vi "MCBJ_IETS_07_2021.vi"() -> ()   [LabVIEW 2016]
uses:
  sub_vi_folder/for autom measure somehowControl 2.ctl
  LUCI-10/_TypeDefs/Choose_Device_Enum.ctl
  <vilib>/Instr/_visa.llb/VISA Configure Serial Port (Instr).vi
  Instance           4 28Saved   motor control w IETS .vi
  Stanford Research 830/Stanford Research 830.lvlib
  Agilent 34401/Agilent 34401.lvlib
  Lake Shore Cryotronics 331/Lake Shore Cryotronics 331.lvlib
  Agilent 3446X Series/Agilent 3446X Series.lvlib
  <vilib>/Analysis/NI_AALBase.lvlib
  Keithley DMM6500 DAQ6500 Series/Keithley DMM6500 DAQ6500 Series.lvlib
  LUCI-10/FEMTO_LUCI-10.lvlib
panel:
  out "High R mode":bool=TRUE
  in  "lockin_once":bool
  out "LIA_all":dbl=3.282477411892588e-08
  out "# IV Curves":u16=101
  out "# O/C Cycles":u16=163
  out "LIA_conductance":dbl=3.282477414397079e-08
  out "R_Ohm_LIA1":dbl=2047762829745.1099
  out "CA gain":dbl=1e-11
  out "Femto_gain":T1(ring)=enum."10^11"
  out "Temp B in K":dbl=16.442 min=0.0 max=1645.0 step=1e-05 format="%^.5e"
  out "Temp. A in K":dbl=6.222 min=0.0 max=1645.0 step=1e-05 format="%^.5e"
  out "Bias_meas":dbl=0.028463005
  out "LIA2_DMM":dbl=0.171521931
  out "LIA1_DMM":dbl=0.0890152763
  in  "Set Lockin":bool
  in  "IETS":bool
  out "G in G0":dbl=6.3026848342087415e-09 format="%#_3g"
  out "Volt drop":dbl=0.001389956
  out "x LIA 1":dbl=0.00285722
  out "X LIA 2":dbl=-0.000922445
  out "delt MP Reached":bool
  out "Low R Mode":bool
  in  "Measurement":bool
  out "IV Active":bool
  in  "IV Sweep":bool
  in  "Stop":bool
  out "# Data Points":u32=663713
  out "R [Ohm]":dbl=2047763022414.3882 format="%#_3g"
  out "Motor Position":i32=-244174520 format="%#.3e"
  out "Reference Velocity":i16=1500
  out "Effective Velocity":i32=1499
  out "Open / Close":bool
  in  "Path Data Files":path=path "D:/MCBJ_DATA/IETS_new programm/ganz neu/S5_2021/c60/Evap_5/21_06_2021/0/322_5Hz_new_mot"
  in  "Tab":T2(tab)
  in  "Opening Velocity (High R)":i16=-1000
  in  "Closing  Velocity (High R)":i16=1500
  in  "switch Res Min [Ohm]":dbl=1000.0
  in  "reverse direction":bool
  in  "Min. R (Delta MP)  [Ohm]":dbl=4000.0
  in  "Switch by Motor Position Overrides other Switch Modes":bool
  in  "Delta Motor Position [counts]":i32=-50000000 format="%#.3e"
  in  "Opening Start Resistance [Ohm]":dbl=14906.0 format="%#.3f"
  in  "High -Low Resistance Velocity Mode":bool=TRUE
  in  "Max. Motor Position [counts]":i32=400000000 format="%#.3e"
  in  "Min. Motor Position [counts]":i32=-300000000 format="%#.3e"
  in  "Closing Velocity (Low R)":i16=1000
  in  "Opening Velocity (Low R)":i16=-2000
  in  "Use Motor":bool=TRUE
  in  "Closing Vel":i16=400
  in  "Opening opening Vel":i16=-2500
  in  "Max. Resistance [Ohm]":dbl=5000000000.0 format="%^#_6e"
  in  "Min. Resistance [Ohm]":dbl=120000.0
  in  "O/C Switch Mode":T3(radio)
  in  "Switch Res_Max. [Ohm]":dbl=100000000.0
  in  "Minimum Limit [counts]":i32=-2000000000 format="%#.3e"
  in  "Maximum Limit [counts]":i32=300000000 format="%#.3e"
  in  "Save load":u16(ring) items=["Save", "Recall"]
  in  "Setup Num":dbl=1.0
  in  "Cont Stor":bool=TRUE
  in  "Grounding":u16(ring)=1 items=["Float", "Ground"]
  in  "Sample Rate":u16(ring)=11 items=["62.5 mHz", "125 mHz", "250 mHz", "500 mHz", "1 Hz", "2 Hz", "4 Hz", "8Hz", "16 Hz", "32 Hz", "64 Hz", "128 Hz", "256 Hz", "512 Hz", "Trigger "]
  in  "In Coupling":u16(ring) items=["AC", "DC"]
  in  "Notch":u16(ring) items=["None", "Line Notch", "2x Line Notch", "Both Notch Filters"]
  in  "Input":u16(ring) items=["Single-Ended Voltage", "Differential Voltage", "1 MOhm Current Gain", "100 MOhm Current Gain"]
  in  "Ext  Trigger":u16(ring)=1 items=["Sine Zero Crossing", "TTL Rising Edge", "TTL Falling Edge"]
  in  "wait bias":u32=1
  in  "res 34401":dbl=1.0 format="%_3f"
  in  "talk 34401":bool
  in  "Line Sync":bool
  in  "rang OC (V)":dbl=2.0 format="%_3f"
  in  "Auto Range":bool=TRUE
  in  "AutoZ":bool=TRUE
  in  "Sensitivity 2":dbl=0.1
  in  "Sensitivity":dbl=0.1
  in  "LIA exp 1":dbl=1.0
  in  "LIA exp 2":dbl=100.0
  in  "Input Z":i32(ring) items=["10Mohm", "Auto"]
  in  "Av. F. Type":i32(ring)=1 items=["Repeat", "Moving"]
  in  "F. Count":u32=10
  in  "Average F.":bool
  in  "Fi. Window":dbl
  in  "AC Filter":i32(ring)=3 items=["3"=3, "20"=20, "200"=200]
  in  "Display":i32(ring) items=["Home Screen", "Home with Large Readings", "Reading Table", "Graph", "Functions Swipe", "Graph Swipe", "Secondary Swipe", "Setting Swipe", "Statistic Swipe", "User Swipe", "Channel Swipe", "Nonswitch Swipe", "Scan Swipe", "Control Channel", "Settings Channel", "Scan Channel"]
  in  "CA gain (man)":dbl=0.0001
  in  "Harm":dbl=2.0
  in  "Expand LIA1":u16(ring) items=["x1", "x10", "x100"]
  in  "Expand LIA2":u16(ring)=2 items=["x1", "x10", "x100"]
  in  "Dyn Reserve LIA1":i16(ring)=1 items=["Auto Reserve"=-1, "High Reserve"=0, "Normal"=1, "Low Noise"=2]
  in  "Dyn Reserve  LIA2":i16(ring)=1 items=["Auto Reserve"=-1, "High Reserve"=0, "Normal"=1, "Low Noise"=2]
  in  "Sensitivity LIA1":i16(ring)=23 items=["Auto Gain"=-1, "2 nV/fA"=0, "5 nV/fA"=1, "10 nV/fA"=2, "20 nV/fA"=3, "50 nV/fA"=4, "100 nV/fA"=5, "200 nV/fA"=6, "500 nV/fA"=7, "1 uV/pA"=8, "2 uV/pA"=9, "5 uV/pA"=10, "10 uV/pA"=11, "20 uV/pA"=12, "50 uV/pA"=13, "100 uV/pA"=14, "200 uV/pA"=15, "500 uV/pA"=16, "1 mV/nA"=17, "2 mV/nA"=18, "5 mV/nA"=19, "10 mV/nA"=20, "20 mV/nA"=21, "50 mV/nA"=22, "100 mV/nA"=23, "200 mV/nA"=24, "500 mV/mA"=25, "1 V/uA"=26]
  in  "Sensitivity LIA2":i16(ring)=23 items=["Auto Gain"=-1, "2 nV/fA"=0, "5 nV/fA"=1, "10 nV/fA"=2, "20 nV/fA"=3, "50 nV/fA"=4, "100 nV/fA"=5, "200 nV/fA"=6, "500 nV/fA"=7, "1 uV/pA"=8, "2 uV/pA"=9, "5 uV/pA"=10, "10 uV/pA"=11, "20 uV/pA"=12, "50 uV/pA"=13, "100 uV/pA"=14, "200 uV/pA"=15, "500 uV/pA"=16, "1 mV/nA"=17, "2 mV/nA"=18, "5 mV/nA"=19, "10 mV/nA"=20, "20 mV/nA"=21, "50 mV/nA"=22, "100 mV/nA"=23, "200 mV/nA"=24, "500 mV/mA"=25, "1 V/uA"=26]
  in  "LP_timeLIA2":u16(ring)=9 items=["10 us", "30 us", "100 us", "300 us", "1 ms", "3 ms", "10 ms", "30 ms", "100 ms", "300 ms", "1 s", "3 s", "10 s", "30 s", "100 s", "300 s", "1 ks", "3 ks", "10 ks", "30 ks"]
  in  "LP_timeLIA1":u16(ring)=9 items=["10 us", "30 us", "100 us", "300 us", "1 ms", "3 ms", "10 ms", "30 ms", "100 ms", "300 ms", "1 s", "3 s", "10 s", "30 s", "100 s", "300 s", "1 ks", "3 ks", "10 ks", "30 ks"]
  in  "LP_slope_ LIA1":u16(ring) items=["6 dB/oct", "12 dB/oct", "18 db/oct", "24 dB/oct"]
  in  "LP Slope LIA2":u16(ring) items=["6 dB/oct", "12 dB/oct", "18 db/oct", "24 dB/oct"]
  in  "Frequency":dbl=322.5
  in  "Auto Pha  LIA2":bool
  in  "Auto Phase":bool
  in  "S OutpAmpl":dbl=0.35
  in  "Man Phase LIA1":dbl
  in  "man phase LIA2":dbl=90.0
  in  "Int. Time":dbl(ring)=1.0 items=["0.001"=0.001, "0.002"=0.002, "0.006"=0.006, "0.02"=0.02, "0.06"=0.06, "0.2"=0.2, "1"=1.0, "10"=10.0, "100"=100.0]
  in  "wait points":i16=2500
  in  "Max.  [Ohm]":dbl=105000000.0 format="%^#_6e"
  in  "Min.  [Ohm]":dbl=50000.0 format="%^#_6e"
  in  "IV Delay [ms]":u16=4500
  in  "Initail V":dbl=0.3
  in  "Final V":dbl=-0.3
  in  "Set0 step":dbl=0.002 format="%#.6g"
  in  "Step (V)":dbl=0.001
  in  "Bias Voltage OC":dbl=0.1
  in  "Pre-R [Ohm]":dbl=300.0
  in  "# IV  Loops":u16=1
  in  "Use_femto":bool=TRUE
  out "Overload":bool
  in  "Bias_polarity":bool=TRUE
  in  "LIA_G":bool
  in  "Yoko_Range":T4(ring)=enum."1V"
  out "Resistance / time graph":dbl(graph)=2047763022414.3882
  out "R_Ohm_Vdrop":dbl=102.57700425624137
  out "Sample Conductance (Main)":dbl(graph)=6.3026848342087415e-09
  in  "amp_very_high_gain":dbl=0.35
  in  "?":bool
  out "no IV":bool=TRUE
  out "XY Graph   3":cluster{"x":dbl, "y":dbl}[](graph)=[{"x"=0.30282192, "y"=0.0005515354698005646}, {"x"=0.30282192, "y"=0.0005515354698005646}, {"x"=0.30282192, "y"=0.0005515354698005646}, {"x"=0.30282192, "y"=0.0005515354698005646}, {"x"=0.30282192, "y"=0.0005515354698005646}, {"x"=0.30282192, "y"=0.0005515354698005646}, {"x"=0.30282192, "y"=0.0005515354698005646}, {"x"=0.30282192, "y"=0.0005515354698005646}, {"x"=0.30282192, "y"=0.0005515354698005646}, {"x"=0.30282192, "y"=0.0005515354698005646}, {"x"=0.30282192, "y"=0.0005515354698005646}, {"x"=0.30282192, "y"=0.0005515354698005646}, {"x"=0.30282192, "y"=0.0005515354698005646}, {"x"=0.30282192, "y"=0.0005515354698005646}, {"x"=0.30282192, "y"=0.0005515354698005646}, {"x"=0.30282192, "y"=0.0005515354698005646}, {"x"=0.30282192, "y"=0.0005515354698005646}, {"x"=0.30282192, "y"=0.0005515354698005646}, {"x"=0.30282192, "y"=0.0005515354698005646}, {"x"=0.30282192, "y"=0.0005515354698005646}, {"x"=0.30282192, "y"=0.0005515354698005646}, {"x"=0.30282192, "y"=0.0005515354698005646}, {"x"=0.30282192, "y"=0.0005515354698005646}, {"x"=0.30282192, "y"=0.0005515354698005646}, {"x"=0.30282192, "y"=0.0005515354698005646}, {"x"=0.30282192, "y"=0.0005515354698005646}, {"x"=0.30282192, "y"=0.0005515354698005646}, {"x"=0.30282192, "y"=0.0005515354698005646}, {"x"=0.30282192, "y"=0.0005515354698005646}, {"x"=0.30282192, "y"=0.0005515354698005646}, {"x"=0.30282192, "y"=0.0005515354698005646}, {"x"=0.30282192, "y"=0.0005515354698005646}, {"x"=0.30282192, "y"=0.0005515354698005646}, {"x"=0.30282192, "y"=0.0005515354698005646}, {"x"=0.30282192, "y"=0.0005515354698005646}, {"x"=0.30282192, "y"=0.0005515354698005646}, {"x"=0.30282192, "y"=0.0005515354698005646}, {"x"=0.30282192, "y"=0.0005515354698005646}, {"x"=0.30282192, "y"=0.0005515354698005646}, {"x"=0.30282192, "y"=0.0005515354698005646}, {"x"=0.30282192, "y"=0.0005515354698005646}, {"x"=0.30282192, "y"=0.0005515354698005646}, {"x"=0.30282192, "y"=0.0005515354698005646}, {"x"=0.30282192, "y"=0.0005515354698005646}, {"x"=0.30282192, "y"=0.0005515354698005646}, {"x"=0.30282192, "y"=0.0005515354698005646}, {"x"=0.30282192, "y"=0.0005515354698005646}, {"x"=0.30282192, "y"=0.0005515354698005646}, {"x"=0.30282192, "y"=0.0005515354698005646}, {"x"=0.30282192, "y"=0.0005515354698005646}, {"x"=0.30282192, "y"=0.0005515354698005646}, {"x"=0.30282192, "y"=0.0005515354698005646}, {"x"=0.30282192, "y"=0.0005515354698005646}, {"x"=0.30282192, "y"=0.0005515354698005646}, {"x"=0.30282192, "y"=0.0005515354698005646}, {"x"=0.30282192, "y"=0.0005515354698005646}, {"x"=0.30282192, "y"=0.0005515354698005646}, {"x"=0.30282192, "y"=0.0005515354698005646}, {"x"=0.30282192, "y"=0.0005515354698005646}, {"x"=0.30282192, "y"=0.0005515354698005646}, {"x"=0.30282192, "y"=0.0005515354698005646}, {"x"=0.30282192, "y"=0.0005515354698005646}, {"x"=0.30282192, "y"=0.0005515354698005646}, {"x"=0.30282192, "y"=0.0005515354698005646}, {"x"=0.30282192, "y"=0.0005515354698005646}, {"x"=0.30282192, "y"=0.0005515354698005646}, {"x"=0.30282192, "y"=0.0005515354698005646}, {"x"=0.30282192, "y"=0.0005515354698005646}, {"x"=0.30282192, "y"=0.0005515354698005646}, {"x"=0.30282192, "y"=0.0005515354698005646}, {"x"=0.30282192, "y"=0.0005515354698005646}, {"x"=0.30282192, "y"=0.0005515354698005646}, {"x"=0.30282192, "y"=0.0005515354698005646}, {"x"=0.30282192, "y"=0.0005515354698005646}, {"x"=0.30282192, "y"=0.0005515354698005646}, {"x"=0.30282192, "y"=0.0005515354698005646}, {"x"=0.30282192, "y"=0.0005515354698005646}, {"x"=0.30282192, "y"=0.0005515354698005646}, {"x"=0.30282192, "y"=0.0005515354698005646}, {"x"=0.30282192, "y"=0.0005515354698005646}, {"x"=0.30282192, "y"=0.0005515354698005646}, {"x"=0.30282192, "y"=0.0005515354698005646}, {"x"=0.30282192, "y"=0.0005515354698005646}, {"x"=0.30282192, "y"=0.0005515354698005646}, {"x"=0.30282192, "y"=0.0005515354698005646}, {"x"=0.30282192, "y"=0.0005515354698005646}, {"x"=0.30282192, "y"=0.0005515354698005646}, {"x"=0.30282192, "y"=0.0005515354698005646}, {"x"=0.30282192, "y"=0.0005515354698005646}, {"x"=0.30282192, "y"=0.0005515354698005646}, {"x"=0.30282192, "y"=0.0005515354698005646}, {"x"=0.30282192, "y"=0.0005515354698005646}, {"x"=0.30282192, "y"=0.0005515354698005646}, {"x"=0.30282192, "y"=0.0005515354698005646}, {"x"=0.30282192, "y"=0.0005515354698005646}, {"x"=0.30282192, "y"=0.0005515354698005646}, {"x"=0.30282192, "y"=0.0005515354698005646}, {"x"=0.30282192, "y"=0.0005515354698005646}, {"x"=0.30282192, "y"=0.0005515354698005646}, {"x"=0.30282192, "y"=0.0005515354698005646}, {"x"=0.30282192, "y"=0.0005515354698005646}, {"x"=0.30282192, "y"=0.0005515354698005646}, {"x"=0.30282192, "y"=0.0005515354698005646}, {"x"=0.30282192, "y"=0.0005515354698005646}, {"x"=0.30282192, "y"=0.0005515354698005646}, {"x"=0.30282192, "y"=0.0005515354698005646}, {"x"=0.30282192, "y"=0.0005515354698005646}, {"x"=0.30282192, "y"=0.0005515354698005646}, {"x"=0.30282192, "y"=0.0005515354698005646}, {"x"=0.30282192, "y"=0.0005515354698005646}, {"x"=0.30282192, "y"=0.0005515354698005646}, {"x"=0.30282192, "y"=0.0005515354698005646}, {"x"=0.30282192, "y"=0.0005515354698005646}, {"x"=0.30282192, "y"=0.0005515354698005646}, {"x"=0.30282192, "y"=0.0005515354698005646}, {"x"=0.30282192, "y"=0.0005515354698005646}, {"x"=0.30282192, "y"=0.0005515354698005646}, {"x"=0.30282192, "y"=0.0005515354698005646}, {"x"=0.30282192, "y"=0.0005515354698005646}, {"x"=0.30282192, "y"=0.0005515354698005646}, {"x"=0.30282192, "y"=0.0005515354698005646}, {"x"=0.30282192, "y"=0.0005515354698005646}, {"x"=0.30282192, "y"=0.0005515354698005646}, {"x"=0.30282192, "y"=0.0005515354698005646}, {"x"=0.30282192, "y"=0.0005515354698005646}, {"x"=0.30282192, "y"=0.0005515354698005646}, {"x"=0.30282192, "y"=0.0005515354698005646}, {"x"=0.30282192, "y"=0.0005515354698005646}, {"x"=0.30282192, "y"=0.0005515354698005646}, {"x"=0.30282192, "y"=0.0005515354698005646}, {"x"=0.30282192, "y"=0.0005515354698005646}, {"x"=0.30282192, "y"=0.0005515354698005646}, {"x"=0.30282192, "y"=0.0005515354698005646}, {"x"=0.30282192, "y"=0.0005515354698005646}, {"x"=0.30282192, "y"=0.0005515354698005646}, {"x"=0.30282192, "y"=0.0005515354698005646}, {"x"=0.30282192, "y"=0.0005515354698005646}, {"x"=0.30282192, "y"=0.0005515354698005646}, {"x"=0.30282192, "y"=0.0005515354698005646}, {"x"=0.30282192, "y"=0.0005515354698005646}, {"x"=0.30282192, "y"=0.0005515354698005646}, {"x"=0.30282192, "y"=0.0005515354698005646}, {"x"=0.30282192, "y"=0.0005515354698005646}, {"x"=0.30282192, "y"=0.0005515354698005646}, {"x"=0.30282192, "y"=0.0005515354698005646}, {"x"=0.30282192, "y"=0.0005515354698005646}, {"x"=0.30282192, "y"=0.0005515354698005646}, {"x"=0.30282192, "y"=0.0005515354698005646}, {"x"=0.30282192, "y"=0.0005515354698005646}, {"x"=0.30282192, "y"=0.0005515354698005646}, {"x"=0.30282192, "y"=0.0005515354698005646}, {"x"=0.30282192, "y"=0.0005515354698005646}, {"x"=0.30282192, "y"=0.0005515354698005646}, {"x"=0.30282192, "y"=0.0005515354698005646}, {"x"=0.30282192, "y"=0.0005515354698005646}, {"x"=0.30282192, "y"=0.0005515354698005646}, {"x"=0.30282192, "y"=0.0005515354698005646}, {"x"=0.30282192, "y"=0.0005515354698005646}, {"x"=0.30282192, "y"=0.0005515354698005646}, {"x"=0.30282192, "y"=0.0005515354698005646}, {"x"=0.30282192, "y"=0.0005515354698005646}, {"x"=0.30282192, "y"=0.0005515354698005646}, {"x"=0.30282192, "y"=0.0005515354698005646}, {"x"=0.30282192, "y"=0.0005515354698005646}, {"x"=0.30282192, "y"=0.0005515354698005646}, {"x"=0.30282192, "y"=0.0005515354698005646}, {"x"=0.30282192, "y"=0.0005515354698005646}, {"x"=0.30282192, "y"=0.0005515354698005646}, {"x"=0.30282192, "y"=0.0005515354698005646}, {"x"=0.30282192, "y"=0.0005515354698005646}, {"x"=0.30282192, "y"=0.0005515354698005646}, {"x"=0.30282192, "y"=0.0005515354698005646}, {"x"=0.30282192, "y"=0.0005515354698005646}, {"x"=0.30282192, "y"=0.0005515354698005646}, {"x"=0.30282192, "y"=0.0005515354698005646}, {"x"=0.30282192, "y"=0.0005515354698005646}, {"x"=0.30282192, "y"=0.0005515354698005646}, {"x"=0.30282192, "y"=0.0005515354698005646}, {"x"=0.30282192, "y"=0.0005515354698005646}, {"x"=0.30282192, "y"=0.0005515354698005646}, {"x"=0.30282192, "y"=0.0005515354698005646}, {"x"=0.30282192, "y"=0.0005515354698005646}, {"x"=0.30282192, "y"=0.0005515354698005646}, {"x"=0.30282192, "y"=0.0005515354698005646}, {"x"=0.30282192, "y"=0.0005515354698005646}, {"x"=0.30282192, "y"=0.0005515354698005646}, {"x"=0.30282192, "y"=0.0005515354698005646}, {"x"=0.30282192, "y"=0.0005515354698005646}, {"x"=0.30282192, "y"=0.0005515354698005646}, {"x"=0.30282192, "y"=0.0005515354698005646}, {"x"=0.30282192, "y"=0.0005515354698005646}, {"x"=0.30282192, "y"=0.0005515354698005646}, {"x"=0.30282192, "y"=0.0005515354698005646}, {"x"=0.30282192, "y"=0.0005515354698005646}, {"x"=0.30282192, "y"=0.0005515354698005646}, {"x"=0.30282192, "y"=0.0005515354698005646}, {"x"=0.30282192, "y"=0.0005515354698005646}, {"x"=0.30282192, "y"=0.0005515354698005646}, {"x"=0.30282192, "y"=0.0005515354698005646}, {"x"=0.30282192, "y"=0.0005515354698005646}, {"x"=0.30282192, "y"=0.0005515354698005646}, {"x"=0.30282192, "y"=0.0005515354698005646}, {"x"=0.30282192, "y"=0.0005515354698005646}, {"x"=0.30282192, "y"=0.0005515354698005646}, {"x"=0.30282192, "y"=0.0005515354698005646}, {"x"=0.30282192, "y"=0.0005515354698005646}, {"x"=0.30282192, "y"=0.0005515354698005646}, {"x"=0.30282192, "y"=0.0005515354698005646}, {"x"=0.30282192, "y"=0.0005515354698005646}, {"x"=0.30282192, "y"=0.0005515354698005646}, {"x"=0.30282192, "y"=0.0005515354698005646}, {"x"=0.30282192, "y"=0.0005515354698005646}, {"x"=0.30282192, "y"=0.0005515354698005646}, {"x"=0.30282192, "y"=0.0005515354698005646}, {"x"=0.30282192, "y"=0.0005515354698005646}, {"x"=0.30282192, "y"=0.0005515354698005646}, {"x"=0.30282192, "y"=0.0005515354698005646}, {"x"=0.30282192, "y"=0.0005515354698005646}, {"x"=0.30282192, "y"=0.0005515354698005646}, {"x"=0.30282192, "y"=0.0005515354698005646}, {"x"=0.30282192, "y"=0.0005515354698005646}, {"x"=0.30282192, "y"=0.0005515354698005646}, {"x"=0.30282192, "y"=0.0005515354698005646}, {"x"=0.30282192, "y"=0.0005515354698005646}, {"x"=0.30282192, "y"=0.0005515354698005646}, {"x"=0.30282192, "y"=0.0005515354698005646}, {"x"=0.30282192, "y"=0.0005515354698005646}, {"x"=0.30282192, "y"=0.0005515354698005646}, {"x"=0.30282192, "y"=0.0005515354698005646}, {"x"=0.30282192, "y"=0.0005515354698005646}, {"x"=0.30282192, "y"=0.0005515354698005646}, {"x"=0.30282192, "y"=0.0005515354698005646}, {"x"=0.30282192, "y"=0.0005515354698005646}, {"x"=0.30282192, "y"=0.0005515354698005646}, {"x"=0.30282192, "y"=0.0005515354698005646}, {"x"=0.30282192, "y"=0.0005515354698005646}, {"x"=0.30282192, "y"=0.0005515354698005646}, {"x"=0.30282192, "y"=0.0005515354698005646}, {"x"=0.30282192, "y"=0.0005515354698005646}, {"x"=0.30282192, "y"=0.0005515354698005646}, {"x"=0.30282192, "y"=0.0005515354698005646}, {"x"=0.30282192, "y"=0.0005515354698005646}, {"x"=0.30282192, "y"=0.0005515354698005646}, {"x"=0.30282192, "y"=0.0005515354698005646}, {"x"=0.30282192, "y"=0.0005515354698005646}, {"x"=0.30282192, "y"=0.0005515354698005646}, {"x"=0.30282192, "y"=0.0005515354698005646}, {"x"=0.30282192, "y"=0.0005515354698005646}, {"x"=0.30282192, "y"=0.0005515354698005646}, {"x"=0.30282192, "y"=0.0005515354698005646}, {"x"=0.30282192, "y"=0.0005515354698005646}, {"x"=0.30282192, "y"=0.0005515354698005646}, {"x"=0.30282192, "y"=0.0005515354698005646}, {"x"=0.30282192, "y"=0.0005515354698005646}, {"x"=0.30282192, "y"=0.0005515354698005646}, {"x"=0.30282192, "y"=0.0005515354698005646}, {"x"=0.30282192, "y"=0.0005515354698005646}, {"x"=0.30282192, "y"=0.0005515354698005646}, {"x"=0.30282192, "y"=0.0005515354698005646}, {"x"=0.30282192, "y"=0.0005515354698005646}, {"x"=0.30282192, "y"=0.0005515354698005646}, {"x"=0.30282192, "y"=0.0005515354698005646}, {"x"=0.30282192, "y"=0.0005515354698005646}, {"x"=0.30282192, "y"=0.0005515354698005646}, {"x"=0.30282192, "y"=0.0005515354698005646}, {"x"=0.30282192, "y"=0.0005515354698005646}, {"x"=0.30282192, "y"=0.0005515354698005646}, {"x"=0.30282192, "y"=0.0005515354698005646}, {"x"=0.30282192, "y"=0.0005515354698005646}, {"x"=0.30282192, "y"=0.0005515354698005646}, {"x"=0.30282192, "y"=0.0005515354698005646}, {"x"=0.30282192, "y"=0.0005515354698005646}, {"x"=0.30282192, "y"=0.0005515354698005646}, {"x"=0.30282192, "y"=0.0005515354698005646}, {"x"=0.30282192, "y"=0.0005515354698005646}, {"x"=0.30282192, "y"=0.0005515354698005646}, {"x"=0.30282192, "y"=0.0005515354698005646}, {"x"=0.30282192, "y"=0.0005515354698005646}, {"x"=0.30282192, "y"=0.0005515354698005646}, {"x"=0.30282192, "y"=0.0005515354698005646}, {"x"=0.30282192, "y"=0.0005515354698005646}, {"x"=0.30282192, "y"=0.0005515354698005646}, {"x"=0.30282192, "y"=0.0005515354698005646}, {"x"=0.30282192, "y"=0.0005515354698005646}, {"x"=0.30282192, "y"=0.0005515354698005646}, {"x"=0.30282192, "y"=0.0005515354698005646}, {"x"=0.30282192, "y"=0.0005515354698005646}, {"x"=0.30282192, "y"=0.0005515354698005646}, {"x"=0.30282192, "y"=0.0005515354698005646}, {"x"=0.30282192, "y"=0.0005515354698005646}, {"x"=0.30282192, "y"=0.0005515354698005646}, {"x"=0.30282192, "y"=0.0005515354698005646}, {"x"=0.30282192, "y"=0.0005515354698005646}, {"x"=0.30282192, "y"=0.0005515354698005646}, {"x"=0.30282192, "y"=0.0005515354698005646}, {"x"=0.30282192, "y"=0.0005515354698005646}, {"x"=0.30282192, "y"=0.0005515354698005646}, {"x"=0.30282192, "y"=0.0005515354698005646}, {"x"=0.30282192, "y"=0.0005515354698005646}, {"x"=0.30282192, "y"=0.0005515354698005646}, {"x"=0.30282192, "y"=0.0005515354698005646}, {"x"=0.30282192, "y"=0.0005515354698005646}, {"x"=0.30282192, "y"=0.0005515354698005646}, {"x"=0.30282192, "y"=0.0005515354698005646}, {"x"=0.30282192, "y"=0.0005515354698005646}, {"x"=0.30282192, "y"=0.0005515354698005646}, {"x"=0.30282192, "y"=0.0005515354698005646}, {"x"=0.30282192, "y"=0.0005515354698005646}, {"x"=0.30282192, "y"=0.0005515354698005646}, {"x"=0.30282192, "y"=0.0005515354698005646}, {"x"=0.30282192, "y"=0.0005515354698005646}, {"x"=0.30282192, "y"=0.0005515354698005646}, {"x"=0.30282192, "y"=0.0005515354698005646}, {"x"=0.30282192, "y"=0.0005515354698005646}, {"x"=0.30282192, "y"=0.0005515354698005646}, {"x"=0.30282192, "y"=0.0005515354698005646}, {"x"=0.30282192, "y"=0.0005515354698005646}, {"x"=0.30282192, "y"=0.0005515354698005646}, {"x"=0.30282192, "y"=0.0005515354698005646}, {"x"=0.30282192, "y"=0.0005515354698005646}, {"x"=0.30282192, "y"=0.0005515354698005646}, {"x"=0.30282192, "y"=0.0005515354698005646}, {"x"=0.30282192, "y"=0.0005515354698005646}, {"x"=0.30282192, "y"=0.0005515354698005646}, {"x"=0.30282192, "y"=0.0005515354698005646}, {"x"=0.30282192, "y"=0.0005515354698005646}, {"x"=0.30282192, "y"=0.0005515354698005646}, {"x"=0.30282192, "y"=0.0005515354698005646}, {"x"=0.30282192, "y"=0.0005515354698005646}, {"x"=0.30282192, "y"=0.0005515354698005646}, {"x"=0.30282192, "y"=0.0005515354698005646}, {"x"=0.30282192, "y"=0.0005515354698005646}, {"x"=0.30282192, "y"=0.0005515354698005646}, {"x"=0.30282192, "y"=0.0005515354698005646}, {"x"=0.30282192, "y"=0.0005515354698005646}, {"x"=0.30282192, "y"=0.0005515354698005646}, {"x"=0.30282192, "y"=0.0005515354698005646}, {"x"=0.30282192, "y"=0.0005515354698005646}, {"x"=0.30282192, "y"=0.0005515354698005646}, {"x"=0.30282192, "y"=0.0005515354698005646}, {"x"=0.30282192, "y"=0.0005515354698005646}, {"x"=0.30282192, "y"=0.0005515354698005646}, {"x"=0.30282192, "y"=0.0005515354698005646}, {"x"=0.30282192, "y"=0.0005515354698005646}, {"x"=0.30282192, "y"=0.0005515354698005646}, {"x"=0.30282192, "y"=0.0005515354698005646}, {"x"=0.30282192, "y"=0.0005515354698005646}, {"x"=0.30282192, "y"=0.0005515354698005646}, {"x"=0.30282192, "y"=0.0005515354698005646}, {"x"=0.30282192, "y"=0.0005515354698005646}, {"x"=0.30282192, "y"=0.0005515354698005646}, {"x"=0.30282192, "y"=0.0005515354698005646}, {"x"=0.30282192, "y"=0.0005515354698005646}, {"x"=0.30282192, "y"=0.0005515354698005646}, {"x"=0.30282192, "y"=0.0005515354698005646}, {"x"=0.30282192, "y"=0.0005515354698005646}, {"x"=0.30282192, "y"=0.0005515354698005646}, {"x"=0.30282192, "y"=0.0005515354698005646}, {"x"=0.30282192, "y"=0.0005515354698005646}, {"x"=0.30282192, "y"=0.0005515354698005646}, {"x"=0.30282192, "y"=0.0005515354698005646}, {"x"=0.30282192, "y"=0.0005515354698005646}, {"x"=0.30282192, "y"=0.0005515354698005646}, {"x"=0.30282192, "y"=0.0005515354698005646}, {"x"=0.30282192, "y"=0.0005515354698005646}, {"x"=0.30282192, "y"=0.0005515354698005646}, {"x"=0.30282192, "y"=0.0005515354698005646}, {"x"=0.30282192, "y"=0.0005515354698005646}, {"x"=0.30282192, "y"=0.0005515354698005646}, {"x"=0.30282192, "y"=0.0005515354698005646}, {"x"=0.30282192, "y"=0.0005515354698005646}, {"x"=0.30282192, "y"=0.0005515354698005646}, {"x"=0.30282192, "y"=0.0005515354698005646}, {"x"=0.30282192, "y"=0.0005515354698005646}, {"x"=0.30282192, "y"=0.0005515354698005646}, {"x"=0.30282192, "y"=0.0005515354698005646}, {"x"=0.30282192, "y"=0.0005515354698005646}, {"x"=0.30282192, "y"=0.0005515354698005646}, {"x"=0.30282192, "y"=0.0005515354698005646}, {"x"=0.30282192, "y"=0.0005515354698005646}, {"x"=0.30282192, "y"=0.0005515354698005646}, {"x"=0.30282192, "y"=0.0005515354698005646}, {"x"=0.30282192, "y"=0.0005515354698005646}, {"x"=0.30282192, "y"=0.0005515354698005646}, {"x"=0.30282192, "y"=0.0005515354698005646}, {"x"=0.30282192, "y"=0.0005515354698005646}, {"x"=0.30282192, "y"=0.0005515354698005646}, {"x"=0.30282192, "y"=0.0005515354698005646}, {"x"=0.30282192, "y"=0.0005515354698005646}, {"x"=0.30282192, "y"=0.0005515354698005646}, {"x"=0.30282192, "y"=0.0005515354698005646}, {"x"=0.30282192, "y"=0.0005515354698005646}, {"x"=0.30282192, "y"=0.0005515354698005646}, {"x"=0.30282192, "y"=0.0005515354698005646}, {"x"=0.30282192, "y"=0.0005515354698005646}, {"x"=0.30282192, "y"=0.0005515354698005646}, {"x"=0.30282192, "y"=0.0005515354698005646}, {"x"=0.30282192, "y"=0.0005515354698005646}, {"x"=0.30282192, "y"=0.0005515354698005646}, {"x"=0.30282192, "y"=0.0005515354698005646}, {"x"=0.30282192, "y"=0.0005515354698005646}, {"x"=0.30282192, "y"=0.0005515354698005646}, {"x"=0.30282192, "y"=0.0005515354698005646}, {"x"=0.30282192, "y"=0.0005515354698005646}, {"x"=0.30282192, "y"=0.0005515354698005646}, {"x"=0.30282192, "y"=0.0005515354698005646}, {"x"=0.30282192, "y"=0.0005515354698005646}, {"x"=0.30282192, "y"=0.0005515354698005646}, {"x"=0.30282192, "y"=0.0005515354698005646}, {"x"=0.30282192, "y"=0.0005515354698005646}, {"x"=0.30282192, "y"=0.0005515354698005646}, {"x"=0.30282192, "y"=0.0005515354698005646}, {"x"=0.30282192, "y"=0.0005515354698005646}, {"x"=0.30282192, "y"=0.0005515354698005646}, {"x"=0.30282192, "y"=0.0005515354698005646}, {"x"=0.30282192, "y"=0.0005515354698005646}, {"x"=0.30282192, "y"=0.0005515354698005646}, {"x"=0.30282192, "y"=0.0005515354698005646}, {"x"=0.30282192, "y"=0.0005515354698005646}, {"x"=0.30282192, "y"=0.0005515354698005646}, {"x"=0.30282192, "y"=0.0005515354698005646}, {"x"=0.30282192, "y"=0.0005515354698005646}, {"x"=0.30282192, "y"=0.0005515354698005646}, {"x"=0.30282192, "y"=0.0005515354698005646}, {"x"=0.30282192, "y"=0.0005515354698005646}, {"x"=0.30282192, "y"=0.0005515354698005646}, {"x"=0.30282192, "y"=0.0005515354698005646}, {"x"=0.30282192, "y"=0.0005515354698005646}, {"x"=0.30282192, "y"=0.0005515354698005646}, {"x"=0.30282192, "y"=0.0005515354698005646}, {"x"=0.30282192, "y"=0.0005515354698005646}, {"x"=0.30282192, "y"=0.0005515354698005646}, {"x"=0.30282192, "y"=0.0005515354698005646}, {"x"=0.30282192, "y"=0.0005515354698005646}, {"x"=0.30282192, "y"=0.0005515354698005646}, {"x"=0.30282192, "y"=0.0005515354698005646}, {"x"=0.30282192, "y"=0.0005515354698005646}, {"x"=0.30282192, "y"=0.0005515354698005646}, {"x"=0.30282192, "y"=0.0005515354698005646}, {"x"=0.30282192, "y"=0.0005515354698005646}, {"x"=0.30282192, "y"=0.0005515354698005646}, {"x"=0.30282192, "y"=0.0005515354698005646}, {"x"=0.30282192, "y"=0.0005515354698005646}, {"x"=0.30282192, "y"=0.0005515354698005646}, {"x"=0.30282192, "y"=0.0005515354698005646}, {"x"=0.30282192, "y"=0.0005515354698005646}, {"x"=0.30282192, "y"=0.0005515354698005646}, {"x"=0.30282192, "y"=0.0005515354698005646}, {"x"=0.30282192, "y"=0.0005515354698005646}, {"x"=0.30282192, "y"=0.0005515354698005646}, {"x"=0.30282192, "y"=0.0005515354698005646}, {"x"=0.30282192, "y"=0.0005515354698005646}, {"x"=0.30282192, "y"=0.0005515354698005646}, {"x"=0.30282192, "y"=0.0005515354698005646}, {"x"=0.30282192, "y"=0.0005515354698005646}, {"x"=0.30282192, "y"=0.0005515354698005646}, {"x"=0.30282192, "y"=0.0005515354698005646}, {"x"=0.30282192, "y"=0.0005515354698005646}, {"x"=0.30282192, "y"=0.0005515354698005646}, {"x"=0.30282192, "y"=0.0005515354698005646}, {"x"=0.30282192, "y"=0.0005515354698005646}, {"x"=0.30282192, "y"=0.0005515354698005646}, {"x"=0.30282192, "y"=0.0005515354698005646}, {"x"=0.30282192, "y"=0.0005515354698005646}, {"x"=0.30282192, "y"=0.0005515354698005646}, {"x"=0.30282192, "y"=0.0005515354698005646}, {"x"=0.30282192, "y"=0.0005515354698005646}, {"x"=0.30282192, "y"=0.0005515354698005646}, {"x"=0.30282192, "y"=0.0005515354698005646}, {"x"=0.30282192, "y"=0.0005515354698005646}, {"x"=0.30282192, "y"=0.0005515354698005646}, {"x"=0.30282192, "y"=0.0005515354698005646}, {"x"=0.30282192, "y"=0.0005515354698005646}, {"x"=0.30282192, "y"=0.0005515354698005646}, {"x"=0.30282192, "y"=0.0005515354698005646}, {"x"=0.30282192, "y"=0.0005515354698005646}, {"x"=0.30282192, "y"=0.0005515354698005646}, {"x"=0.30282192, "y"=0.0005515354698005646}, {"x"=0.30282192, "y"=0.0005515354698005646}, {"x"=0.30282192, "y"=0.0005515354698005646}, {"x"=0.30282192, "y"=0.0005515354698005646}, {"x"=0.30282192, "y"=0.0005515354698005646}, {"x"=0.30282192, "y"=0.0005515354698005646}, {"x"=0.30282192, "y"=0.0005515354698005646}, {"x"=0.30282192, "y"=0.0005515354698005646}, {"x"=0.30282192, "y"=0.0005515354698005646}, {"x"=0.30282192, "y"=0.0005515354698005646}, {"x"=0.30282192, "y"=0.0005515354698005646}, {"x"=0.30282192, "y"=0.0005515354698005646}, {"x"=0.30282192, "y"=0.0005515354698005646}, {"x"=0.30282192, "y"=0.0005515354698005646}, {"x"=0.30282192, "y"=0.0005515354698005646}, {"x"=0.30282192, "y"=0.0005515354698005646}, {"x"=0.30282192, "y"=0.0005515354698005646}, {"x"=0.30282192, "y"=0.0005515354698005646}, {"x"=0.30282192, "y"=0.0005515354698005646}, {"x"=0.30282192, "y"=0.0005515354698005646}, {"x"=0.30282192, "y"=0.0005515354698005646}, {"x"=0.30282192, "y"=0.0005515354698005646}, {"x"=0.30282192, "y"=0.0005515354698005646}, {"x"=0.30282192, "y"=0.0005515354698005646}, {"x"=0.30282192, "y"=0.0005515354698005646}, {"x"=0.30282192, "y"=0.0005515354698005646}, {"x"=0.30282192, "y"=0.0005515354698005646}, {"x"=0.30282192, "y"=0.0005515354698005646}, {"x"=0.30282192, "y"=0.0005515354698005646}, {"x"=0.30282192, "y"=0.0005515354698005646}, {"x"=0.30282192, "y"=0.0005515354698005646}, {"x"=0.30282192, "y"=0.0005515354698005646}, {"x"=0.30282192, "y"=0.0005515354698005646}, {"x"=0.30282192, "y"=0.0005515354698005646}, {"x"=0.30282192, "y"=0.0005515354698005646}, {"x"=0.30282192, "y"=0.0005515354698005646}, {"x"=0.30282192, "y"=0.0005515354698005646}, {"x"=0.30282192, "y"=0.0005515354698005646}, {"x"=0.30282192, "y"=0.0005515354698005646}, {"x"=0.30282192, "y"=0.0005515354698005646}, {"x"=0.30282192, "y"=0.0005515354698005646}, {"x"=0.30282192, "y"=0.0005515354698005646}, {"x"=0.30282192, "y"=0.0005515354698005646}, {"x"=0.30282192, "y"=0.0005515354698005646}, {"x"=0.30282192, "y"=0.0005515354698005646}, {"x"=0.30282192, "y"=0.0005515354698005646}, {"x"=0.30282192, "y"=0.0005515354698005646}, {"x"=0.30282192, "y"=0.0005515354698005646}, {"x"=0.30282192, "y"=0.0005515354698005646}, {"x"=0.30282192, "y"=0.0005515354698005646}, {"x"=0.30282192, "y"=0.0005515354698005646}, {"x"=0.30282192, "y"=0.0005515354698005646}, {"x"=0.30282192, "y"=0.0005515354698005646}, {"x"=0.30282192, "y"=0.0005515354698005646}, {"x"=0.30282192, "y"=0.0005515354698005646}, {"x"=0.30282192, "y"=0.0005515354698005646}, {"x"=0.30282192, "y"=0.0005515354698005646}, {"x"=0.30282192, "y"=0.0005515354698005646}, {"x"=0.30282192, "y"=0.0005515354698005646}, {"x"=0.30282192, "y"=0.0005515354698005646}, {"x"=0.30282192, "y"=0.0005515354698005646}, {"x"=0.30282192, "y"=0.0005515354698005646}, {"x"=0.30282192, "y"=0.0005515354698005646}, {"x"=0.30282192, "y"=0.0005515354698005646}, {"x"=0.30282192, "y"=0.0005515354698005646}, {"x"=0.30282192, "y"=0.0005515354698005646}, {"x"=0.30282192, "y"=0.0005515354698005646}, {"x"=0.30282192, "y"=0.0005515354698005646}, {"x"=0.30282192, "y"=0.0005515354698005646}, {"x"=0.30282192, "y"=0.0005515354698005646}, {"x"=0.30282192, "y"=0.0005515354698005646}, {"x"=0.30282192, "y"=0.0005515354698005646}, {"x"=0.30282192, "y"=0.0005515354698005646}, {"x"=0.30282192, "y"=0.0005515354698005646}, {"x"=0.30282192, "y"=0.0005515354698005646}, {"x"=0.30282192, "y"=0.0005515354698005646}, {"x"=0.30282192, "y"=0.0005515354698005646}, {"x"=0.30282192, "y"=0.0005515354698005646}, {"x"=0.30282192, "y"=0.0005515354698005646}, {"x"=0.30282192, "y"=0.0005515354698005646}, {"x"=0.30282192, "y"=0.0005515354698005646}, {"x"=0.30282192, "y"=0.0005515354698005646}, {"x"=0.30282192, "y"=0.0005515354698005646}, {"x"=0.30282192, "y"=0.0005515354698005646}, {"x"=0.30282192, "y"=0.0005515354698005646}, {"x"=0.30282192, "y"=0.0005515354698005646}, {"x"=0.30282192, "y"=0.0005515354698005646}, {"x"=0.30282192, "y"=0.0005515354698005646}, {"x"=0.30282192, "y"=0.0005515354698005646}, {"x"=0.30282192, "y"=0.0005515354698005646}, {"x"=0.30282192, "y"=0.0005515354698005646}, {"x"=0.30282192, "y"=0.0005515354698005646}, {"x"=0.30282192, "y"=0.0005515354698005646}, {"x"=0.30282192, "y"=0.0005515354698005646}, {"x"=0.30282192, "y"=0.0005515354698005646}, {"x"=0.30282192, "y"=0.0005515354698005646}, {"x"=0.30282192, "y"=0.0005515354698005646}, {"x"=0.30282192, "y"=0.0005515354698005646}, {"x"=0.30282192, "y"=0.0005515354698005646}, {"x"=0.30282192, "y"=0.0005515354698005646}, {"x"=0.30282192, "y"=0.0005515354698005646}, {"x"=0.30282192, "y"=0.0005515354698005646}, {"x"=0.30282192, "y"=0.0005515354698005646}, {"x"=0.30282192, "y"=0.0005515354698005646}, {"x"=0.30282192, "y"=0.0005515354698005646}, {"x"=0.30282192, "y"=0.0005515354698005646}, {"x"=0.30282192, "y"=0.0005515354698005646}, {"x"=0.30282192, "y"=0.0005515354698005646}, {"x"=0.30282192, "y"=0.0005515354698005646}, {"x"=0.30282192, "y"=0.0005515354698005646}, {"x"=0.30282192, "y"=0.0005515354698005646}, {"x"=0.30282192, "y"=0.0005515354698005646}, {"x"=0.30282192, "y"=0.0005515354698005646}, {"x"=0.30282192, "y"=0.0005515354698005646}, {"x"=0.30282192, "y"=0.0005515354698005646}, {"x"=0.30282192, "y"=0.0005515354698005646}, {"x"=0.30282192, "y"=0.0005515354698005646}, {"x"=0.30282192, "y"=0.0005515354698005646}, {"x"=0.30282192, "y"=0.0005515354698005646}, {"x"=0.30282192, "y"=0.0005515354698005646}, {"x"=0.30282192, "y"=0.0005515354698005646}, {"x"=0.30282192, "y"=0.0005515354698005646}, {"x"=0.30282192, "y"=0.0005515354698005646}, {"x"=0.30282192, "y"=0.0005515354698005646}, {"x"=0.30282192, "y"=0.0005515354698005646}, {"x"=0.30282192, "y"=0.0005515354698005646}, {"x"=0.30282192, "y"=0.0005515354698005646}, {"x"=0.30282192, "y"=0.0005515354698005646}, {"x"=0.30282192, "y"=0.0005515354698005646}, {"x"=0.30282192, "y"=0.0005515354698005646}, {"x"=0.30282192, "y"=0.0005515354698005646}, {"x"=0.30282192, "y"=0.0005515354698005646}, {"x"=0.30282192, "y"=0.0005515354698005646}, {"x"=0.30282192, "y"=0.0005515354698005646}, {"x"=0.30282192, "y"=0.0005515354698005646}, {"x"=0.30282192, "y"=0.0005515354698005646}, {"x"=0.30282192, "y"=0.0005515354698005646}, {"x"=0.30282192, "y"=0.0005515354698005646}, {"x"=0.30282192, "y"=0.0005515354698005646}, {"x"=0.30282192, "y"=0.0005515354698005646}, {"x"=0.30282192, "y"=0.0005515354698005646}, {"x"=0.30282192, "y"=0.0005515354698005646}, {"x"=0.30282192, "y"=0.0005515354698005646}, {"x"=0.30282192, "y"=0.0005515354698005646}, {"x"=0.30282192, "y"=0.0005515354698005646}, {"x"=0.30282192, "y"=0.0005515354698005646}, {"x"=0.30282192, "y"=0.0005515354698005646}, {"x"=0.30282192, "y"=0.0005515354698005646}, {"x"=0.30282192, "y"=0.0005515354698005646}, {"x"=0.30282192, "y"=0.0005515354698005646}, {"x"=0.30282192, "y"=0.0005515354698005646}, {"x"=0.30282192, "y"=0.0005515354698005646}, {"x"=0.30282192, "y"=0.0005515354698005646}, {"x"=0.30282192, "y"=0.0005515354698005646}, {"x"=0.30282192, "y"=0.0005515354698005646}, {"x"=0.30282192, "y"=0.0005515354698005646}, {"x"=0.30282192, "y"=0.0005515354698005646}, {"x"=0.30282192, "y"=0.0005515354698005646}, {"x"=0.30282192, "y"=0.0005515354698005646}, {"x"=0.30282192, "y"=0.0005515354698005646}, {"x"=0.30282192, "y"=0.0005515354698005646}, {"x"=0.30282192, "y"=0.0005515354698005646}, {"x"=0.30282192, "y"=0.0005515354698005646}, {"x"=0.30282192, "y"=0.0005515354698005646}, {"x"=0.30282192, "y"=0.0005515354698005646}, {"x"=0.30282192, "y"=0.0005515354698005646}, {"x"=0.30282192, "y"=0.0005515354698005646}, {"x"=0.30282192, "y"=0.0005515354698005646}, {"x"=0.30282192, "y"=0.0005515354698005646}, {"x"=0.30282192, "y"=0.0005515354698005646}, {"x"=0.30282192, "y"=0.0005515354698005646}, {"x"=0.30282192, "y"=0.0005515354698005646}, {"x"=0.30282192, "y"=0.0005515354698005646}, {"x"=0.30282192, "y"=0.0005515354698005646}, {"x"=0.30282192, "y"=0.0005515354698005646}, {"x"=0.30282192, "y"=0.0005515354698005646}, {"x"=0.30282192, "y"=0.0005515354698005646}, {"x"=0.30282192, "y"=0.0005515354698005646}, {"x"=0.30282192, "y"=0.0005515354698005646}, {"x"=0.30282192, "y"=0.0005515354698005646}, {"x"=0.30282192, "y"=0.0005515354698005646}, {"x"=0.30282192, "y"=0.0005515354698005646}, {"x"=0.30282192, "y"=0.0005515354698005646}, {"x"=0.30282192, "y"=0.0005515354698005646}, {"x"=0.30282192, "y"=0.0005515354698005646}, {"x"=0.30282192, "y"=0.0005515354698005646}, {"x"=0.30282192, "y"=0.0005515354698005646}, {"x"=0.30282192, "y"=0.0005515354698005646}, {"x"=0.30282192, "y"=0.0005515354698005646}, {"x"=0.30282192, "y"=0.0005515354698005646}, {"x"=0.30282192, "y"=0.0005515354698005646}, {"x"=0.30282192, "y"=0.0005515354698005646}, {"x"=0.30282192, "y"=0.0005515354698005646}, {"x"=0.30282192, "y"=0.0005515354698005646}, {"x"=0.30282192, "y"=0.0005515354698005646}, {"x"=0.30282192, "y"=0.0005515354698005646}, {"x"=0.30282192, "y"=0.0005515354698005646}, {"x"=0.30282192, "y"=0.0005515354698005646}, {"x"=0.30282192, "y"=0.0005515354698005646}, {"x"=0.30282192, "y"=0.0005515354698005646}, {"x"=0.30282192, "y"=0.0005515354698005646}, {"x"=0.30282192, "y"=0.0005515354698005646}, {"x"=0.30282192, "y"=0.0005515354698005646}, {"x"=0.30282192, "y"=0.0005515354698005646}, {"x"=0.30282192, "y"=0.0005515354698005646}, {"x"=0.30282192, "y"=0.0005515354698005646}, {"x"=0.30282192, "y"=0.0005515354698005646}, {"x"=0.30282192, "y"=0.0005515354698005646}, {"x"=0.30282192, "y"=0.0005515354698005646}, {"x"=0.30282192, "y"=0.0005515354698005646}, {"x"=0.30282192, "y"=0.0005515354698005646}, {"x"=0.30282192, "y"=0.0005515354698005646}, {"x"=0.30282192, "y"=0.0005515354698005646}, {"x"=0.30282192, "y"=0.0005515354698005646}, {"x"=0.30282192, "y"=0.0005515354698005646}, {"x"=0.30282192, "y"=0.0005515354698005646}, {"x"=0.30282192, "y"=0.0005515354698005646}, {"x"=0.30282192, "y"=0.0005515354698005646}, {"x"=0.30282192, "y"=0.0005515354698005646}, {"x"=0.30282192, "y"=0.0005515354698005646}, {"x"=0.30282192, "y"=0.0005515354698005646}, {"x"=0.30282192, "y"=0.0005515354698005646}, {"x"=0.30282192, "y"=0.0005515354698005646}, {"x"=0.30282192, "y"=0.0005515354698005646}, {"x"=0.30282192, "y"=0.0005515354698005646}, {"x"=0.30282192, "y"=0.0005515354698005646}, {"x"=0.30282192, "y"=0.0005515354698005646}, {"x"=0.30282192, "y"=0.0005515354698005646}, {"x"=0.30282192, "y"=0.0005515354698005646}, {"x"=0.30282192, "y"=0.0005515354698005646}, {"x"=0.30282192, "y"=0.0005515354698005646}, {"x"=0.30282192, "y"=0.0005515354698005646}, {"x"=0.30282192, "y"=0.0005515354698005646}, {"x"=0.30282192, "y"=0.0005515354698005646}, {"x"=0.30282192, "y"=0.0005515354698005646}, {"x"=0.30282192, "y"=0.0005515354698005646}, {"x"=0.30282192, "y"=0.0005515354698005646}, {"x"=0.30282192, "y"=0.0005515354698005646}, {"x"=0.30282192, "y"=0.0005515354698005646}, {"x"=0.30282192, "y"=0.0005515354698005646}, {"x"=0.30282192, "y"=0.0005515354698005646}, {"x"=0.30282192, "y"=0.0005515354698005646}, {"x"=0.30282192, "y"=0.0005515354698005646}, {"x"=0.30282192, "y"=0.0005515354698005646}, {"x"=0.30282192, "y"=0.0005515354698005646}, {"x"=0.30282192, "y"=0.0005515354698005646}, {"x"=0.30282192, "y"=0.0005515354698005646}, {"x"=0.30282192, "y"=0.0005515354698005646}, {"x"=0.30282192, "y"=0.0005515354698005646}, {"x"=0.30282192, "y"=0.0005515354698005646}, {"x"=0.30282192, "y"=0.0005515354698005646}, {"x"=0.30282192, "y"=0.0005515354698005646}, {"x"=0.30282192, "y"=0.0005515354698005646}, {"x"=0.30282192, "y"=0.0005515354698005646}, {"x"=0.30282192, "y"=0.0005515354698005646}, {"x"=0.30282192, "y"=0.0005515354698005646}, {"x"=0.30282192, "y"=0.0005515354698005646}, {"x"=0.30282192, "y"=0.0005515354698005646}, {"x"=0.30282192, "y"=0.0005515354698005646}, {"x"=0.30282192, "y"=0.0005515354698005646}, {"x"=0.30282192, "y"=0.0005515354698005646}, {"x"=0.30282192, "y"=0.0005515354698005646}, {"x"=0.30282192, "y"=0.0005515354698005646}, {"x"=0.30282192, "y"=0.0005515354698005646}, {"x"=0.30282192, "y"=0.0005515354698005646}, {"x"=0.30282192, "y"=0.0005515354698005646}, {"x"=0.30282192, "y"=0.0005515354698005646}, {"x"=0.30282192, "y"=0.0005515354698005646}, {"x"=0.30282192, "y"=0.0005515354698005646}, {"x"=0.30282192, "y"=0.0005515354698005646}, {"x"=0.30282192, "y"=0.0005515354698005646}, {"x"=0.30282192, "y"=0.0005515354698005646}, {"x"=0.30282192, "y"=0.0005515354698005646}, {"x"=0.30282192, "y"=0.0005515354698005646}, {"x"=0.30282192, "y"=0.0005515354698005646}, {"x"=0.30282192, "y"=0.0005515354698005646}, {"x"=0.30282192, "y"=0.0005515354698005646}, {"x"=0.30282192, "y"=0.0005515354698005646}, {"x"=0.30282192, "y"=0.0005515354698005646}, {"x"=0.30282192, "y"=0.0005515354698005646}, {"x"=0.30282192, "y"=0.0005515354698005646}, {"x"=0.30282192, "y"=0.0005515354698005646}, {"x"=0.30282192, "y"=0.0005515354698005646}, {"x"=0.30282192, "y"=0.0005515354698005646}, {"x"=0.30282192, "y"=0.0005515354698005646}, {"x"=0.30282192, "y"=0.0005515354698005646}, {"x"=0.30282192, "y"=0.0005515354698005646}, {"x"=0.30282192, "y"=0.0005515354698005646}, {"x"=0.30282192, "y"=0.0005515354698005646}, {"x"=0.30282192, "y"=0.0005515354698005646}, {"x"=0.30282192, "y"=0.0005515354698005646}, {"x"=0.30282192, "y"=0.0005515354698005646}, {"x"=0.30282192, "y"=0.0005515354698005646}, {"x"=0.30282192, "y"=0.0005515354698005646}, {"x"=0.30282192, "y"=0.0005515354698005646}, {"x"=0.30282192, "y"=0.0005515354698005646}, {"x"=0.30282192, "y"=0.0005515354698005646}, {"x"=0.30282192, "y"=0.0005515354698005646}, {"x"=0.30282192, "y"=0.0005515354698005646}, {"x"=0.30282192, "y"=0.0005515354698005646}, {"x"=0.30282192, "y"=0.0005515354698005646}, {"x"=0.30282192, "y"=0.0005515354698005646}, {"x"=0.30282192, "y"=0.0005515354698005646}, {"x"=0.30282192, "y"=0.0005515354698005646}, {"x"=0.30282192, "y"=0.0005515354698005646}, {"x"=0.30282192, "y"=0.0005515354698005646}, {"x"=0.30282192, "y"=0.0005515354698005646}, {"x"=0.30282192, "y"=0.0005515354698005646}, {"x"=0.30282192, "y"=0.0005515354698005646}, {"x"=0.30282192, "y"=0.0005515354698005646}, {"x"=0.30282192, "y"=0.0005515354698005646}, {"x"=0.30282192, "y"=0.0005515354698005646}, {"x"=0.30282192, "y"=0.0005515354698005646}, {"x"=0.30282192, "y"=0.0005515354698005646}, {"x"=0.30282192, "y"=0.0005515354698005646}, {"x"=0.30282192, "y"=0.0005515354698005646}, {"x"=0.30282192, "y"=0.0005515354698005646}, {"x"=0.30282192, "y"=0.0005515354698005646}, {"x"=0.30282192, "y"=0.0005515354698005646}, {"x"=0.30282192, "y"=0.0005515354698005646}, {"x"=0.30282192, "y"=0.0005515354698005646}, {"x"=0.30282192, "y"=0.0005515354698005646}, {"x"=0.30282192, "y"=0.0005515354698005646}, {"x"=0.30282192, "y"=0.0005515354698005646}, {"x"=0.30282192, "y"=0.0005515354698005646}, {"x"=0.30282192, "y"=0.0005515354698005646}, {"x"=0.30282192, "y"=0.0005515354698005646}, {"x"=0.30282192, "y"=0.0005515354698005646}, {"x"=0.30282192, "y"=0.0005515354698005646}, {"x"=0.30282192, "y"=0.0005515354698005646}, {"x"=0.30282192, "y"=0.0005515354698005646}, {"x"=0.30282192, "y"=0.0005515354698005646}, {"x"=0.30282192, "y"=0.0005515354698005646}, {"x"=0.30282192, "y"=0.0005515354698005646}, {"x"=0.30282192, "y"=0.0005515354698005646}, {"x"=0.30282192, "y"=0.0005515354698005646}, {"x"=0.30282192, "y"=0.0005515354698005646}, {"x"=0.30282192, "y"=0.0005515354698005646}, {"x"=0.30282192, "y"=0.0005515354698005646}, {"x"=0.30282192, "y"=0.0005515354698005646}, {"x"=0.30282192, "y"=0.0005515354698005646}, {"x"=0.30282192, "y"=0.0005515354698005646}, {"x"=0.30282192, "y"=0.0005515354698005646}, {"x"=0.30282192, "y"=0.0005515354698005646}, {"x"=0.30282192, "y"=0.0005515354698005646}, {"x"=0.30282192, "y"=0.0005515354698005646}, {"x"=0.30282192, "y"=0.0005515354698005646}, {"x"=0.30282192, "y"=0.0005515354698005646}, {"x"=0.30282192, "y"=0.0005515354698005646}, {"x"=0.30282192, "y"=0.0005515354698005646}, {"x"=0.30282192, "y"=0.0005515354698005646}, {"x"=0.30282192, "y"=0.0005515354698005646}, {"x"=0.30282192, "y"=0.0005515354698005646}, {"x"=0.30282192, "y"=0.0005515354698005646}, {"x"=0.30282192, "y"=0.0005515354698005646}, {"x"=0.30282192, "y"=0.0005515354698005646}, {"x"=0.30282192, "y"=0.0005515354698005646}, {"x"=0.30282192, "y"=0.0005515354698005646}, {"x"=0.30282192, "y"=0.0005515354698005646}, {"x"=0.30282192, "y"=0.0005515354698005646}, {"x"=0.30282192, "y"=0.0005515354698005646}, {"x"=0.30282192, "y"=0.0005515354698005646}, {"x"=0.30282192, "y"=0.0005515354698005646}, {"x"=0.30282192, "y"=0.0005515354698005646}, {"x"=0.30282192, "y"=0.0005515354698005646}, {"x"=0.30282192, "y"=0.0005515354698005646}, {"x"=0.30282192, "y"=0.0005515354698005646}, {"x"=0.30282192, "y"=0.0005515354698005646}, {"x"=0.30282192, "y"=0.0005515354698005646}, {"x"=0.30282192, "y"=0.0005515354698005646}, {"x"=0.30282192, "y"=0.0005515354698005646}, {"x"=0.30282192, "y"=0.0005515354698005646}, {"x"=0.30282192, "y"=0.0005515354698005646}, {"x"=0.30282192, "y"=0.0005515354698005646}, {"x"=0.30282192, "y"=0.0005515354698005646}, {"x"=0.30282192, "y"=0.0005515354698005646}, {"x"=0.30282192, "y"=0.0005515354698005646}, {"x"=0.30282192, "y"=0.0005515354698005646}, {"x"=0.30282192, "y"=0.0005515354698005646}, {"x"=0.30282192, "y"=0.0005515354698005646}, {"x"=0.30282192, "y"=0.0005515354698005646}, {"x"=0.30282192, "y"=0.0005515354698005646}, {"x"=0.30282192, "y"=0.0005515354698005646}, {"x"=0.30282192, "y"=0.0005515354698005646}, {"x"=0.30282192, "y"=0.0005515354698005646}, {"x"=0.30282192, "y"=0.0005515354698005646}, {"x"=0.30282192, "y"=0.0005515354698005646}, {"x"=0.30282192, "y"=0.0005515354698005646}, {"x"=0.30282192, "y"=0.0005515354698005646}, {"x"=0.30282192, "y"=0.0005515354698005646}, {"x"=0.30282192, "y"=0.0005515354698005646}, {"x"=0.30282192, "y"=0.0005515354698005646}, {"x"=0.30282192, "y"=0.0005515354698005646}, {"x"=0.30282192, "y"=0.0005515354698005646}, {"x"=0.30282192, "y"=0.0005515354698005646}, {"x"=0.30282192, "y"=0.0005515354698005646}, {"x"=0.30282192, "y"=0.0005515354698005646}, {"x"=0.30282192, "y"=0.0005515354698005646}, {"x"=0.30282192, "y"=0.0005515354698005646}, {"x"=0.30282192, "y"=0.0005515354698005646}, {"x"=0.30282192, "y"=0.0005515354698005646}, {"x"=0.30282192, "y"=0.0005515354698005646}, {"x"=0.30282192, "y"=0.0005515354698005646}, {"x"=0.30282192, "y"=0.0005515354698005646}, {"x"=0.30282192, "y"=0.0005515354698005646}, {"x"=0.30282192, "y"=0.0005515354698005646}, {"x"=0.30282192, "y"=0.0005515354698005646}, {"x"=0.30282192, "y"=0.0005515354698005646}, {"x"=0.30282192, "y"=0.0005515354698005646}, {"x"=0.30282192, "y"=0.0005515354698005646}, {"x"=0.30282192, "y"=0.0005515354698005646}, {"x"=0.30282192, "y"=0.0005515354698005646}, {"x"=0.30282192, "y"=0.0005515354698005646}, {"x"=0.30282192, "y"=0.0005515354698005646}, {"x"=0.30282192, "y"=0.0005515354698005646}, {"x"=0.30282192, "y"=0.0005515354698005646}, {"x"=0.30282192, "y"=0.0005515354698005646}, {"x"=0.30282192, "y"=0.0005515354698005646}, {"x"=0.30282192, "y"=0.0005515354698005646}, {"x"=0.30282192, "y"=0.0005515354698005646}, {"x"=0.30282192, "y"=0.0005515354698005646}, {"x"=0.30282192, "y"=0.0005515354698005646}, {"x"=0.30282192, "y"=0.0005515354698005646}, {"x"=0.30282192, "y"=0.0005515354698005646}, {"x"=0.30282192, "y"=0.0005515354698005646}, {"x"=0.30282192, "y"=0.0005515354698005646}, {"x"=0.30282192, "y"=0.0005515354698005646}, {"x"=0.30282192, "y"=0.0005515354698005646}, {"x"=0.30282192, "y"=0.0005515354698005646}, {"x"=0.30282192, "y"=0.0005515354698005646}, {"x"=0.30282192, "y"=0.0005515354698005646}, {"x"=0.30282192, "y"=0.0005515354698005646}, {"x"=0.30282192, "y"=0.0005515354698005646}, {"x"=0.30282192, "y"=0.0005515354698005646}, {"x"=0.30282192, "y"=0.0005515354698005646}, {"x"=0.30282192, "y"=0.0005515354698005646}, {"x"=0.30282192, "y"=0.0005515354698005646}, {"x"=0.30282192, "y"=0.0005515354698005646}, {"x"=0.30282192, "y"=0.0005515354698005646}, {"x"=0.30282192, "y"=0.0005515354698005646}, {"x"=0.30282192, "y"=0.0005515354698005646}, {"x"=0.30282192, "y"=0.0005515354698005646}, {"x"=0.30282192, "y"=0.0005515354698005646}, {"x"=0.30282192, "y"=0.0005515354698005646}, {"x"=0.30282192, "y"=0.0005515354698005646}, {"x"=0.30282192, "y"=0.0005515354698005646}, {"x"=0.30282192, "y"=0.0005515354698005646}, {"x"=0.30282192, "y"=0.0005515354698005646}, {"x"=0.30282192, "y"=0.0005515354698005646}, {"x"=0.30282192, "y"=0.0005515354698005646}, {"x"=0.30282192, "y"=0.0005515354698005646}, {"x"=0.30282192, "y"=0.0005515354698005646}, {"x"=0.30282192, "y"=0.0005515354698005646}, {"x"=0.30282192, "y"=0.0005515354698005646}, {"x"=0.30282192, "y"=0.0005515354698005646}, {"x"=0.30282192, "y"=0.0005515354698005646}, {"x"=0.30282192, "y"=0.0005515354698005646}, {"x"=0.30282192, "y"=0.0005515354698005646}, {"x"=0.30282192, "y"=0.0005515354698005646}, {"x"=0.30282192, "y"=0.0005515354698005646}, {"x"=0.30282192, "y"=0.0005515354698005646}, {"x"=0.30282192, "y"=0.0005515354698005646}, {"x"=0.30282192, "y"=0.0005515354698005646}, {"x"=0.30282192, "y"=0.0005515354698005646}, {"x"=0.30282192, "y"=0.0005515354698005646}, {"x"=0.30282192, "y"=0.0005515354698005646}, {"x"=0.30282192, "y"=0.0005515354698005646}, {"x"=0.30282192, "y"=0.0005515354698005646}, {"x"=0.30282192, "y"=0.0005515354698005646}, {"x"=0.30282192, "y"=0.0005515354698005646}, {"x"=0.30282192, "y"=0.0005515354698005646}, {"x"=0.30282192, "y"=0.0005515354698005646}, {"x"=0.30282192, "y"=0.0005515354698005646}]
  out "XY Graph   4":cluster{"x":dbl, "y":dbl}[](graph)=[{"x"=0.30282192, "y"=0.012730640556902548}, {"x"=0.30282192, "y"=0.012730640556902548}, {"x"=0.30282192, "y"=0.012730640556902548}, {"x"=0.30282192, "y"=0.012730640556902548}, {"x"=0.30282192, "y"=0.012730640556902548}, {"x"=0.30282192, "y"=0.012730640556902548}, {"x"=0.30282192, "y"=0.012730640556902548}, {"x"=0.30282192, "y"=0.012730640556902548}, {"x"=0.30282192, "y"=0.012730640556902548}, {"x"=0.30282192, "y"=0.012730640556902548}, {"x"=0.30282192, "y"=0.012730640556902548}, {"x"=0.30282192, "y"=0.012730640556902548}, {"x"=0.30282192, "y"=0.012730640556902548}, {"x"=0.30282192, "y"=0.012730640556902548}, {"x"=0.30282192, "y"=0.012730640556902548}, {"x"=0.30282192, "y"=0.012730640556902548}, {"x"=0.30282192, "y"=0.012730640556902548}, {"x"=0.30282192, "y"=0.012730640556902548}, {"x"=0.30282192, "y"=0.012730640556902548}, {"x"=0.30282192, "y"=0.012730640556902548}, {"x"=0.30282192, "y"=0.012730640556902548}, {"x"=0.30282192, "y"=0.012730640556902548}, {"x"=0.30282192, "y"=0.012730640556902548}, {"x"=0.30282192, "y"=0.012730640556902548}, {"x"=0.30282192, "y"=0.012730640556902548}, {"x"=0.30282192, "y"=0.012730640556902548}, {"x"=0.30282192, "y"=0.012730640556902548}, {"x"=0.30282192, "y"=0.012730640556902548}, {"x"=0.30282192, "y"=0.012730640556902548}, {"x"=0.30282192, "y"=0.012730640556902548}, {"x"=0.30282192, "y"=0.012730640556902548}, {"x"=0.30282192, "y"=0.012730640556902548}, {"x"=0.30282192, "y"=0.012730640556902548}, {"x"=0.30282192, "y"=0.012730640556902548}, {"x"=0.30282192, "y"=0.012730640556902548}, {"x"=0.30282192, "y"=0.012730640556902548}, {"x"=0.30282192, "y"=0.012730640556902548}, {"x"=0.30282192, "y"=0.012730640556902548}, {"x"=0.30282192, "y"=0.012730640556902548}, {"x"=0.30282192, "y"=0.012730640556902548}, {"x"=0.30282192, "y"=0.012730640556902548}, {"x"=0.30282192, "y"=0.012730640556902548}, {"x"=0.30282192, "y"=0.012730640556902548}, {"x"=0.30282192, "y"=0.012730640556902548}, {"x"=0.30282192, "y"=0.012730640556902548}, {"x"=0.30282192, "y"=0.012730640556902548}, {"x"=0.30282192, "y"=0.012730640556902548}, {"x"=0.30282192, "y"=0.012730640556902548}, {"x"=0.30282192, "y"=0.012730640556902548}, {"x"=0.30282192, "y"=0.012730640556902548}, {"x"=0.30282192, "y"=0.012730640556902548}, {"x"=0.30282192, "y"=0.012730640556902548}, {"x"=0.30282192, "y"=0.012730640556902548}, {"x"=0.30282192, "y"=0.012730640556902548}, {"x"=0.30282192, "y"=0.012730640556902548}, {"x"=0.30282192, "y"=0.012730640556902548}, {"x"=0.30282192, "y"=0.012730640556902548}, {"x"=0.30282192, "y"=0.012730640556902548}, {"x"=0.30282192, "y"=0.012730640556902548}, {"x"=0.30282192, "y"=0.012730640556902548}, {"x"=0.30282192, "y"=0.012730640556902548}, {"x"=0.30282192, "y"=0.012730640556902548}, {"x"=0.30282192, "y"=0.012730640556902548}, {"x"=0.30282192, "y"=0.012730640556902548}, {"x"=0.30282192, "y"=0.012730640556902548}, {"x"=0.30282192, "y"=0.012730640556902548}, {"x"=0.30282192, "y"=0.012730640556902548}, {"x"=0.30282192, "y"=0.012730640556902548}, {"x"=0.30282192, "y"=0.012730640556902548}, {"x"=0.30282192, "y"=0.012730640556902548}, {"x"=0.30282192, "y"=0.012730640556902548}, {"x"=0.30282192, "y"=0.012730640556902548}, {"x"=0.30282192, "y"=0.012730640556902548}, {"x"=0.30282192, "y"=0.012730640556902548}, {"x"=0.30282192, "y"=0.012730640556902548}, {"x"=0.30282192, "y"=0.012730640556902548}, {"x"=0.30282192, "y"=0.012730640556902548}, {"x"=0.30282192, "y"=0.012730640556902548}, {"x"=0.30282192, "y"=0.012730640556902548}, {"x"=0.30282192, "y"=0.012730640556902548}, {"x"=0.30282192, "y"=0.012730640556902548}, {"x"=0.30282192, "y"=0.012730640556902548}, {"x"=0.30282192, "y"=0.012730640556902548}, {"x"=0.30282192, "y"=0.012730640556902548}, {"x"=0.30282192, "y"=0.012730640556902548}, {"x"=0.30282192, "y"=0.012730640556902548}, {"x"=0.30282192, "y"=0.012730640556902548}, {"x"=0.30282192, "y"=0.012730640556902548}, {"x"=0.30282192, "y"=0.012730640556902548}, {"x"=0.30282192, "y"=0.012730640556902548}, {"x"=0.30282192, "y"=0.012730640556902548}, {"x"=0.30282192, "y"=0.012730640556902548}, {"x"=0.30282192, "y"=0.012730640556902548}, {"x"=0.30282192, "y"=0.012730640556902548}, {"x"=0.30282192, "y"=0.012730640556902548}, {"x"=0.30282192, "y"=0.012730640556902548}, {"x"=0.30282192, "y"=0.012730640556902548}, {"x"=0.30282192, "y"=0.012730640556902548}, {"x"=0.30282192, "y"=0.012730640556902548}, {"x"=0.30282192, "y"=0.012730640556902548}, {"x"=0.30282192, "y"=0.012730640556902548}, {"x"=0.30282192, "y"=0.012730640556902548}, {"x"=0.30282192, "y"=0.012730640556902548}, {"x"=0.30282192, "y"=0.012730640556902548}, {"x"=0.30282192, "y"=0.012730640556902548}, {"x"=0.30282192, "y"=0.012730640556902548}, {"x"=0.30282192, "y"=0.012730640556902548}, {"x"=0.30282192, "y"=0.012730640556902548}, {"x"=0.30282192, "y"=0.012730640556902548}, {"x"=0.30282192, "y"=0.012730640556902548}, {"x"=0.30282192, "y"=0.012730640556902548}, {"x"=0.30282192, "y"=0.012730640556902548}, {"x"=0.30282192, "y"=0.012730640556902548}, {"x"=0.30282192, "y"=0.012730640556902548}, {"x"=0.30282192, "y"=0.012730640556902548}, {"x"=0.30282192, "y"=0.012730640556902548}, {"x"=0.30282192, "y"=0.012730640556902548}, {"x"=0.30282192, "y"=0.012730640556902548}, {"x"=0.30282192, "y"=0.012730640556902548}, {"x"=0.30282192, "y"=0.012730640556902548}, {"x"=0.30282192, "y"=0.012730640556902548}, {"x"=0.30282192, "y"=0.012730640556902548}, {"x"=0.30282192, "y"=0.012730640556902548}, {"x"=0.30282192, "y"=0.012730640556902548}, {"x"=0.30282192, "y"=0.012730640556902548}, {"x"=0.30282192, "y"=0.012730640556902548}, {"x"=0.30282192, "y"=0.012730640556902548}, {"x"=0.30282192, "y"=0.012730640556902548}, {"x"=0.30282192, "y"=0.012730640556902548}, {"x"=0.30282192, "y"=0.012730640556902548}, {"x"=0.30282192, "y"=0.012730640556902548}, {"x"=0.30282192, "y"=0.012730640556902548}, {"x"=0.30282192, "y"=0.012730640556902548}, {"x"=0.30282192, "y"=0.012730640556902548}, {"x"=0.30282192, "y"=0.012730640556902548}, {"x"=0.30282192, "y"=0.012730640556902548}, {"x"=0.30282192, "y"=0.012730640556902548}, {"x"=0.30282192, "y"=0.012730640556902548}, {"x"=0.30282192, "y"=0.012730640556902548}, {"x"=0.30282192, "y"=0.012730640556902548}, {"x"=0.30282192, "y"=0.012730640556902548}, {"x"=0.30282192, "y"=0.012730640556902548}, {"x"=0.30282192, "y"=0.012730640556902548}, {"x"=0.30282192, "y"=0.012730640556902548}, {"x"=0.30282192, "y"=0.012730640556902548}, {"x"=0.30282192, "y"=0.012730640556902548}, {"x"=0.30282192, "y"=0.012730640556902548}, {"x"=0.30282192, "y"=0.012730640556902548}, {"x"=0.30282192, "y"=0.012730640556902548}, {"x"=0.30282192, "y"=0.012730640556902548}, {"x"=0.30282192, "y"=0.012730640556902548}, {"x"=0.30282192, "y"=0.012730640556902548}, {"x"=0.30282192, "y"=0.012730640556902548}, {"x"=0.30282192, "y"=0.012730640556902548}, {"x"=0.30282192, "y"=0.012730640556902548}, {"x"=0.30282192, "y"=0.012730640556902548}, {"x"=0.30282192, "y"=0.012730640556902548}, {"x"=0.30282192, "y"=0.012730640556902548}, {"x"=0.30282192, "y"=0.012730640556902548}, {"x"=0.30282192, "y"=0.012730640556902548}, {"x"=0.30282192, "y"=0.012730640556902548}, {"x"=0.30282192, "y"=0.012730640556902548}, {"x"=0.30282192, "y"=0.012730640556902548}, {"x"=0.30282192, "y"=0.012730640556902548}, {"x"=0.30282192, "y"=0.012730640556902548}, {"x"=0.30282192, "y"=0.012730640556902548}, {"x"=0.30282192, "y"=0.012730640556902548}, {"x"=0.30282192, "y"=0.012730640556902548}, {"x"=0.30282192, "y"=0.012730640556902548}, {"x"=0.30282192, "y"=0.012730640556902548}, {"x"=0.30282192, "y"=0.012730640556902548}, {"x"=0.30282192, "y"=0.012730640556902548}, {"x"=0.30282192, "y"=0.012730640556902548}, {"x"=0.30282192, "y"=0.012730640556902548}, {"x"=0.30282192, "y"=0.012730640556902548}, {"x"=0.30282192, "y"=0.012730640556902548}, {"x"=0.30282192, "y"=0.012730640556902548}, {"x"=0.30282192, "y"=0.012730640556902548}, {"x"=0.30282192, "y"=0.012730640556902548}, {"x"=0.30282192, "y"=0.012730640556902548}, {"x"=0.30282192, "y"=0.012730640556902548}, {"x"=0.30282192, "y"=0.012730640556902548}, {"x"=0.30282192, "y"=0.012730640556902548}, {"x"=0.30282192, "y"=0.012730640556902548}, {"x"=0.30282192, "y"=0.012730640556902548}, {"x"=0.30282192, "y"=0.012730640556902548}, {"x"=0.30282192, "y"=0.012730640556902548}, {"x"=0.30282192, "y"=0.012730640556902548}, {"x"=0.30282192, "y"=0.012730640556902548}, {"x"=0.30282192, "y"=0.012730640556902548}, {"x"=0.30282192, "y"=0.012730640556902548}, {"x"=0.30282192, "y"=0.012730640556902548}, {"x"=0.30282192, "y"=0.012730640556902548}, {"x"=0.30282192, "y"=0.012730640556902548}, {"x"=0.30282192, "y"=0.012730640556902548}, {"x"=0.30282192, "y"=0.012730640556902548}, {"x"=0.30282192, "y"=0.012730640556902548}, {"x"=0.30282192, "y"=0.012730640556902548}, {"x"=0.30282192, "y"=0.012730640556902548}, {"x"=0.30282192, "y"=0.012730640556902548}, {"x"=0.30282192, "y"=0.012730640556902548}, {"x"=0.30282192, "y"=0.012730640556902548}, {"x"=0.30282192, "y"=0.012730640556902548}, {"x"=0.30282192, "y"=0.012730640556902548}, {"x"=0.30282192, "y"=0.012730640556902548}, {"x"=0.30282192, "y"=0.012730640556902548}, {"x"=0.30282192, "y"=0.012730640556902548}, {"x"=0.30282192, "y"=0.012730640556902548}, {"x"=0.30282192, "y"=0.012730640556902548}, {"x"=0.30282192, "y"=0.012730640556902548}, {"x"=0.30282192, "y"=0.012730640556902548}, {"x"=0.30282192, "y"=0.012730640556902548}, {"x"=0.30282192, "y"=0.012730640556902548}, {"x"=0.30282192, "y"=0.012730640556902548}, {"x"=0.30282192, "y"=0.012730640556902548}, {"x"=0.30282192, "y"=0.012730640556902548}, {"x"=0.30282192, "y"=0.012730640556902548}, {"x"=0.30282192, "y"=0.012730640556902548}, {"x"=0.30282192, "y"=0.012730640556902548}, {"x"=0.30282192, "y"=0.012730640556902548}, {"x"=0.30282192, "y"=0.012730640556902548}, {"x"=0.30282192, "y"=0.012730640556902548}, {"x"=0.30282192, "y"=0.012730640556902548}, {"x"=0.30282192, "y"=0.012730640556902548}, {"x"=0.30282192, "y"=0.012730640556902548}, {"x"=0.30282192, "y"=0.012730640556902548}, {"x"=0.30282192, "y"=0.012730640556902548}, {"x"=0.30282192, "y"=0.012730640556902548}, {"x"=0.30282192, "y"=0.012730640556902548}, {"x"=0.30282192, "y"=0.012730640556902548}, {"x"=0.30282192, "y"=0.012730640556902548}, {"x"=0.30282192, "y"=0.012730640556902548}, {"x"=0.30282192, "y"=0.012730640556902548}, {"x"=0.30282192, "y"=0.012730640556902548}, {"x"=0.30282192, "y"=0.012730640556902548}, {"x"=0.30282192, "y"=0.012730640556902548}, {"x"=0.30282192, "y"=0.012730640556902548}, {"x"=0.30282192, "y"=0.012730640556902548}, {"x"=0.30282192, "y"=0.012730640556902548}, {"x"=0.30282192, "y"=0.012730640556902548}, {"x"=0.30282192, "y"=0.012730640556902548}, {"x"=0.30282192, "y"=0.012730640556902548}, {"x"=0.30282192, "y"=0.012730640556902548}, {"x"=0.30282192, "y"=0.012730640556902548}, {"x"=0.30282192, "y"=0.012730640556902548}, {"x"=0.30282192, "y"=0.012730640556902548}, {"x"=0.30282192, "y"=0.012730640556902548}, {"x"=0.30282192, "y"=0.012730640556902548}, {"x"=0.30282192, "y"=0.012730640556902548}, {"x"=0.30282192, "y"=0.012730640556902548}, {"x"=0.30282192, "y"=0.012730640556902548}, {"x"=0.30282192, "y"=0.012730640556902548}, {"x"=0.30282192, "y"=0.012730640556902548}, {"x"=0.30282192, "y"=0.012730640556902548}, {"x"=0.30282192, "y"=0.012730640556902548}, {"x"=0.30282192, "y"=0.012730640556902548}, {"x"=0.30282192, "y"=0.012730640556902548}, {"x"=0.30282192, "y"=0.012730640556902548}, {"x"=0.30282192, "y"=0.012730640556902548}, {"x"=0.30282192, "y"=0.012730640556902548}, {"x"=0.30282192, "y"=0.012730640556902548}, {"x"=0.30282192, "y"=0.012730640556902548}, {"x"=0.30282192, "y"=0.012730640556902548}, {"x"=0.30282192, "y"=0.012730640556902548}, {"x"=0.30282192, "y"=0.012730640556902548}, {"x"=0.30282192, "y"=0.012730640556902548}, {"x"=0.30282192, "y"=0.012730640556902548}, {"x"=0.30282192, "y"=0.012730640556902548}, {"x"=0.30282192, "y"=0.012730640556902548}, {"x"=0.30282192, "y"=0.012730640556902548}, {"x"=0.30282192, "y"=0.012730640556902548}, {"x"=0.30282192, "y"=0.012730640556902548}, {"x"=0.30282192, "y"=0.012730640556902548}, {"x"=0.30282192, "y"=0.012730640556902548}, {"x"=0.30282192, "y"=0.012730640556902548}, {"x"=0.30282192, "y"=0.012730640556902548}, {"x"=0.30282192, "y"=0.012730640556902548}, {"x"=0.30282192, "y"=0.012730640556902548}, {"x"=0.30282192, "y"=0.012730640556902548}, {"x"=0.30282192, "y"=0.012730640556902548}, {"x"=0.30282192, "y"=0.012730640556902548}, {"x"=0.30282192, "y"=0.012730640556902548}, {"x"=0.30282192, "y"=0.012730640556902548}, {"x"=0.30282192, "y"=0.012730640556902548}, {"x"=0.30282192, "y"=0.012730640556902548}, {"x"=0.30282192, "y"=0.012730640556902548}, {"x"=0.30282192, "y"=0.012730640556902548}, {"x"=0.30282192, "y"=0.012730640556902548}, {"x"=0.30282192, "y"=0.012730640556902548}, {"x"=0.30282192, "y"=0.012730640556902548}, {"x"=0.30282192, "y"=0.012730640556902548}, {"x"=0.30282192, "y"=0.012730640556902548}, {"x"=0.30282192, "y"=0.012730640556902548}, {"x"=0.30282192, "y"=0.012730640556902548}, {"x"=0.30282192, "y"=0.012730640556902548}, {"x"=0.30282192, "y"=0.012730640556902548}, {"x"=0.30282192, "y"=0.012730640556902548}, {"x"=0.30282192, "y"=0.012730640556902548}, {"x"=0.30282192, "y"=0.012730640556902548}, {"x"=0.30282192, "y"=0.012730640556902548}, {"x"=0.30282192, "y"=0.012730640556902548}, {"x"=0.30282192, "y"=0.012730640556902548}, {"x"=0.30282192, "y"=0.012730640556902548}, {"x"=0.30282192, "y"=0.012730640556902548}, {"x"=0.30282192, "y"=0.012730640556902548}, {"x"=0.30282192, "y"=0.012730640556902548}, {"x"=0.30282192, "y"=0.012730640556902548}, {"x"=0.30282192, "y"=0.012730640556902548}, {"x"=0.30282192, "y"=0.012730640556902548}, {"x"=0.30282192, "y"=0.012730640556902548}, {"x"=0.30282192, "y"=0.012730640556902548}, {"x"=0.30282192, "y"=0.012730640556902548}, {"x"=0.30282192, "y"=0.012730640556902548}, {"x"=0.30282192, "y"=0.012730640556902548}, {"x"=0.30282192, "y"=0.012730640556902548}, {"x"=0.30282192, "y"=0.012730640556902548}, {"x"=0.30282192, "y"=0.012730640556902548}, {"x"=0.30282192, "y"=0.012730640556902548}, {"x"=0.30282192, "y"=0.012730640556902548}, {"x"=0.30282192, "y"=0.012730640556902548}, {"x"=0.30282192, "y"=0.012730640556902548}, {"x"=0.30282192, "y"=0.012730640556902548}, {"x"=0.30282192, "y"=0.012730640556902548}, {"x"=0.30282192, "y"=0.012730640556902548}, {"x"=0.30282192, "y"=0.012730640556902548}, {"x"=0.30282192, "y"=0.012730640556902548}, {"x"=0.30282192, "y"=0.012730640556902548}, {"x"=0.30282192, "y"=0.012730640556902548}, {"x"=0.30282192, "y"=0.012730640556902548}, {"x"=0.30282192, "y"=0.012730640556902548}, {"x"=0.30282192, "y"=0.012730640556902548}, {"x"=0.30282192, "y"=0.012730640556902548}, {"x"=0.30282192, "y"=0.012730640556902548}, {"x"=0.30282192, "y"=0.012730640556902548}, {"x"=0.30282192, "y"=0.012730640556902548}, {"x"=0.30282192, "y"=0.012730640556902548}, {"x"=0.30282192, "y"=0.012730640556902548}, {"x"=0.30282192, "y"=0.012730640556902548}, {"x"=0.30282192, "y"=0.012730640556902548}, {"x"=0.30282192, "y"=0.012730640556902548}, {"x"=0.30282192, "y"=0.012730640556902548}, {"x"=0.30282192, "y"=0.012730640556902548}, {"x"=0.30282192, "y"=0.012730640556902548}, {"x"=0.30282192, "y"=0.012730640556902548}, {"x"=0.30282192, "y"=0.012730640556902548}, {"x"=0.30282192, "y"=0.012730640556902548}, {"x"=0.30282192, "y"=0.012730640556902548}, {"x"=0.30282192, "y"=0.012730640556902548}, {"x"=0.30282192, "y"=0.012730640556902548}, {"x"=0.30282192, "y"=0.012730640556902548}, {"x"=0.30282192, "y"=0.012730640556902548}, {"x"=0.30282192, "y"=0.012730640556902548}, {"x"=0.30282192, "y"=0.012730640556902548}, {"x"=0.30282192, "y"=0.012730640556902548}, {"x"=0.30282192, "y"=0.012730640556902548}, {"x"=0.30282192, "y"=0.012730640556902548}, {"x"=0.30282192, "y"=0.012730640556902548}, {"x"=0.30282192, "y"=0.012730640556902548}, {"x"=0.30282192, "y"=0.012730640556902548}, {"x"=0.30282192, "y"=0.012730640556902548}, {"x"=0.30282192, "y"=0.012730640556902548}, {"x"=0.30282192, "y"=0.012730640556902548}, {"x"=0.30282192, "y"=0.012730640556902548}, {"x"=0.30282192, "y"=0.012730640556902548}, {"x"=0.30282192, "y"=0.012730640556902548}, {"x"=0.30282192, "y"=0.012730640556902548}, {"x"=0.30282192, "y"=0.012730640556902548}, {"x"=0.30282192, "y"=0.012730640556902548}, {"x"=0.30282192, "y"=0.012730640556902548}, {"x"=0.30282192, "y"=0.012730640556902548}, {"x"=0.30282192, "y"=0.012730640556902548}, {"x"=0.30282192, "y"=0.012730640556902548}, {"x"=0.30282192, "y"=0.012730640556902548}, {"x"=0.30282192, "y"=0.012730640556902548}, {"x"=0.30282192, "y"=0.012730640556902548}, {"x"=0.30282192, "y"=0.012730640556902548}, {"x"=0.30282192, "y"=0.012730640556902548}, {"x"=0.30282192, "y"=0.012730640556902548}, {"x"=0.30282192, "y"=0.012730640556902548}, {"x"=0.30282192, "y"=0.012730640556902548}, {"x"=0.30282192, "y"=0.012730640556902548}, {"x"=0.30282192, "y"=0.012730640556902548}, {"x"=0.30282192, "y"=0.012730640556902548}, {"x"=0.30282192, "y"=0.012730640556902548}, {"x"=0.30282192, "y"=0.012730640556902548}, {"x"=0.30282192, "y"=0.012730640556902548}, {"x"=0.30282192, "y"=0.012730640556902548}, {"x"=0.30282192, "y"=0.012730640556902548}, {"x"=0.30282192, "y"=0.012730640556902548}, {"x"=0.30282192, "y"=0.012730640556902548}, {"x"=0.30282192, "y"=0.012730640556902548}, {"x"=0.30282192, "y"=0.012730640556902548}, {"x"=0.30282192, "y"=0.012730640556902548}, {"x"=0.30282192, "y"=0.012730640556902548}, {"x"=0.30282192, "y"=0.012730640556902548}, {"x"=0.30282192, "y"=0.012730640556902548}, {"x"=0.30282192, "y"=0.012730640556902548}, {"x"=0.30282192, "y"=0.012730640556902548}, {"x"=0.30282192, "y"=0.012730640556902548}, {"x"=0.30282192, "y"=0.012730640556902548}, {"x"=0.30282192, "y"=0.012730640556902548}, {"x"=0.30282192, "y"=0.012730640556902548}, {"x"=0.30282192, "y"=0.012730640556902548}, {"x"=0.30282192, "y"=0.012730640556902548}, {"x"=0.30282192, "y"=0.012730640556902548}, {"x"=0.30282192, "y"=0.012730640556902548}, {"x"=0.30282192, "y"=0.012730640556902548}, {"x"=0.30282192, "y"=0.012730640556902548}, {"x"=0.30282192, "y"=0.012730640556902548}, {"x"=0.30282192, "y"=0.012730640556902548}, {"x"=0.30282192, "y"=0.012730640556902548}, {"x"=0.30282192, "y"=0.012730640556902548}, {"x"=0.30282192, "y"=0.012730640556902548}, {"x"=0.30282192, "y"=0.012730640556902548}, {"x"=0.30282192, "y"=0.012730640556902548}, {"x"=0.30282192, "y"=0.012730640556902548}, {"x"=0.30282192, "y"=0.012730640556902548}, {"x"=0.30282192, "y"=0.012730640556902548}, {"x"=0.30282192, "y"=0.012730640556902548}, {"x"=0.30282192, "y"=0.012730640556902548}, {"x"=0.30282192, "y"=0.012730640556902548}, {"x"=0.30282192, "y"=0.012730640556902548}, {"x"=0.30282192, "y"=0.012730640556902548}, {"x"=0.30282192, "y"=0.012730640556902548}, {"x"=0.30282192, "y"=0.012730640556902548}, {"x"=0.30282192, "y"=0.012730640556902548}, {"x"=0.30282192, "y"=0.012730640556902548}, {"x"=0.30282192, "y"=0.012730640556902548}, {"x"=0.30282192, "y"=0.012730640556902548}, {"x"=0.30282192, "y"=0.012730640556902548}, {"x"=0.30282192, "y"=0.012730640556902548}, {"x"=0.30282192, "y"=0.012730640556902548}, {"x"=0.30282192, "y"=0.012730640556902548}, {"x"=0.30282192, "y"=0.012730640556902548}, {"x"=0.30282192, "y"=0.012730640556902548}, {"x"=0.30282192, "y"=0.012730640556902548}, {"x"=0.30282192, "y"=0.012730640556902548}, {"x"=0.30282192, "y"=0.012730640556902548}, {"x"=0.30282192, "y"=0.012730640556902548}, {"x"=0.30282192, "y"=0.012730640556902548}, {"x"=0.30282192, "y"=0.012730640556902548}, {"x"=0.30282192, "y"=0.012730640556902548}, {"x"=0.30282192, "y"=0.012730640556902548}, {"x"=0.30282192, "y"=0.012730640556902548}, {"x"=0.30282192, "y"=0.012730640556902548}, {"x"=0.30282192, "y"=0.012730640556902548}, {"x"=0.30282192, "y"=0.012730640556902548}, {"x"=0.30282192, "y"=0.012730640556902548}, {"x"=0.30282192, "y"=0.012730640556902548}, {"x"=0.30282192, "y"=0.012730640556902548}, {"x"=0.30282192, "y"=0.012730640556902548}, {"x"=0.30282192, "y"=0.012730640556902548}, {"x"=0.30282192, "y"=0.012730640556902548}, {"x"=0.30282192, "y"=0.012730640556902548}, {"x"=0.30282192, "y"=0.012730640556902548}, {"x"=0.30282192, "y"=0.012730640556902548}, {"x"=0.30282192, "y"=0.012730640556902548}, {"x"=0.30282192, "y"=0.012730640556902548}, {"x"=0.30282192, "y"=0.012730640556902548}, {"x"=0.30282192, "y"=0.012730640556902548}, {"x"=0.30282192, "y"=0.012730640556902548}, {"x"=0.30282192, "y"=0.012730640556902548}, {"x"=0.30282192, "y"=0.012730640556902548}, {"x"=0.30282192, "y"=0.012730640556902548}, {"x"=0.30282192, "y"=0.012730640556902548}, {"x"=0.30282192, "y"=0.012730640556902548}, {"x"=0.30282192, "y"=0.012730640556902548}, {"x"=0.30282192, "y"=0.012730640556902548}, {"x"=0.30282192, "y"=0.012730640556902548}, {"x"=0.30282192, "y"=0.012730640556902548}, {"x"=0.30282192, "y"=0.012730640556902548}, {"x"=0.30282192, "y"=0.012730640556902548}, {"x"=0.30282192, "y"=0.012730640556902548}, {"x"=0.30282192, "y"=0.012730640556902548}, {"x"=0.30282192, "y"=0.012730640556902548}, {"x"=0.30282192, "y"=0.012730640556902548}, {"x"=0.30282192, "y"=0.012730640556902548}, {"x"=0.30282192, "y"=0.012730640556902548}, {"x"=0.30282192, "y"=0.012730640556902548}, {"x"=0.30282192, "y"=0.012730640556902548}, {"x"=0.30282192, "y"=0.012730640556902548}, {"x"=0.30282192, "y"=0.012730640556902548}, {"x"=0.30282192, "y"=0.012730640556902548}, {"x"=0.30282192, "y"=0.012730640556902548}, {"x"=0.30282192, "y"=0.012730640556902548}, {"x"=0.30282192, "y"=0.012730640556902548}, {"x"=0.30282192, "y"=0.012730640556902548}, {"x"=0.30282192, "y"=0.012730640556902548}, {"x"=0.30282192, "y"=0.012730640556902548}, {"x"=0.30282192, "y"=0.012730640556902548}, {"x"=0.30282192, "y"=0.012730640556902548}, {"x"=0.30282192, "y"=0.012730640556902548}, {"x"=0.30282192, "y"=0.012730640556902548}, {"x"=0.30282192, "y"=0.012730640556902548}, {"x"=0.30282192, "y"=0.012730640556902548}, {"x"=0.30282192, "y"=0.012730640556902548}, {"x"=0.30282192, "y"=0.012730640556902548}, {"x"=0.30282192, "y"=0.012730640556902548}, {"x"=0.30282192, "y"=0.012730640556902548}, {"x"=0.30282192, "y"=0.012730640556902548}, {"x"=0.30282192, "y"=0.012730640556902548}, {"x"=0.30282192, "y"=0.012730640556902548}, {"x"=0.30282192, "y"=0.012730640556902548}, {"x"=0.30282192, "y"=0.012730640556902548}, {"x"=0.30282192, "y"=0.012730640556902548}, {"x"=0.30282192, "y"=0.012730640556902548}, {"x"=0.30282192, "y"=0.012730640556902548}, {"x"=0.30282192, "y"=0.012730640556902548}, {"x"=0.30282192, "y"=0.012730640556902548}, {"x"=0.30282192, "y"=0.012730640556902548}, {"x"=0.30282192, "y"=0.012730640556902548}, {"x"=0.30282192, "y"=0.012730640556902548}, {"x"=0.30282192, "y"=0.012730640556902548}, {"x"=0.30282192, "y"=0.012730640556902548}, {"x"=0.30282192, "y"=0.012730640556902548}, {"x"=0.30282192, "y"=0.012730640556902548}, {"x"=0.30282192, "y"=0.012730640556902548}, {"x"=0.30282192, "y"=0.012730640556902548}, {"x"=0.30282192, "y"=0.012730640556902548}, {"x"=0.30282192, "y"=0.012730640556902548}, {"x"=0.30282192, "y"=0.012730640556902548}, {"x"=0.30282192, "y"=0.012730640556902548}, {"x"=0.30282192, "y"=0.012730640556902548}, {"x"=0.30282192, "y"=0.012730640556902548}, {"x"=0.30282192, "y"=0.012730640556902548}, {"x"=0.30282192, "y"=0.012730640556902548}, {"x"=0.30282192, "y"=0.012730640556902548}, {"x"=0.30282192, "y"=0.012730640556902548}, {"x"=0.30282192, "y"=0.012730640556902548}, {"x"=0.30282192, "y"=0.012730640556902548}, {"x"=0.30282192, "y"=0.012730640556902548}, {"x"=0.30282192, "y"=0.012730640556902548}, {"x"=0.30282192, "y"=0.012730640556902548}, {"x"=0.30282192, "y"=0.012730640556902548}, {"x"=0.30282192, "y"=0.012730640556902548}, {"x"=0.30282192, "y"=0.012730640556902548}, {"x"=0.30282192, "y"=0.012730640556902548}, {"x"=0.30282192, "y"=0.012730640556902548}, {"x"=0.30282192, "y"=0.012730640556902548}, {"x"=0.30282192, "y"=0.012730640556902548}, {"x"=0.30282192, "y"=0.012730640556902548}, {"x"=0.30282192, "y"=0.012730640556902548}, {"x"=0.30282192, "y"=0.012730640556902548}, {"x"=0.30282192, "y"=0.012730640556902548}, {"x"=0.30282192, "y"=0.012730640556902548}, {"x"=0.30282192, "y"=0.012730640556902548}, {"x"=0.30282192, "y"=0.012730640556902548}, {"x"=0.30282192, "y"=0.012730640556902548}, {"x"=0.30282192, "y"=0.012730640556902548}, {"x"=0.30282192, "y"=0.012730640556902548}, {"x"=0.30282192, "y"=0.012730640556902548}, {"x"=0.30282192, "y"=0.012730640556902548}, {"x"=0.30282192, "y"=0.012730640556902548}, {"x"=0.30282192, "y"=0.012730640556902548}, {"x"=0.30282192, "y"=0.012730640556902548}, {"x"=0.30282192, "y"=0.012730640556902548}, {"x"=0.30282192, "y"=0.012730640556902548}, {"x"=0.30282192, "y"=0.012730640556902548}, {"x"=0.30282192, "y"=0.012730640556902548}, {"x"=0.30282192, "y"=0.012730640556902548}, {"x"=0.30282192, "y"=0.012730640556902548}, {"x"=0.30282192, "y"=0.012730640556902548}, {"x"=0.30282192, "y"=0.012730640556902548}, {"x"=0.30282192, "y"=0.012730640556902548}, {"x"=0.30282192, "y"=0.012730640556902548}, {"x"=0.30282192, "y"=0.012730640556902548}, {"x"=0.30282192, "y"=0.012730640556902548}, {"x"=0.30282192, "y"=0.012730640556902548}, {"x"=0.30282192, "y"=0.012730640556902548}, {"x"=0.30282192, "y"=0.012730640556902548}, {"x"=0.30282192, "y"=0.012730640556902548}, {"x"=0.30282192, "y"=0.012730640556902548}, {"x"=0.30282192, "y"=0.012730640556902548}, {"x"=0.30282192, "y"=0.012730640556902548}, {"x"=0.30282192, "y"=0.012730640556902548}, {"x"=0.30282192, "y"=0.012730640556902548}, {"x"=0.30282192, "y"=0.012730640556902548}, {"x"=0.30282192, "y"=0.012730640556902548}, {"x"=0.30282192, "y"=0.012730640556902548}, {"x"=0.30282192, "y"=0.012730640556902548}, {"x"=0.30282192, "y"=0.012730640556902548}, {"x"=0.30282192, "y"=0.012730640556902548}, {"x"=0.30282192, "y"=0.012730640556902548}, {"x"=0.30282192, "y"=0.012730640556902548}, {"x"=0.30282192, "y"=0.012730640556902548}, {"x"=0.30282192, "y"=0.012730640556902548}, {"x"=0.30282192, "y"=0.012730640556902548}, {"x"=0.30282192, "y"=0.012730640556902548}, {"x"=0.30282192, "y"=0.012730640556902548}, {"x"=0.30282192, "y"=0.012730640556902548}, {"x"=0.30282192, "y"=0.012730640556902548}, {"x"=0.30282192, "y"=0.012730640556902548}, {"x"=0.30282192, "y"=0.012730640556902548}, {"x"=0.30282192, "y"=0.012730640556902548}, {"x"=0.30282192, "y"=0.012730640556902548}, {"x"=0.30282192, "y"=0.012730640556902548}, {"x"=0.30282192, "y"=0.012730640556902548}, {"x"=0.30282192, "y"=0.012730640556902548}, {"x"=0.30282192, "y"=0.012730640556902548}, {"x"=0.30282192, "y"=0.012730640556902548}, {"x"=0.30282192, "y"=0.012730640556902548}, {"x"=0.30282192, "y"=0.012730640556902548}, {"x"=0.30282192, "y"=0.012730640556902548}, {"x"=0.30282192, "y"=0.012730640556902548}, {"x"=0.30282192, "y"=0.012730640556902548}, {"x"=0.30282192, "y"=0.012730640556902548}, {"x"=0.30282192, "y"=0.012730640556902548}, {"x"=0.30282192, "y"=0.012730640556902548}, {"x"=0.30282192, "y"=0.012730640556902548}, {"x"=0.30282192, "y"=0.012730640556902548}, {"x"=0.30282192, "y"=0.012730640556902548}, {"x"=0.30282192, "y"=0.012730640556902548}, {"x"=0.30282192, "y"=0.012730640556902548}, {"x"=0.30282192, "y"=0.012730640556902548}, {"x"=0.30282192, "y"=0.012730640556902548}, {"x"=0.30282192, "y"=0.012730640556902548}, {"x"=0.30282192, "y"=0.012730640556902548}, {"x"=0.30282192, "y"=0.012730640556902548}, {"x"=0.30282192, "y"=0.012730640556902548}, {"x"=0.30282192, "y"=0.012730640556902548}, {"x"=0.30282192, "y"=0.012730640556902548}, {"x"=0.30282192, "y"=0.012730640556902548}, {"x"=0.30282192, "y"=0.012730640556902548}, {"x"=0.30282192, "y"=0.012730640556902548}, {"x"=0.30282192, "y"=0.012730640556902548}, {"x"=0.30282192, "y"=0.012730640556902548}, {"x"=0.30282192, "y"=0.012730640556902548}, {"x"=0.30282192, "y"=0.012730640556902548}, {"x"=0.30282192, "y"=0.012730640556902548}, {"x"=0.30282192, "y"=0.012730640556902548}, {"x"=0.30282192, "y"=0.012730640556902548}, {"x"=0.30282192, "y"=0.012730640556902548}, {"x"=0.30282192, "y"=0.012730640556902548}, {"x"=0.30282192, "y"=0.012730640556902548}, {"x"=0.30282192, "y"=0.012730640556902548}, {"x"=0.30282192, "y"=0.012730640556902548}, {"x"=0.30282192, "y"=0.012730640556902548}, {"x"=0.30282192, "y"=0.012730640556902548}, {"x"=0.30282192, "y"=0.012730640556902548}, {"x"=0.30282192, "y"=0.012730640556902548}, {"x"=0.30282192, "y"=0.012730640556902548}, {"x"=0.30282192, "y"=0.012730640556902548}, {"x"=0.30282192, "y"=0.012730640556902548}, {"x"=0.30282192, "y"=0.012730640556902548}, {"x"=0.30282192, "y"=0.012730640556902548}, {"x"=0.30282192, "y"=0.012730640556902548}, {"x"=0.30282192, "y"=0.012730640556902548}, {"x"=0.30282192, "y"=0.012730640556902548}, {"x"=0.30282192, "y"=0.012730640556902548}, {"x"=0.30282192, "y"=0.012730640556902548}, {"x"=0.30282192, "y"=0.012730640556902548}, {"x"=0.30282192, "y"=0.012730640556902548}, {"x"=0.30282192, "y"=0.012730640556902548}, {"x"=0.30282192, "y"=0.012730640556902548}, {"x"=0.30282192, "y"=0.012730640556902548}, {"x"=0.30282192, "y"=0.012730640556902548}, {"x"=0.30282192, "y"=0.012730640556902548}, {"x"=0.30282192, "y"=0.012730640556902548}, {"x"=0.30282192, "y"=0.012730640556902548}, {"x"=0.30282192, "y"=0.012730640556902548}, {"x"=0.30282192, "y"=0.012730640556902548}, {"x"=0.30282192, "y"=0.012730640556902548}, {"x"=0.30282192, "y"=0.012730640556902548}, {"x"=0.30282192, "y"=0.012730640556902548}, {"x"=0.30282192, "y"=0.012730640556902548}, {"x"=0.30282192, "y"=0.012730640556902548}, {"x"=0.30282192, "y"=0.012730640556902548}, {"x"=0.30282192, "y"=0.012730640556902548}, {"x"=0.30282192, "y"=0.012730640556902548}, {"x"=0.30282192, "y"=0.012730640556902548}, {"x"=0.30282192, "y"=0.012730640556902548}, {"x"=0.30282192, "y"=0.012730640556902548}, {"x"=0.30282192, "y"=0.012730640556902548}, {"x"=0.30282192, "y"=0.012730640556902548}, {"x"=0.30282192, "y"=0.012730640556902548}, {"x"=0.30282192, "y"=0.012730640556902548}, {"x"=0.30282192, "y"=0.012730640556902548}, {"x"=0.30282192, "y"=0.012730640556902548}, {"x"=0.30282192, "y"=0.012730640556902548}, {"x"=0.30282192, "y"=0.012730640556902548}, {"x"=0.30282192, "y"=0.012730640556902548}, {"x"=0.30282192, "y"=0.012730640556902548}, {"x"=0.30282192, "y"=0.012730640556902548}, {"x"=0.30282192, "y"=0.012730640556902548}, {"x"=0.30282192, "y"=0.012730640556902548}, {"x"=0.30282192, "y"=0.012730640556902548}, {"x"=0.30282192, "y"=0.012730640556902548}, {"x"=0.30282192, "y"=0.012730640556902548}, {"x"=0.30282192, "y"=0.012730640556902548}, {"x"=0.30282192, "y"=0.012730640556902548}, {"x"=0.30282192, "y"=0.012730640556902548}, {"x"=0.30282192, "y"=0.012730640556902548}, {"x"=0.30282192, "y"=0.012730640556902548}, {"x"=0.30282192, "y"=0.012730640556902548}, {"x"=0.30282192, "y"=0.012730640556902548}, {"x"=0.30282192, "y"=0.012730640556902548}, {"x"=0.30282192, "y"=0.012730640556902548}, {"x"=0.30282192, "y"=0.012730640556902548}, {"x"=0.30282192, "y"=0.012730640556902548}, {"x"=0.30282192, "y"=0.012730640556902548}, {"x"=0.30282192, "y"=0.012730640556902548}, {"x"=0.30282192, "y"=0.012730640556902548}, {"x"=0.30282192, "y"=0.012730640556902548}, {"x"=0.30282192, "y"=0.012730640556902548}, {"x"=0.30282192, "y"=0.012730640556902548}, {"x"=0.30282192, "y"=0.012730640556902548}, {"x"=0.30282192, "y"=0.012730640556902548}, {"x"=0.30282192, "y"=0.012730640556902548}, {"x"=0.30282192, "y"=0.012730640556902548}, {"x"=0.30282192, "y"=0.012730640556902548}, {"x"=0.30282192, "y"=0.012730640556902548}, {"x"=0.30282192, "y"=0.012730640556902548}, {"x"=0.30282192, "y"=0.012730640556902548}, {"x"=0.30282192, "y"=0.012730640556902548}, {"x"=0.30282192, "y"=0.012730640556902548}, {"x"=0.30282192, "y"=0.012730640556902548}, {"x"=0.30282192, "y"=0.012730640556902548}, {"x"=0.30282192, "y"=0.012730640556902548}, {"x"=0.30282192, "y"=0.012730640556902548}, {"x"=0.30282192, "y"=0.012730640556902548}, {"x"=0.30282192, "y"=0.012730640556902548}, {"x"=0.30282192, "y"=0.012730640556902548}, {"x"=0.30282192, "y"=0.012730640556902548}, {"x"=0.30282192, "y"=0.012730640556902548}, {"x"=0.30282192, "y"=0.012730640556902548}, {"x"=0.30282192, "y"=0.012730640556902548}, {"x"=0.30282192, "y"=0.012730640556902548}, {"x"=0.30282192, "y"=0.012730640556902548}, {"x"=0.30282192, "y"=0.012730640556902548}, {"x"=0.30282192, "y"=0.012730640556902548}, {"x"=0.30282192, "y"=0.012730640556902548}, {"x"=0.30282192, "y"=0.012730640556902548}, {"x"=0.30282192, "y"=0.012730640556902548}, {"x"=0.30282192, "y"=0.012730640556902548}, {"x"=0.30282192, "y"=0.012730640556902548}, {"x"=0.30282192, "y"=0.012730640556902548}, {"x"=0.30282192, "y"=0.012730640556902548}, {"x"=0.30282192, "y"=0.012730640556902548}, {"x"=0.30282192, "y"=0.012730640556902548}, {"x"=0.30282192, "y"=0.012730640556902548}, {"x"=0.30282192, "y"=0.012730640556902548}, {"x"=0.30282192, "y"=0.012730640556902548}, {"x"=0.30282192, "y"=0.012730640556902548}, {"x"=0.30282192, "y"=0.012730640556902548}, {"x"=0.30282192, "y"=0.012730640556902548}, {"x"=0.30282192, "y"=0.012730640556902548}, {"x"=0.30282192, "y"=0.012730640556902548}, {"x"=0.30282192, "y"=0.012730640556902548}, {"x"=0.30282192, "y"=0.012730640556902548}, {"x"=0.30282192, "y"=0.012730640556902548}, {"x"=0.30282192, "y"=0.012730640556902548}, {"x"=0.30282192, "y"=0.012730640556902548}, {"x"=0.30282192, "y"=0.012730640556902548}, {"x"=0.30282192, "y"=0.012730640556902548}, {"x"=0.30282192, "y"=0.012730640556902548}, {"x"=0.30282192, "y"=0.012730640556902548}, {"x"=0.30282192, "y"=0.012730640556902548}, {"x"=0.30282192, "y"=0.012730640556902548}, {"x"=0.30282192, "y"=0.012730640556902548}, {"x"=0.30282192, "y"=0.012730640556902548}, {"x"=0.30282192, "y"=0.012730640556902548}, {"x"=0.30282192, "y"=0.012730640556902548}, {"x"=0.30282192, "y"=0.012730640556902548}, {"x"=0.30282192, "y"=0.012730640556902548}, {"x"=0.30282192, "y"=0.012730640556902548}, {"x"=0.30282192, "y"=0.012730640556902548}, {"x"=0.30282192, "y"=0.012730640556902548}, {"x"=0.30282192, "y"=0.012730640556902548}, {"x"=0.30282192, "y"=0.012730640556902548}, {"x"=0.30282192, "y"=0.012730640556902548}, {"x"=0.30282192, "y"=0.012730640556902548}, {"x"=0.30282192, "y"=0.012730640556902548}, {"x"=0.30282192, "y"=0.012730640556902548}, {"x"=0.30282192, "y"=0.012730640556902548}, {"x"=0.30282192, "y"=0.012730640556902548}, {"x"=0.30282192, "y"=0.012730640556902548}, {"x"=0.30282192, "y"=0.012730640556902548}, {"x"=0.30282192, "y"=0.012730640556902548}, {"x"=0.30282192, "y"=0.012730640556902548}, {"x"=0.30282192, "y"=0.012730640556902548}, {"x"=0.30282192, "y"=0.012730640556902548}, {"x"=0.30282192, "y"=0.012730640556902548}, {"x"=0.30282192, "y"=0.012730640556902548}, {"x"=0.30282192, "y"=0.012730640556902548}, {"x"=0.30282192, "y"=0.012730640556902548}, {"x"=0.30282192, "y"=0.012730640556902548}, {"x"=0.30282192, "y"=0.012730640556902548}, {"x"=0.30282192, "y"=0.012730640556902548}, {"x"=0.30282192, "y"=0.012730640556902548}, {"x"=0.30282192, "y"=0.012730640556902548}, {"x"=0.30282192, "y"=0.012730640556902548}, {"x"=0.30282192, "y"=0.012730640556902548}, {"x"=0.30282192, "y"=0.012730640556902548}, {"x"=0.30282192, "y"=0.012730640556902548}, {"x"=0.30282192, "y"=0.012730640556902548}, {"x"=0.30282192, "y"=0.012730640556902548}, {"x"=0.30282192, "y"=0.012730640556902548}, {"x"=0.30282192, "y"=0.012730640556902548}, {"x"=0.30282192, "y"=0.012730640556902548}, {"x"=0.30282192, "y"=0.012730640556902548}, {"x"=0.30282192, "y"=0.012730640556902548}, {"x"=0.30282192, "y"=0.012730640556902548}, {"x"=0.30282192, "y"=0.012730640556902548}, {"x"=0.30282192, "y"=0.012730640556902548}, {"x"=0.30282192, "y"=0.012730640556902548}, {"x"=0.30282192, "y"=0.012730640556902548}, {"x"=0.30282192, "y"=0.012730640556902548}, {"x"=0.30282192, "y"=0.012730640556902548}, {"x"=0.30282192, "y"=0.012730640556902548}, {"x"=0.30282192, "y"=0.012730640556902548}, {"x"=0.30282192, "y"=0.012730640556902548}, {"x"=0.30282192, "y"=0.012730640556902548}, {"x"=0.30282192, "y"=0.012730640556902548}, {"x"=0.30282192, "y"=0.012730640556902548}, {"x"=0.30282192, "y"=0.012730640556902548}, {"x"=0.30282192, "y"=0.012730640556902548}, {"x"=0.30282192, "y"=0.012730640556902548}, {"x"=0.30282192, "y"=0.012730640556902548}, {"x"=0.30282192, "y"=0.012730640556902548}, {"x"=0.30282192, "y"=0.012730640556902548}, {"x"=0.30282192, "y"=0.012730640556902548}, {"x"=0.30282192, "y"=0.012730640556902548}, {"x"=0.30282192, "y"=0.012730640556902548}, {"x"=0.30282192, "y"=0.012730640556902548}, {"x"=0.30282192, "y"=0.012730640556902548}, {"x"=0.30282192, "y"=0.012730640556902548}, {"x"=0.30282192, "y"=0.012730640556902548}, {"x"=0.30282192, "y"=0.012730640556902548}, {"x"=0.30282192, "y"=0.012730640556902548}, {"x"=0.30282192, "y"=0.012730640556902548}, {"x"=0.30282192, "y"=0.012730640556902548}, {"x"=0.30282192, "y"=0.012730640556902548}, {"x"=0.30282192, "y"=0.012730640556902548}, {"x"=0.30282192, "y"=0.012730640556902548}, {"x"=0.30282192, "y"=0.012730640556902548}, {"x"=0.30282192, "y"=0.012730640556902548}, {"x"=0.30282192, "y"=0.012730640556902548}, {"x"=0.30282192, "y"=0.012730640556902548}, {"x"=0.30282192, "y"=0.012730640556902548}, {"x"=0.30282192, "y"=0.012730640556902548}, {"x"=0.30282192, "y"=0.012730640556902548}, {"x"=0.30282192, "y"=0.012730640556902548}, {"x"=0.30282192, "y"=0.012730640556902548}, {"x"=0.30282192, "y"=0.012730640556902548}, {"x"=0.30282192, "y"=0.012730640556902548}, {"x"=0.30282192, "y"=0.012730640556902548}, {"x"=0.30282192, "y"=0.012730640556902548}, {"x"=0.30282192, "y"=0.012730640556902548}, {"x"=0.30282192, "y"=0.012730640556902548}, {"x"=0.30282192, "y"=0.012730640556902548}, {"x"=0.30282192, "y"=0.012730640556902548}, {"x"=0.30282192, "y"=0.012730640556902548}, {"x"=0.30282192, "y"=0.012730640556902548}, {"x"=0.30282192, "y"=0.012730640556902548}, {"x"=0.30282192, "y"=0.012730640556902548}, {"x"=0.30282192, "y"=0.012730640556902548}, {"x"=0.30282192, "y"=0.012730640556902548}, {"x"=0.30282192, "y"=0.012730640556902548}, {"x"=0.30282192, "y"=0.012730640556902548}, {"x"=0.30282192, "y"=0.012730640556902548}, {"x"=0.30282192, "y"=0.012730640556902548}, {"x"=0.30282192, "y"=0.012730640556902548}, {"x"=0.30282192, "y"=0.012730640556902548}, {"x"=0.30282192, "y"=0.012730640556902548}, {"x"=0.30282192, "y"=0.012730640556902548}, {"x"=0.30282192, "y"=0.012730640556902548}, {"x"=0.30282192, "y"=0.012730640556902548}, {"x"=0.30282192, "y"=0.012730640556902548}, {"x"=0.30282192, "y"=0.012730640556902548}, {"x"=0.30282192, "y"=0.012730640556902548}, {"x"=0.30282192, "y"=0.012730640556902548}, {"x"=0.30282192, "y"=0.012730640556902548}, {"x"=0.30282192, "y"=0.012730640556902548}, {"x"=0.30282192, "y"=0.012730640556902548}, {"x"=0.30282192, "y"=0.012730640556902548}, {"x"=0.30282192, "y"=0.012730640556902548}, {"x"=0.30282192, "y"=0.012730640556902548}, {"x"=0.30282192, "y"=0.012730640556902548}, {"x"=0.30282192, "y"=0.012730640556902548}, {"x"=0.30282192, "y"=0.012730640556902548}, {"x"=0.30282192, "y"=0.012730640556902548}, {"x"=0.30282192, "y"=0.012730640556902548}, {"x"=0.30282192, "y"=0.012730640556902548}, {"x"=0.30282192, "y"=0.012730640556902548}, {"x"=0.30282192, "y"=0.012730640556902548}, {"x"=0.30282192, "y"=0.012730640556902548}, {"x"=0.30282192, "y"=0.012730640556902548}, {"x"=0.30282192, "y"=0.012730640556902548}, {"x"=0.30282192, "y"=0.012730640556902548}, {"x"=0.30282192, "y"=0.012730640556902548}, {"x"=0.30282192, "y"=0.012730640556902548}, {"x"=0.30282192, "y"=0.012730640556902548}, {"x"=0.30282192, "y"=0.012730640556902548}, {"x"=0.30282192, "y"=0.012730640556902548}, {"x"=0.30282192, "y"=0.012730640556902548}, {"x"=0.30282192, "y"=0.012730640556902548}, {"x"=0.30282192, "y"=0.012730640556902548}, {"x"=0.30282192, "y"=0.012730640556902548}, {"x"=0.30282192, "y"=0.012730640556902548}, {"x"=0.30282192, "y"=0.012730640556902548}, {"x"=0.30282192, "y"=0.012730640556902548}, {"x"=0.30282192, "y"=0.012730640556902548}, {"x"=0.30282192, "y"=0.012730640556902548}, {"x"=0.30282192, "y"=0.012730640556902548}, {"x"=0.30282192, "y"=0.012730640556902548}, {"x"=0.30282192, "y"=0.012730640556902548}, {"x"=0.30282192, "y"=0.012730640556902548}, {"x"=0.30282192, "y"=0.012730640556902548}, {"x"=0.30282192, "y"=0.012730640556902548}, {"x"=0.30282192, "y"=0.012730640556902548}, {"x"=0.30282192, "y"=0.012730640556902548}, {"x"=0.30282192, "y"=0.012730640556902548}, {"x"=0.30282192, "y"=0.012730640556902548}, {"x"=0.30282192, "y"=0.012730640556902548}, {"x"=0.30282192, "y"=0.012730640556902548}, {"x"=0.30282192, "y"=0.012730640556902548}, {"x"=0.30282192, "y"=0.012730640556902548}, {"x"=0.30282192, "y"=0.012730640556902548}, {"x"=0.30282192, "y"=0.012730640556902548}, {"x"=0.30282192, "y"=0.012730640556902548}, {"x"=0.30282192, "y"=0.012730640556902548}, {"x"=0.30282192, "y"=0.012730640556902548}, {"x"=0.30282192, "y"=0.012730640556902548}, {"x"=0.30282192, "y"=0.012730640556902548}, {"x"=0.30282192, "y"=0.012730640556902548}, {"x"=0.30282192, "y"=0.012730640556902548}, {"x"=0.30282192, "y"=0.012730640556902548}, {"x"=0.30282192, "y"=0.012730640556902548}, {"x"=0.30282192, "y"=0.012730640556902548}, {"x"=0.30282192, "y"=0.012730640556902548}, {"x"=0.30282192, "y"=0.012730640556902548}, {"x"=0.30282192, "y"=0.012730640556902548}, {"x"=0.30282192, "y"=0.012730640556902548}, {"x"=0.30282192, "y"=0.012730640556902548}, {"x"=0.30282192, "y"=0.012730640556902548}, {"x"=0.30282192, "y"=0.012730640556902548}, {"x"=0.30282192, "y"=0.012730640556902548}, {"x"=0.30282192, "y"=0.012730640556902548}, {"x"=0.30282192, "y"=0.012730640556902548}, {"x"=0.30282192, "y"=0.012730640556902548}, {"x"=0.30282192, "y"=0.012730640556902548}, {"x"=0.30282192, "y"=0.012730640556902548}, {"x"=0.30282192, "y"=0.012730640556902548}, {"x"=0.30282192, "y"=0.012730640556902548}, {"x"=0.30282192, "y"=0.012730640556902548}, {"x"=0.30282192, "y"=0.012730640556902548}, {"x"=0.30282192, "y"=0.012730640556902548}, {"x"=0.30282192, "y"=0.012730640556902548}, {"x"=0.30282192, "y"=0.012730640556902548}, {"x"=0.30282192, "y"=0.012730640556902548}]
  in  "Min_LIA1_Signal":dbl=0.035
  in  "MAX LIA_1_Signal":dbl=0.65
  in  "MAX V_drop_Signal":dbl=0.35
  in  "Min_Vdrop_Signal":dbl=0.028
  in  "LIA2_internal":bool=TRUE
  in  "auto_amp_high_gain":dbl=0.25
  in  "auto_amp_low_gain":dbl=0.2
  in  "ampl. high_low_G":T5(ring)=enum."10^7"
  in  "ampl. low_low_G":T5(ring)=enum."10^8"
  in  "ampl. high_high_G":T5(ring)=enum."10^6"
  in  "amp_very_low_gain":dbl=0.2
  out "lia 2 phase":dbl=-93.672
  out "phase_Lia1":dbl=76.77
  in  "min_temp_limit":dbl=35.0 format="%#_13g"
  out "?":cluster{"x":dbl, "y":dbl}[](graph)=[{"x"=0.30282192, "y"=0.780048243}, {"x"=0.30282192, "y"=0.780048243}, {"x"=0.30282192, "y"=0.780048243}, {"x"=0.30282192, "y"=0.780048243}, {"x"=0.30282192, "y"=0.780048243}, {"x"=0.30282192, "y"=0.780048243}, {"x"=0.30282192, "y"=0.780048243}, {"x"=0.30282192, "y"=0.780048243}, {"x"=0.30282192, "y"=0.780048243}, {"x"=0.30282192, "y"=0.780048243}, {"x"=0.30282192, "y"=0.780048243}, {"x"=0.30282192, "y"=0.780048243}, {"x"=0.30282192, "y"=0.780048243}, {"x"=0.30282192, "y"=0.780048243}, {"x"=0.30282192, "y"=0.780048243}, {"x"=0.30282192, "y"=0.780048243}, {"x"=0.30282192, "y"=0.780048243}, {"x"=0.30282192, "y"=0.780048243}, {"x"=0.30282192, "y"=0.780048243}, {"x"=0.30282192, "y"=0.780048243}, {"x"=0.30282192, "y"=0.780048243}, {"x"=0.30282192, "y"=0.780048243}, {"x"=0.30282192, "y"=0.780048243}, {"x"=0.30282192, "y"=0.780048243}, {"x"=0.30282192, "y"=0.780048243}, {"x"=0.30282192, "y"=0.780048243}, {"x"=0.30282192, "y"=0.780048243}, {"x"=0.30282192, "y"=0.780048243}, {"x"=0.30282192, "y"=0.780048243}, {"x"=0.30282192, "y"=0.780048243}, {"x"=0.30282192, "y"=0.780048243}, {"x"=0.30282192, "y"=0.780048243}, {"x"=0.30282192, "y"=0.780048243}, {"x"=0.30282192, "y"=0.780048243}, {"x"=0.30282192, "y"=0.780048243}, {"x"=0.30282192, "y"=0.780048243}, {"x"=0.30282192, "y"=0.780048243}, {"x"=0.30282192, "y"=0.780048243}, {"x"=0.30282192, "y"=0.780048243}, {"x"=0.30282192, "y"=0.780048243}, {"x"=0.30282192, "y"=0.780048243}, {"x"=0.30282192, "y"=0.780048243}, {"x"=0.30282192, "y"=0.780048243}, {"x"=0.30282192, "y"=0.780048243}, {"x"=0.30282192, "y"=0.780048243}, {"x"=0.30282192, "y"=0.780048243}, {"x"=0.30282192, "y"=0.780048243}, {"x"=0.30282192, "y"=0.780048243}, {"x"=0.30282192, "y"=0.780048243}, {"x"=0.30282192, "y"=0.780048243}, {"x"=0.30282192, "y"=0.780048243}, {"x"=0.30282192, "y"=0.780048243}, {"x"=0.30282192, "y"=0.780048243}, {"x"=0.30282192, "y"=0.780048243}, {"x"=0.30282192, "y"=0.780048243}, {"x"=0.30282192, "y"=0.780048243}, {"x"=0.30282192, "y"=0.780048243}, {"x"=0.30282192, "y"=0.780048243}, {"x"=0.30282192, "y"=0.780048243}, {"x"=0.30282192, "y"=0.780048243}, {"x"=0.30282192, "y"=0.780048243}, {"x"=0.30282192, "y"=0.780048243}, {"x"=0.30282192, "y"=0.780048243}, {"x"=0.30282192, "y"=0.780048243}, {"x"=0.30282192, "y"=0.780048243}, {"x"=0.30282192, "y"=0.780048243}, {"x"=0.30282192, "y"=0.780048243}, {"x"=0.30282192, "y"=0.780048243}, {"x"=0.30282192, "y"=0.780048243}, {"x"=0.30282192, "y"=0.780048243}, {"x"=0.30282192, "y"=0.780048243}, {"x"=0.30282192, "y"=0.780048243}, {"x"=0.30282192, "y"=0.780048243}, {"x"=0.30282192, "y"=0.780048243}, {"x"=0.30282192, "y"=0.780048243}, {"x"=0.30282192, "y"=0.780048243}, {"x"=0.30282192, "y"=0.780048243}, {"x"=0.30282192, "y"=0.780048243}, {"x"=0.30282192, "y"=0.780048243}, {"x"=0.30282192, "y"=0.780048243}, {"x"=0.30282192, "y"=0.780048243}, {"x"=0.30282192, "y"=0.780048243}, {"x"=0.30282192, "y"=0.780048243}, {"x"=0.30282192, "y"=0.780048243}, {"x"=0.30282192, "y"=0.780048243}, {"x"=0.30282192, "y"=0.780048243}, {"x"=0.30282192, "y"=0.780048243}, {"x"=0.30282192, "y"=0.780048243}, {"x"=0.30282192, "y"=0.780048243}, {"x"=0.30282192, "y"=0.780048243}, {"x"=0.30282192, "y"=0.780048243}, {"x"=0.30282192, "y"=0.780048243}, {"x"=0.30282192, "y"=0.780048243}, {"x"=0.30282192, "y"=0.780048243}, {"x"=0.30282192, "y"=0.780048243}, {"x"=0.30282192, "y"=0.780048243}, {"x"=0.30282192, "y"=0.780048243}, {"x"=0.30282192, "y"=0.780048243}, {"x"=0.30282192, "y"=0.780048243}, {"x"=0.30282192, "y"=0.780048243}, {"x"=0.30282192, "y"=0.780048243}, {"x"=0.30282192, "y"=0.780048243}, {"x"=0.30282192, "y"=0.780048243}, {"x"=0.30282192, "y"=0.780048243}, {"x"=0.30282192, "y"=0.780048243}, {"x"=0.30282192, "y"=0.780048243}, {"x"=0.30282192, "y"=0.780048243}, {"x"=0.30282192, "y"=0.780048243}, {"x"=0.30282192, "y"=0.780048243}, {"x"=0.30282192, "y"=0.780048243}, {"x"=0.30282192, "y"=0.780048243}, {"x"=0.30282192, "y"=0.780048243}, {"x"=0.30282192, "y"=0.780048243}, {"x"=0.30282192, "y"=0.780048243}, {"x"=0.30282192, "y"=0.780048243}, {"x"=0.30282192, "y"=0.780048243}, {"x"=0.30282192, "y"=0.780048243}, {"x"=0.30282192, "y"=0.780048243}, {"x"=0.30282192, "y"=0.780048243}, {"x"=0.30282192, "y"=0.780048243}, {"x"=0.30282192, "y"=0.780048243}, {"x"=0.30282192, "y"=0.780048243}, {"x"=0.30282192, "y"=0.780048243}, {"x"=0.30282192, "y"=0.780048243}, {"x"=0.30282192, "y"=0.780048243}, {"x"=0.30282192, "y"=0.780048243}, {"x"=0.30282192, "y"=0.780048243}, {"x"=0.30282192, "y"=0.780048243}, {"x"=0.30282192, "y"=0.780048243}, {"x"=0.30282192, "y"=0.780048243}, {"x"=0.30282192, "y"=0.780048243}, {"x"=0.30282192, "y"=0.780048243}, {"x"=0.30282192, "y"=0.780048243}, {"x"=0.30282192, "y"=0.780048243}, {"x"=0.30282192, "y"=0.780048243}, {"x"=0.30282192, "y"=0.780048243}, {"x"=0.30282192, "y"=0.780048243}, {"x"=0.30282192, "y"=0.780048243}, {"x"=0.30282192, "y"=0.780048243}, {"x"=0.30282192, "y"=0.780048243}, {"x"=0.30282192, "y"=0.780048243}, {"x"=0.30282192, "y"=0.780048243}, {"x"=0.30282192, "y"=0.780048243}, {"x"=0.30282192, "y"=0.780048243}, {"x"=0.30282192, "y"=0.780048243}, {"x"=0.30282192, "y"=0.780048243}, {"x"=0.30282192, "y"=0.780048243}, {"x"=0.30282192, "y"=0.780048243}, {"x"=0.30282192, "y"=0.780048243}, {"x"=0.30282192, "y"=0.780048243}, {"x"=0.30282192, "y"=0.780048243}, {"x"=0.30282192, "y"=0.780048243}, {"x"=0.30282192, "y"=0.780048243}, {"x"=0.30282192, "y"=0.780048243}, {"x"=0.30282192, "y"=0.780048243}, {"x"=0.30282192, "y"=0.780048243}, {"x"=0.30282192, "y"=0.780048243}, {"x"=0.30282192, "y"=0.780048243}, {"x"=0.30282192, "y"=0.780048243}, {"x"=0.30282192, "y"=0.780048243}, {"x"=0.30282192, "y"=0.780048243}, {"x"=0.30282192, "y"=0.780048243}, {"x"=0.30282192, "y"=0.780048243}, {"x"=0.30282192, "y"=0.780048243}, {"x"=0.30282192, "y"=0.780048243}, {"x"=0.30282192, "y"=0.780048243}, {"x"=0.30282192, "y"=0.780048243}, {"x"=0.30282192, "y"=0.780048243}, {"x"=0.30282192, "y"=0.780048243}, {"x"=0.30282192, "y"=0.780048243}, {"x"=0.30282192, "y"=0.780048243}, {"x"=0.30282192, "y"=0.780048243}, {"x"=0.30282192, "y"=0.780048243}, {"x"=0.30282192, "y"=0.780048243}, {"x"=0.30282192, "y"=0.780048243}, {"x"=0.30282192, "y"=0.780048243}, {"x"=0.30282192, "y"=0.780048243}, {"x"=0.30282192, "y"=0.780048243}, {"x"=0.30282192, "y"=0.780048243}, {"x"=0.30282192, "y"=0.780048243}, {"x"=0.30282192, "y"=0.780048243}, {"x"=0.30282192, "y"=0.780048243}, {"x"=0.30282192, "y"=0.780048243}, {"x"=0.30282192, "y"=0.780048243}, {"x"=0.30282192, "y"=0.780048243}, {"x"=0.30282192, "y"=0.780048243}, {"x"=0.30282192, "y"=0.780048243}, {"x"=0.30282192, "y"=0.780048243}, {"x"=0.30282192, "y"=0.780048243}, {"x"=0.30282192, "y"=0.780048243}, {"x"=0.30282192, "y"=0.780048243}, {"x"=0.30282192, "y"=0.780048243}, {"x"=0.30282192, "y"=0.780048243}, {"x"=0.30282192, "y"=0.780048243}, {"x"=0.30282192, "y"=0.780048243}, {"x"=0.30282192, "y"=0.780048243}, {"x"=0.30282192, "y"=0.780048243}, {"x"=0.30282192, "y"=0.780048243}, {"x"=0.30282192, "y"=0.780048243}, {"x"=0.30282192, "y"=0.780048243}, {"x"=0.30282192, "y"=0.780048243}, {"x"=0.30282192, "y"=0.780048243}, {"x"=0.30282192, "y"=0.780048243}, {"x"=0.30282192, "y"=0.780048243}, {"x"=0.30282192, "y"=0.780048243}, {"x"=0.30282192, "y"=0.780048243}, {"x"=0.30282192, "y"=0.780048243}, {"x"=0.30282192, "y"=0.780048243}, {"x"=0.30282192, "y"=0.780048243}, {"x"=0.30282192, "y"=0.780048243}, {"x"=0.30282192, "y"=0.780048243}, {"x"=0.30282192, "y"=0.780048243}, {"x"=0.30282192, "y"=0.780048243}, {"x"=0.30282192, "y"=0.780048243}, {"x"=0.30282192, "y"=0.780048243}, {"x"=0.30282192, "y"=0.780048243}, {"x"=0.30282192, "y"=0.780048243}, {"x"=0.30282192, "y"=0.780048243}, {"x"=0.30282192, "y"=0.780048243}, {"x"=0.30282192, "y"=0.780048243}, {"x"=0.30282192, "y"=0.780048243}, {"x"=0.30282192, "y"=0.780048243}, {"x"=0.30282192, "y"=0.780048243}, {"x"=0.30282192, "y"=0.780048243}, {"x"=0.30282192, "y"=0.780048243}, {"x"=0.30282192, "y"=0.780048243}, {"x"=0.30282192, "y"=0.780048243}, {"x"=0.30282192, "y"=0.780048243}, {"x"=0.30282192, "y"=0.780048243}, {"x"=0.30282192, "y"=0.780048243}, {"x"=0.30282192, "y"=0.780048243}, {"x"=0.30282192, "y"=0.780048243}, {"x"=0.30282192, "y"=0.780048243}, {"x"=0.30282192, "y"=0.780048243}, {"x"=0.30282192, "y"=0.780048243}, {"x"=0.30282192, "y"=0.780048243}, {"x"=0.30282192, "y"=0.780048243}, {"x"=0.30282192, "y"=0.780048243}, {"x"=0.30282192, "y"=0.780048243}, {"x"=0.30282192, "y"=0.780048243}, {"x"=0.30282192, "y"=0.780048243}, {"x"=0.30282192, "y"=0.780048243}, {"x"=0.30282192, "y"=0.780048243}, {"x"=0.30282192, "y"=0.780048243}, {"x"=0.30282192, "y"=0.780048243}, {"x"=0.30282192, "y"=0.780048243}, {"x"=0.30282192, "y"=0.780048243}, {"x"=0.30282192, "y"=0.780048243}, {"x"=0.30282192, "y"=0.780048243}, {"x"=0.30282192, "y"=0.780048243}, {"x"=0.30282192, "y"=0.780048243}, {"x"=0.30282192, "y"=0.780048243}, {"x"=0.30282192, "y"=0.780048243}, {"x"=0.30282192, "y"=0.780048243}, {"x"=0.30282192, "y"=0.780048243}, {"x"=0.30282192, "y"=0.780048243}, {"x"=0.30282192, "y"=0.780048243}, {"x"=0.30282192, "y"=0.780048243}, {"x"=0.30282192, "y"=0.780048243}, {"x"=0.30282192, "y"=0.780048243}, {"x"=0.30282192, "y"=0.780048243}, {"x"=0.30282192, "y"=0.780048243}, {"x"=0.30282192, "y"=0.780048243}, {"x"=0.30282192, "y"=0.780048243}, {"x"=0.30282192, "y"=0.780048243}, {"x"=0.30282192, "y"=0.780048243}, {"x"=0.30282192, "y"=0.780048243}, {"x"=0.30282192, "y"=0.780048243}, {"x"=0.30282192, "y"=0.780048243}, {"x"=0.30282192, "y"=0.780048243}, {"x"=0.30282192, "y"=0.780048243}, {"x"=0.30282192, "y"=0.780048243}, {"x"=0.30282192, "y"=0.780048243}, {"x"=0.30282192, "y"=0.780048243}, {"x"=0.30282192, "y"=0.780048243}, {"x"=0.30282192, "y"=0.780048243}, {"x"=0.30282192, "y"=0.780048243}, {"x"=0.30282192, "y"=0.780048243}, {"x"=0.30282192, "y"=0.780048243}, {"x"=0.30282192, "y"=0.780048243}, {"x"=0.30282192, "y"=0.780048243}, {"x"=0.30282192, "y"=0.780048243}, {"x"=0.30282192, "y"=0.780048243}, {"x"=0.30282192, "y"=0.780048243}, {"x"=0.30282192, "y"=0.780048243}, {"x"=0.30282192, "y"=0.780048243}, {"x"=0.30282192, "y"=0.780048243}, {"x"=0.30282192, "y"=0.780048243}, {"x"=0.30282192, "y"=0.780048243}, {"x"=0.30282192, "y"=0.780048243}, {"x"=0.30282192, "y"=0.780048243}, {"x"=0.30282192, "y"=0.780048243}, {"x"=0.30282192, "y"=0.780048243}, {"x"=0.30282192, "y"=0.780048243}, {"x"=0.30282192, "y"=0.780048243}, {"x"=0.30282192, "y"=0.780048243}, {"x"=0.30282192, "y"=0.780048243}, {"x"=0.30282192, "y"=0.780048243}, {"x"=0.30282192, "y"=0.780048243}, {"x"=0.30282192, "y"=0.780048243}, {"x"=0.30282192, "y"=0.780048243}, {"x"=0.30282192, "y"=0.780048243}, {"x"=0.30282192, "y"=0.780048243}, {"x"=0.30282192, "y"=0.780048243}, {"x"=0.30282192, "y"=0.780048243}, {"x"=0.30282192, "y"=0.780048243}, {"x"=0.30282192, "y"=0.780048243}, {"x"=0.30282192, "y"=0.780048243}, {"x"=0.30282192, "y"=0.780048243}, {"x"=0.30282192, "y"=0.780048243}, {"x"=0.30282192, "y"=0.780048243}, {"x"=0.30282192, "y"=0.780048243}, {"x"=0.30282192, "y"=0.780048243}, {"x"=0.30282192, "y"=0.780048243}, {"x"=0.30282192, "y"=0.780048243}, {"x"=0.30282192, "y"=0.780048243}, {"x"=0.30282192, "y"=0.780048243}, {"x"=0.30282192, "y"=0.780048243}, {"x"=0.30282192, "y"=0.780048243}, {"x"=0.30282192, "y"=0.780048243}, {"x"=0.30282192, "y"=0.780048243}, {"x"=0.30282192, "y"=0.780048243}, {"x"=0.30282192, "y"=0.780048243}, {"x"=0.30282192, "y"=0.780048243}, {"x"=0.30282192, "y"=0.780048243}, {"x"=0.30282192, "y"=0.780048243}, {"x"=0.30282192, "y"=0.780048243}, {"x"=0.30282192, "y"=0.780048243}, {"x"=0.30282192, "y"=0.780048243}, {"x"=0.30282192, "y"=0.780048243}, {"x"=0.30282192, "y"=0.780048243}, {"x"=0.30282192, "y"=0.780048243}, {"x"=0.30282192, "y"=0.780048243}, {"x"=0.30282192, "y"=0.780048243}, {"x"=0.30282192, "y"=0.780048243}, {"x"=0.30282192, "y"=0.780048243}, {"x"=0.30282192, "y"=0.780048243}, {"x"=0.30282192, "y"=0.780048243}, {"x"=0.30282192, "y"=0.780048243}, {"x"=0.30282192, "y"=0.780048243}, {"x"=0.30282192, "y"=0.780048243}, {"x"=0.30282192, "y"=0.780048243}, {"x"=0.30282192, "y"=0.780048243}, {"x"=0.30282192, "y"=0.780048243}, {"x"=0.30282192, "y"=0.780048243}, {"x"=0.30282192, "y"=0.780048243}, {"x"=0.30282192, "y"=0.780048243}, {"x"=0.30282192, "y"=0.780048243}, {"x"=0.30282192, "y"=0.780048243}, {"x"=0.30282192, "y"=0.780048243}, {"x"=0.30282192, "y"=0.780048243}, {"x"=0.30282192, "y"=0.780048243}, {"x"=0.30282192, "y"=0.780048243}, {"x"=0.30282192, "y"=0.780048243}, {"x"=0.30282192, "y"=0.780048243}, {"x"=0.30282192, "y"=0.780048243}, {"x"=0.30282192, "y"=0.780048243}, {"x"=0.30282192, "y"=0.780048243}, {"x"=0.30282192, "y"=0.780048243}, {"x"=0.30282192, "y"=0.780048243}, {"x"=0.30282192, "y"=0.780048243}, {"x"=0.30282192, "y"=0.780048243}, {"x"=0.30282192, "y"=0.780048243}, {"x"=0.30282192, "y"=0.780048243}, {"x"=0.30282192, "y"=0.780048243}, {"x"=0.30282192, "y"=0.780048243}, {"x"=0.30282192, "y"=0.780048243}, {"x"=0.30282192, "y"=0.780048243}, {"x"=0.30282192, "y"=0.780048243}, {"x"=0.30282192, "y"=0.780048243}, {"x"=0.30282192, "y"=0.780048243}, {"x"=0.30282192, "y"=0.780048243}, {"x"=0.30282192, "y"=0.780048243}, {"x"=0.30282192, "y"=0.780048243}, {"x"=0.30282192, "y"=0.780048243}, {"x"=0.30282192, "y"=0.780048243}, {"x"=0.30282192, "y"=0.780048243}, {"x"=0.30282192, "y"=0.780048243}, {"x"=0.30282192, "y"=0.780048243}, {"x"=0.30282192, "y"=0.780048243}, {"x"=0.30282192, "y"=0.780048243}, {"x"=0.30282192, "y"=0.780048243}, {"x"=0.30282192, "y"=0.780048243}, {"x"=0.30282192, "y"=0.780048243}, {"x"=0.30282192, "y"=0.780048243}, {"x"=0.30282192, "y"=0.780048243}, {"x"=0.30282192, "y"=0.780048243}, {"x"=0.30282192, "y"=0.780048243}, {"x"=0.30282192, "y"=0.780048243}, {"x"=0.30282192, "y"=0.780048243}, {"x"=0.30282192, "y"=0.780048243}, {"x"=0.30282192, "y"=0.780048243}, {"x"=0.30282192, "y"=0.780048243}, {"x"=0.30282192, "y"=0.780048243}, {"x"=0.30282192, "y"=0.780048243}, {"x"=0.30282192, "y"=0.780048243}, {"x"=0.30282192, "y"=0.780048243}, {"x"=0.30282192, "y"=0.780048243}, {"x"=0.30282192, "y"=0.780048243}, {"x"=0.30282192, "y"=0.780048243}, {"x"=0.30282192, "y"=0.780048243}, {"x"=0.30282192, "y"=0.780048243}, {"x"=0.30282192, "y"=0.780048243}, {"x"=0.30282192, "y"=0.780048243}, {"x"=0.30282192, "y"=0.780048243}, {"x"=0.30282192, "y"=0.780048243}, {"x"=0.30282192, "y"=0.780048243}, {"x"=0.30282192, "y"=0.780048243}, {"x"=0.30282192, "y"=0.780048243}, {"x"=0.30282192, "y"=0.780048243}, {"x"=0.30282192, "y"=0.780048243}, {"x"=0.30282192, "y"=0.780048243}, {"x"=0.30282192, "y"=0.780048243}, {"x"=0.30282192, "y"=0.780048243}, {"x"=0.30282192, "y"=0.780048243}, {"x"=0.30282192, "y"=0.780048243}, {"x"=0.30282192, "y"=0.780048243}, {"x"=0.30282192, "y"=0.780048243}, {"x"=0.30282192, "y"=0.780048243}, {"x"=0.30282192, "y"=0.780048243}, {"x"=0.30282192, "y"=0.780048243}, {"x"=0.30282192, "y"=0.780048243}, {"x"=0.30282192, "y"=0.780048243}, {"x"=0.30282192, "y"=0.780048243}, {"x"=0.30282192, "y"=0.780048243}, {"x"=0.30282192, "y"=0.780048243}, {"x"=0.30282192, "y"=0.780048243}, {"x"=0.30282192, "y"=0.780048243}, {"x"=0.30282192, "y"=0.780048243}, {"x"=0.30282192, "y"=0.780048243}, {"x"=0.30282192, "y"=0.780048243}, {"x"=0.30282192, "y"=0.780048243}, {"x"=0.30282192, "y"=0.780048243}, {"x"=0.30282192, "y"=0.780048243}, {"x"=0.30282192, "y"=0.780048243}, {"x"=0.30282192, "y"=0.780048243}, {"x"=0.30282192, "y"=0.780048243}, {"x"=0.30282192, "y"=0.780048243}, {"x"=0.30282192, "y"=0.780048243}, {"x"=0.30282192, "y"=0.780048243}, {"x"=0.30282192, "y"=0.780048243}, {"x"=0.30282192, "y"=0.780048243}, {"x"=0.30282192, "y"=0.780048243}, {"x"=0.30282192, "y"=0.780048243}, {"x"=0.30282192, "y"=0.780048243}, {"x"=0.30282192, "y"=0.780048243}, {"x"=0.30282192, "y"=0.780048243}, {"x"=0.30282192, "y"=0.780048243}, {"x"=0.30282192, "y"=0.780048243}, {"x"=0.30282192, "y"=0.780048243}, {"x"=0.30282192, "y"=0.780048243}, {"x"=0.30282192, "y"=0.780048243}, {"x"=0.30282192, "y"=0.780048243}, {"x"=0.30282192, "y"=0.780048243}, {"x"=0.30282192, "y"=0.780048243}, {"x"=0.30282192, "y"=0.780048243}, {"x"=0.30282192, "y"=0.780048243}, {"x"=0.30282192, "y"=0.780048243}, {"x"=0.30282192, "y"=0.780048243}, {"x"=0.30282192, "y"=0.780048243}, {"x"=0.30282192, "y"=0.780048243}, {"x"=0.30282192, "y"=0.780048243}, {"x"=0.30282192, "y"=0.780048243}, {"x"=0.30282192, "y"=0.780048243}, {"x"=0.30282192, "y"=0.780048243}, {"x"=0.30282192, "y"=0.780048243}, {"x"=0.30282192, "y"=0.780048243}, {"x"=0.30282192, "y"=0.780048243}, {"x"=0.30282192, "y"=0.780048243}, {"x"=0.30282192, "y"=0.780048243}, {"x"=0.30282192, "y"=0.780048243}, {"x"=0.30282192, "y"=0.780048243}, {"x"=0.30282192, "y"=0.780048243}, {"x"=0.30282192, "y"=0.780048243}, {"x"=0.30282192, "y"=0.780048243}, {"x"=0.30282192, "y"=0.780048243}, {"x"=0.30282192, "y"=0.780048243}, {"x"=0.30282192, "y"=0.780048243}, {"x"=0.30282192, "y"=0.780048243}, {"x"=0.30282192, "y"=0.780048243}, {"x"=0.30282192, "y"=0.780048243}, {"x"=0.30282192, "y"=0.780048243}, {"x"=0.30282192, "y"=0.780048243}, {"x"=0.30282192, "y"=0.780048243}, {"x"=0.30282192, "y"=0.780048243}, {"x"=0.30282192, "y"=0.780048243}, {"x"=0.30282192, "y"=0.780048243}, {"x"=0.30282192, "y"=0.780048243}, {"x"=0.30282192, "y"=0.780048243}, {"x"=0.30282192, "y"=0.780048243}, {"x"=0.30282192, "y"=0.780048243}, {"x"=0.30282192, "y"=0.780048243}, {"x"=0.30282192, "y"=0.780048243}, {"x"=0.30282192, "y"=0.780048243}, {"x"=0.30282192, "y"=0.780048243}, {"x"=0.30282192, "y"=0.780048243}, {"x"=0.30282192, "y"=0.780048243}, {"x"=0.30282192, "y"=0.780048243}, {"x"=0.30282192, "y"=0.780048243}, {"x"=0.30282192, "y"=0.780048243}, {"x"=0.30282192, "y"=0.780048243}, {"x"=0.30282192, "y"=0.780048243}, {"x"=0.30282192, "y"=0.780048243}, {"x"=0.30282192, "y"=0.780048243}, {"x"=0.30282192, "y"=0.780048243}, {"x"=0.30282192, "y"=0.780048243}, {"x"=0.30282192, "y"=0.780048243}, {"x"=0.30282192, "y"=0.780048243}, {"x"=0.30282192, "y"=0.780048243}, {"x"=0.30282192, "y"=0.780048243}, {"x"=0.30282192, "y"=0.780048243}, {"x"=0.30282192, "y"=0.780048243}, {"x"=0.30282192, "y"=0.780048243}, {"x"=0.30282192, "y"=0.780048243}, {"x"=0.30282192, "y"=0.780048243}, {"x"=0.30282192, "y"=0.780048243}, {"x"=0.30282192, "y"=0.780048243}, {"x"=0.30282192, "y"=0.780048243}, {"x"=0.30282192, "y"=0.780048243}, {"x"=0.30282192, "y"=0.780048243}, {"x"=0.30282192, "y"=0.780048243}, {"x"=0.30282192, "y"=0.780048243}, {"x"=0.30282192, "y"=0.780048243}, {"x"=0.30282192, "y"=0.780048243}, {"x"=0.30282192, "y"=0.780048243}, {"x"=0.30282192, "y"=0.780048243}, {"x"=0.30282192, "y"=0.780048243}, {"x"=0.30282192, "y"=0.780048243}, {"x"=0.30282192, "y"=0.780048243}, {"x"=0.30282192, "y"=0.780048243}, {"x"=0.30282192, "y"=0.780048243}, {"x"=0.30282192, "y"=0.780048243}, {"x"=0.30282192, "y"=0.780048243}, {"x"=0.30282192, "y"=0.780048243}, {"x"=0.30282192, "y"=0.780048243}, {"x"=0.30282192, "y"=0.780048243}, {"x"=0.30282192, "y"=0.780048243}, {"x"=0.30282192, "y"=0.780048243}, {"x"=0.30282192, "y"=0.780048243}, {"x"=0.30282192, "y"=0.780048243}, {"x"=0.30282192, "y"=0.780048243}, {"x"=0.30282192, "y"=0.780048243}, {"x"=0.30282192, "y"=0.780048243}, {"x"=0.30282192, "y"=0.780048243}, {"x"=0.30282192, "y"=0.780048243}, {"x"=0.30282192, "y"=0.780048243}, {"x"=0.30282192, "y"=0.780048243}, {"x"=0.30282192, "y"=0.780048243}, {"x"=0.30282192, "y"=0.780048243}, {"x"=0.30282192, "y"=0.780048243}, {"x"=0.30282192, "y"=0.780048243}, {"x"=0.30282192, "y"=0.780048243}, {"x"=0.30282192, "y"=0.780048243}, {"x"=0.30282192, "y"=0.780048243}, {"x"=0.30282192, "y"=0.780048243}, {"x"=0.30282192, "y"=0.780048243}, {"x"=0.30282192, "y"=0.780048243}, {"x"=0.30282192, "y"=0.780048243}, {"x"=0.30282192, "y"=0.780048243}, {"x"=0.30282192, "y"=0.780048243}, {"x"=0.30282192, "y"=0.780048243}, {"x"=0.30282192, "y"=0.780048243}, {"x"=0.30282192, "y"=0.780048243}, {"x"=0.30282192, "y"=0.780048243}, {"x"=0.30282192, "y"=0.780048243}, {"x"=0.30282192, "y"=0.780048243}, {"x"=0.30282192, "y"=0.780048243}, {"x"=0.30282192, "y"=0.780048243}, {"x"=0.30282192, "y"=0.780048243}, {"x"=0.30282192, "y"=0.780048243}, {"x"=0.30282192, "y"=0.780048243}, {"x"=0.30282192, "y"=0.780048243}, {"x"=0.30282192, "y"=0.780048243}, {"x"=0.30282192, "y"=0.780048243}, {"x"=0.30282192, "y"=0.780048243}, {"x"=0.30282192, "y"=0.780048243}, {"x"=0.30282192, "y"=0.780048243}, {"x"=0.30282192, "y"=0.780048243}, {"x"=0.30282192, "y"=0.780048243}, {"x"=0.30282192, "y"=0.780048243}, {"x"=0.30282192, "y"=0.780048243}, {"x"=0.30282192, "y"=0.780048243}, {"x"=0.30282192, "y"=0.780048243}, {"x"=0.30282192, "y"=0.780048243}, {"x"=0.30282192, "y"=0.780048243}, {"x"=0.30282192, "y"=0.780048243}, {"x"=0.30282192, "y"=0.780048243}, {"x"=0.30282192, "y"=0.780048243}, {"x"=0.30282192, "y"=0.780048243}, {"x"=0.30282192, "y"=0.780048243}, {"x"=0.30282192, "y"=0.780048243}, {"x"=0.30282192, "y"=0.780048243}, {"x"=0.30282192, "y"=0.780048243}, {"x"=0.30282192, "y"=0.780048243}, {"x"=0.30282192, "y"=0.780048243}, {"x"=0.30282192, "y"=0.780048243}, {"x"=0.30282192, "y"=0.780048243}, {"x"=0.30282192, "y"=0.780048243}, {"x"=0.30282192, "y"=0.780048243}, {"x"=0.30282192, "y"=0.780048243}, {"x"=0.30282192, "y"=0.780048243}, {"x"=0.30282192, "y"=0.780048243}, {"x"=0.30282192, "y"=0.780048243}, {"x"=0.30282192, "y"=0.780048243}, {"x"=0.30282192, "y"=0.780048243}, {"x"=0.30282192, "y"=0.780048243}, {"x"=0.30282192, "y"=0.780048243}, {"x"=0.30282192, "y"=0.780048243}, {"x"=0.30282192, "y"=0.780048243}, {"x"=0.30282192, "y"=0.780048243}, {"x"=0.30282192, "y"=0.780048243}, {"x"=0.30282192, "y"=0.780048243}, {"x"=0.30282192, "y"=0.780048243}, {"x"=0.30282192, "y"=0.780048243}, {"x"=0.30282192, "y"=0.780048243}, {"x"=0.30282192, "y"=0.780048243}, {"x"=0.30282192, "y"=0.780048243}, {"x"=0.30282192, "y"=0.780048243}, {"x"=0.30282192, "y"=0.780048243}, {"x"=0.30282192, "y"=0.780048243}, {"x"=0.30282192, "y"=0.780048243}, {"x"=0.30282192, "y"=0.780048243}, {"x"=0.30282192, "y"=0.780048243}, {"x"=0.30282192, "y"=0.780048243}, {"x"=0.30282192, "y"=0.780048243}, {"x"=0.30282192, "y"=0.780048243}, {"x"=0.30282192, "y"=0.780048243}, {"x"=0.30282192, "y"=0.780048243}, {"x"=0.30282192, "y"=0.780048243}, {"x"=0.30282192, "y"=0.780048243}, {"x"=0.30282192, "y"=0.780048243}, {"x"=0.30282192, "y"=0.780048243}, {"x"=0.30282192, "y"=0.780048243}, {"x"=0.30282192, "y"=0.780048243}, {"x"=0.30282192, "y"=0.780048243}, {"x"=0.30282192, "y"=0.780048243}, {"x"=0.30282192, "y"=0.780048243}, {"x"=0.30282192, "y"=0.780048243}, {"x"=0.30282192, "y"=0.780048243}, {"x"=0.30282192, "y"=0.780048243}, {"x"=0.30282192, "y"=0.780048243}, {"x"=0.30282192, "y"=0.780048243}, {"x"=0.30282192, "y"=0.780048243}, {"x"=0.30282192, "y"=0.780048243}, {"x"=0.30282192, "y"=0.780048243}, {"x"=0.30282192, "y"=0.780048243}, {"x"=0.30282192, "y"=0.780048243}, {"x"=0.30282192, "y"=0.780048243}, {"x"=0.30282192, "y"=0.780048243}, {"x"=0.30282192, "y"=0.780048243}, {"x"=0.30282192, "y"=0.780048243}, {"x"=0.30282192, "y"=0.780048243}, {"x"=0.30282192, "y"=0.780048243}, {"x"=0.30282192, "y"=0.780048243}, {"x"=0.30282192, "y"=0.780048243}, {"x"=0.30282192, "y"=0.780048243}, {"x"=0.30282192, "y"=0.780048243}, {"x"=0.30282192, "y"=0.780048243}, {"x"=0.30282192, "y"=0.780048243}, {"x"=0.30282192, "y"=0.780048243}, {"x"=0.30282192, "y"=0.780048243}, {"x"=0.30282192, "y"=0.780048243}, {"x"=0.30282192, "y"=0.780048243}, {"x"=0.30282192, "y"=0.780048243}, {"x"=0.30282192, "y"=0.780048243}, {"x"=0.30282192, "y"=0.780048243}, {"x"=0.30282192, "y"=0.780048243}, {"x"=0.30282192, "y"=0.780048243}, {"x"=0.30282192, "y"=0.780048243}, {"x"=0.30282192, "y"=0.780048243}, {"x"=0.30282192, "y"=0.780048243}, {"x"=0.30282192, "y"=0.780048243}, {"x"=0.30282192, "y"=0.780048243}, {"x"=0.30282192, "y"=0.780048243}, {"x"=0.30282192, "y"=0.780048243}, {"x"=0.30282192, "y"=0.780048243}, {"x"=0.30282192, "y"=0.780048243}, {"x"=0.30282192, "y"=0.780048243}, {"x"=0.30282192, "y"=0.780048243}, {"x"=0.30282192, "y"=0.780048243}, {"x"=0.30282192, "y"=0.780048243}, {"x"=0.30282192, "y"=0.780048243}, {"x"=0.30282192, "y"=0.780048243}, {"x"=0.30282192, "y"=0.780048243}, {"x"=0.30282192, "y"=0.780048243}, {"x"=0.30282192, "y"=0.780048243}, {"x"=0.30282192, "y"=0.780048243}, {"x"=0.30282192, "y"=0.780048243}, {"x"=0.30282192, "y"=0.780048243}, {"x"=0.30282192, "y"=0.780048243}, {"x"=0.30282192, "y"=0.780048243}, {"x"=0.30282192, "y"=0.780048243}, {"x"=0.30282192, "y"=0.780048243}, {"x"=0.30282192, "y"=0.780048243}, {"x"=0.30282192, "y"=0.780048243}, {"x"=0.30282192, "y"=0.780048243}, {"x"=0.30282192, "y"=0.780048243}, {"x"=0.30282192, "y"=0.780048243}, {"x"=0.30282192, "y"=0.780048243}, {"x"=0.30282192, "y"=0.780048243}, {"x"=0.30282192, "y"=0.780048243}, {"x"=0.30282192, "y"=0.780048243}, {"x"=0.30282192, "y"=0.780048243}, {"x"=0.30282192, "y"=0.780048243}, {"x"=0.30282192, "y"=0.780048243}, {"x"=0.30282192, "y"=0.780048243}, {"x"=0.30282192, "y"=0.780048243}, {"x"=0.30282192, "y"=0.780048243}, {"x"=0.30282192, "y"=0.780048243}, {"x"=0.30282192, "y"=0.780048243}, {"x"=0.30282192, "y"=0.780048243}, {"x"=0.30282192, "y"=0.780048243}, {"x"=0.30282192, "y"=0.780048243}, {"x"=0.30282192, "y"=0.780048243}, {"x"=0.30282192, "y"=0.780048243}, {"x"=0.30282192, "y"=0.780048243}, {"x"=0.30282192, "y"=0.780048243}, {"x"=0.30282192, "y"=0.780048243}, {"x"=0.30282192, "y"=0.780048243}, {"x"=0.30282192, "y"=0.780048243}, {"x"=0.30282192, "y"=0.780048243}, {"x"=0.30282192, "y"=0.780048243}, {"x"=0.30282192, "y"=0.780048243}, {"x"=0.30282192, "y"=0.780048243}, {"x"=0.30282192, "y"=0.780048243}, {"x"=0.30282192, "y"=0.780048243}, {"x"=0.30282192, "y"=0.780048243}, {"x"=0.30282192, "y"=0.780048243}, {"x"=0.30282192, "y"=0.780048243}, {"x"=0.30282192, "y"=0.780048243}, {"x"=0.30282192, "y"=0.780048243}, {"x"=0.30282192, "y"=0.780048243}, {"x"=0.30282192, "y"=0.780048243}, {"x"=0.30282192, "y"=0.780048243}, {"x"=0.30282192, "y"=0.780048243}, {"x"=0.30282192, "y"=0.780048243}, {"x"=0.30282192, "y"=0.780048243}, {"x"=0.30282192, "y"=0.780048243}, {"x"=0.30282192, "y"=0.780048243}, {"x"=0.30282192, "y"=0.780048243}, {"x"=0.30282192, "y"=0.780048243}, {"x"=0.30282192, "y"=0.780048243}, {"x"=0.30282192, "y"=0.780048243}, {"x"=0.30282192, "y"=0.780048243}, {"x"=0.30282192, "y"=0.780048243}, {"x"=0.30282192, "y"=0.780048243}, {"x"=0.30282192, "y"=0.780048243}, {"x"=0.30282192, "y"=0.780048243}, {"x"=0.30282192, "y"=0.780048243}, {"x"=0.30282192, "y"=0.780048243}, {"x"=0.30282192, "y"=0.780048243}, {"x"=0.30282192, "y"=0.780048243}, {"x"=0.30282192, "y"=0.780048243}, {"x"=0.30282192, "y"=0.780048243}, {"x"=0.30282192, "y"=0.780048243}, {"x"=0.30282192, "y"=0.780048243}, {"x"=0.30282192, "y"=0.780048243}, {"x"=0.30282192, "y"=0.780048243}, {"x"=0.30282192, "y"=0.780048243}, {"x"=0.30282192, "y"=0.780048243}, {"x"=0.30282192, "y"=0.780048243}, {"x"=0.30282192, "y"=0.780048243}, {"x"=0.30282192, "y"=0.780048243}, {"x"=0.30282192, "y"=0.780048243}, {"x"=0.30282192, "y"=0.780048243}, {"x"=0.30282192, "y"=0.780048243}, {"x"=0.30282192, "y"=0.780048243}, {"x"=0.30282192, "y"=0.780048243}, {"x"=0.30282192, "y"=0.780048243}, {"x"=0.30282192, "y"=0.780048243}, {"x"=0.30282192, "y"=0.780048243}, {"x"=0.30282192, "y"=0.780048243}, {"x"=0.30282192, "y"=0.780048243}, {"x"=0.30282192, "y"=0.780048243}, {"x"=0.30282192, "y"=0.780048243}, {"x"=0.30282192, "y"=0.780048243}, {"x"=0.30282192, "y"=0.780048243}, {"x"=0.30282192, "y"=0.780048243}, {"x"=0.30282192, "y"=0.780048243}, {"x"=0.30282192, "y"=0.780048243}, {"x"=0.30282192, "y"=0.780048243}, {"x"=0.30282192, "y"=0.780048243}, {"x"=0.30282192, "y"=0.780048243}, {"x"=0.30282192, "y"=0.780048243}, {"x"=0.30282192, "y"=0.780048243}, {"x"=0.30282192, "y"=0.780048243}, {"x"=0.30282192, "y"=0.780048243}, {"x"=0.30282192, "y"=0.780048243}, {"x"=0.30282192, "y"=0.780048243}, {"x"=0.30282192, "y"=0.780048243}, {"x"=0.30282192, "y"=0.780048243}, {"x"=0.30282192, "y"=0.780048243}, {"x"=0.30282192, "y"=0.780048243}, {"x"=0.30282192, "y"=0.780048243}, {"x"=0.30282192, "y"=0.780048243}, {"x"=0.30282192, "y"=0.780048243}, {"x"=0.30282192, "y"=0.780048243}, {"x"=0.30282192, "y"=0.780048243}, {"x"=0.30282192, "y"=0.780048243}, {"x"=0.30282192, "y"=0.780048243}, {"x"=0.30282192, "y"=0.780048243}, {"x"=0.30282192, "y"=0.780048243}, {"x"=0.30282192, "y"=0.780048243}, {"x"=0.30282192, "y"=0.780048243}, {"x"=0.30282192, "y"=0.780048243}, {"x"=0.30282192, "y"=0.780048243}, {"x"=0.30282192, "y"=0.780048243}, {"x"=0.30282192, "y"=0.780048243}, {"x"=0.30282192, "y"=0.780048243}, {"x"=0.30282192, "y"=0.780048243}, {"x"=0.30282192, "y"=0.780048243}, {"x"=0.30282192, "y"=0.780048243}, {"x"=0.30282192, "y"=0.780048243}, {"x"=0.30282192, "y"=0.780048243}, {"x"=0.30282192, "y"=0.780048243}, {"x"=0.30282192, "y"=0.780048243}, {"x"=0.30282192, "y"=0.780048243}, {"x"=0.30282192, "y"=0.780048243}, {"x"=0.30282192, "y"=0.780048243}, {"x"=0.30282192, "y"=0.780048243}, {"x"=0.30282192, "y"=0.780048243}, {"x"=0.30282192, "y"=0.780048243}, {"x"=0.30282192, "y"=0.780048243}, {"x"=0.30282192, "y"=0.780048243}, {"x"=0.30282192, "y"=0.780048243}, {"x"=0.30282192, "y"=0.780048243}, {"x"=0.30282192, "y"=0.780048243}, {"x"=0.30282192, "y"=0.780048243}, {"x"=0.30282192, "y"=0.780048243}, {"x"=0.30282192, "y"=0.780048243}, {"x"=0.30282192, "y"=0.780048243}, {"x"=0.30282192, "y"=0.780048243}, {"x"=0.30282192, "y"=0.780048243}, {"x"=0.30282192, "y"=0.780048243}, {"x"=0.30282192, "y"=0.780048243}, {"x"=0.30282192, "y"=0.780048243}, {"x"=0.30282192, "y"=0.780048243}, {"x"=0.30282192, "y"=0.780048243}, {"x"=0.30282192, "y"=0.780048243}, {"x"=0.30282192, "y"=0.780048243}, {"x"=0.30282192, "y"=0.780048243}, {"x"=0.30282192, "y"=0.780048243}, {"x"=0.30282192, "y"=0.780048243}, {"x"=0.30282192, "y"=0.780048243}, {"x"=0.30282192, "y"=0.780048243}, {"x"=0.30282192, "y"=0.780048243}, {"x"=0.30282192, "y"=0.780048243}, {"x"=0.30282192, "y"=0.780048243}, {"x"=0.30282192, "y"=0.780048243}, {"x"=0.30282192, "y"=0.780048243}, {"x"=0.30282192, "y"=0.780048243}, {"x"=0.30282192, "y"=0.780048243}, {"x"=0.30282192, "y"=0.780048243}, {"x"=0.30282192, "y"=0.780048243}, {"x"=0.30282192, "y"=0.780048243}, {"x"=0.30282192, "y"=0.780048243}, {"x"=0.30282192, "y"=0.780048243}, {"x"=0.30282192, "y"=0.780048243}, {"x"=0.30282192, "y"=0.780048243}, {"x"=0.30282192, "y"=0.780048243}, {"x"=0.30282192, "y"=0.780048243}, {"x"=0.30282192, "y"=0.780048243}, {"x"=0.30282192, "y"=0.780048243}, {"x"=0.30282192, "y"=0.780048243}, {"x"=0.30282192, "y"=0.780048243}, {"x"=0.30282192, "y"=0.780048243}, {"x"=0.30282192, "y"=0.780048243}, {"x"=0.30282192, "y"=0.780048243}, {"x"=0.30282192, "y"=0.780048243}, {"x"=0.30282192, "y"=0.780048243}, {"x"=0.30282192, "y"=0.780048243}, {"x"=0.30282192, "y"=0.780048243}, {"x"=0.30282192, "y"=0.780048243}, {"x"=0.30282192, "y"=0.780048243}, {"x"=0.30282192, "y"=0.780048243}, {"x"=0.30282192, "y"=0.780048243}, {"x"=0.30282192, "y"=0.780048243}, {"x"=0.30282192, "y"=0.780048243}, {"x"=0.30282192, "y"=0.780048243}, {"x"=0.30282192, "y"=0.780048243}, {"x"=0.30282192, "y"=0.780048243}, {"x"=0.30282192, "y"=0.780048243}, {"x"=0.30282192, "y"=0.780048243}, {"x"=0.30282192, "y"=0.780048243}, {"x"=0.30282192, "y"=0.780048243}, {"x"=0.30282192, "y"=0.780048243}, {"x"=0.30282192, "y"=0.780048243}, {"x"=0.30282192, "y"=0.780048243}, {"x"=0.30282192, "y"=0.780048243}, {"x"=0.30282192, "y"=0.780048243}, {"x"=0.30282192, "y"=0.780048243}, {"x"=0.30282192, "y"=0.780048243}, {"x"=0.30282192, "y"=0.780048243}, {"x"=0.30282192, "y"=0.780048243}, {"x"=0.30282192, "y"=0.780048243}, {"x"=0.30282192, "y"=0.780048243}, {"x"=0.30282192, "y"=0.780048243}, {"x"=0.30282192, "y"=0.780048243}, {"x"=0.30282192, "y"=0.780048243}, {"x"=0.30282192, "y"=0.780048243}, {"x"=0.30282192, "y"=0.780048243}, {"x"=0.30282192, "y"=0.780048243}, {"x"=0.30282192, "y"=0.780048243}, {"x"=0.30282192, "y"=0.780048243}, {"x"=0.30282192, "y"=0.780048243}, {"x"=0.30282192, "y"=0.780048243}, {"x"=0.30282192, "y"=0.780048243}, {"x"=0.30282192, "y"=0.780048243}, {"x"=0.30282192, "y"=0.780048243}, {"x"=0.30282192, "y"=0.780048243}, {"x"=0.30282192, "y"=0.780048243}, {"x"=0.30282192, "y"=0.780048243}, {"x"=0.30282192, "y"=0.780048243}, {"x"=0.30282192, "y"=0.780048243}, {"x"=0.30282192, "y"=0.780048243}, {"x"=0.30282192, "y"=0.780048243}, {"x"=0.30282192, "y"=0.780048243}, {"x"=0.30282192, "y"=0.780048243}, {"x"=0.30282192, "y"=0.780048243}, {"x"=0.30282192, "y"=0.780048243}, {"x"=0.30282192, "y"=0.780048243}, {"x"=0.30282192, "y"=0.780048243}, {"x"=0.30282192, "y"=0.780048243}, {"x"=0.30282192, "y"=0.780048243}, {"x"=0.30282192, "y"=0.780048243}, {"x"=0.30282192, "y"=0.780048243}, {"x"=0.30282192, "y"=0.780048243}, {"x"=0.30282192, "y"=0.780048243}, {"x"=0.30282192, "y"=0.780048243}, {"x"=0.30282192, "y"=0.780048243}, {"x"=0.30282192, "y"=0.780048243}, {"x"=0.30282192, "y"=0.780048243}, {"x"=0.30282192, "y"=0.780048243}, {"x"=0.30282192, "y"=0.780048243}, {"x"=0.30282192, "y"=0.780048243}, {"x"=0.30282192, "y"=0.780048243}, {"x"=0.30282192, "y"=0.780048243}, {"x"=0.30282192, "y"=0.780048243}, {"x"=0.30282192, "y"=0.780048243}, {"x"=0.30282192, "y"=0.780048243}, {"x"=0.30282192, "y"=0.780048243}, {"x"=0.30282192, "y"=0.780048243}, {"x"=0.30282192, "y"=0.780048243}, {"x"=0.30282192, "y"=0.780048243}, {"x"=0.30282192, "y"=0.780048243}, {"x"=0.30282192, "y"=0.780048243}, {"x"=0.30282192, "y"=0.780048243}, {"x"=0.30282192, "y"=0.780048243}, {"x"=0.30282192, "y"=0.780048243}, {"x"=0.30282192, "y"=0.780048243}]
  in  "max_gain":T6(ring)=enum."10^11 High speed"
  in  "Range_switch_delay":u32=100
  out "LIA2_DMM_chart":dbl(graph)=0.171521931
  out "LIA1_DMM_chart":dbl(graph)=0.0890152763
  out "Sample Conductance (slave)":dbl(graph)=3.282477414397079e-08
  out "Acquired Data":string="-2.441745E+8;6.302685E-9;0.000000E+0;2.047763E+12"
  out "IV Comment":string="Data_Points   O/C_Cyles  Motor_Pos  lockin_phase  Temperature Voltage_drop LockAmpl timeLIA1 timeLIA2   OC_timestamp \r662500\t162\t-213699152\t90\t9.546\t45\t4\t9\t9\tH:25:52,4278\t"
  out "34401 range read":string="+1.00000000E+01\n"
  out "Delta MP":T7=-396067365
  out "# Errors":u16
  out "sample Temperature":dbl(graph)=16.442
  in  "Array size":i16=20
  out "CV":dbl(graph)=0.3740831552508511
  in  "CV _ Value":dbl=0.415
  out "cond array last 10":dbl[](array[numeric])=[9.654340139697067e-09, 1.320559420051316e-08, 8.837437385608568e-09, 1.6618852247786115e-08, 1.6316719224485995e-08, 1.6842461386011378e-08, 5.90070540600802e-09, 1.2460448687652757e-08, 1.2265786084019354e-08, 8.78458980378888e-09, 6.730649478763007e-09, 7.04468631417935e-09, 8.182326425719535e-09, 6.488679100132683e-09, 1.771263421519368e-08, 1.7904465482821712e-08, 1.1616211013874701e-08, 7.148327156326288e-09, 6.723558382028771e-09, 1.3097055427322855e-08]
  out "CV 2":dbl=0.3740831552508511
  in  "Apply SP":bool
  in  "Update Motor Position":bool
  in  "Abort Motion":bool
  in  "Reset":bool
  in  "Maximum Motor Velocity":u16(slide)=4500 min=200 max=5000 step=10 scale=200.0..5000.0
  in  "Rel. Move":bool
  in  "Calibration Factor (#counts / nm)":dbl=20000000.0 format="%#.0g"
  in  "Distance Increment [nm]":dbl
  in  "Motor Position Increment [counts]":i32=2000
  in  "Relative Move Mode":T8(radio)
  in  "Abs. Move":bool
  in  "New Motor Position":i32=4000 min=-1800000000 max=1800000000 step=1000
  in  "bias_in_loop":dbl=0.1 format="%#_7g"
  in  "Bias_set_in_loop":bool
  in  "Bias_pol_inloop":bool=TRUE
  in  "Femto_Index":i32=1
  in  "LIA1_DMM_VISA":refnum<visa-resource-name>="USB0::0x2A8D::0x1401::MY59000923::INSTR"
  in  "VISA Resource MC":refnum<visa-resource-name>="COM1"
  in  "Agilent 34410A":refnum<visa-resource-name>="GPIB0::10::INSTR"
  out "Error MC":errorcluster
  out "Error SMU":errorcluster
  in  "LIA2_DMM_VISA":refnum<visa-resource-name>="USB0::0x2A8D::0x1401::MY57230853::INSTR"
  in  "DMM_6500_VISA":refnum<visa-resource-name>="USB0::0x05E6::0x6500::04446089::INSTR"
  in  "Yokogawa 7651":refnum<visa-resource-name>="GPIB0::13::INSTR"
  in  "VISA LIA1":refnum<visa-resource-name>="GPIB0::8::INSTR"
  in  "VISA  LIA2":refnum<visa-resource-name>="GPIB0::20::INSTR"
  in  "tempcontrl visa":refnum<visa-resource-name>="GPIB0::12::INSTR"
  out "Femto status":i32=1
  out "Status_out":i32=6
  out "index_out":i32=1
  in  "Label Filenames o/c/n":bool
  out "LabVIEW\nTimeStamp":timestamp=timestamp(3707354373.917821 s since 1904-01-01)
  out "Activate_Femto":bool=TRUE
  # "Motor Settings"
  # "OC Mode"
  # "High - Low R Mode"
  # "Emergency Abort Conditions (Motor Stop)"
  # "Lock in Setting"
  # "IV Settings"
  # "DMM Options"
  # "Absolute Positioning (LA)"
  # "Speed Limit (SP)"
  # "Zero Motor Position (HO)"
  # "Relative Positioning (LR)"
  # "Update Motor Position (POS, GN)"
  # "Abort Motion / Emergency Off (DI)"
  # "VISA Settings"
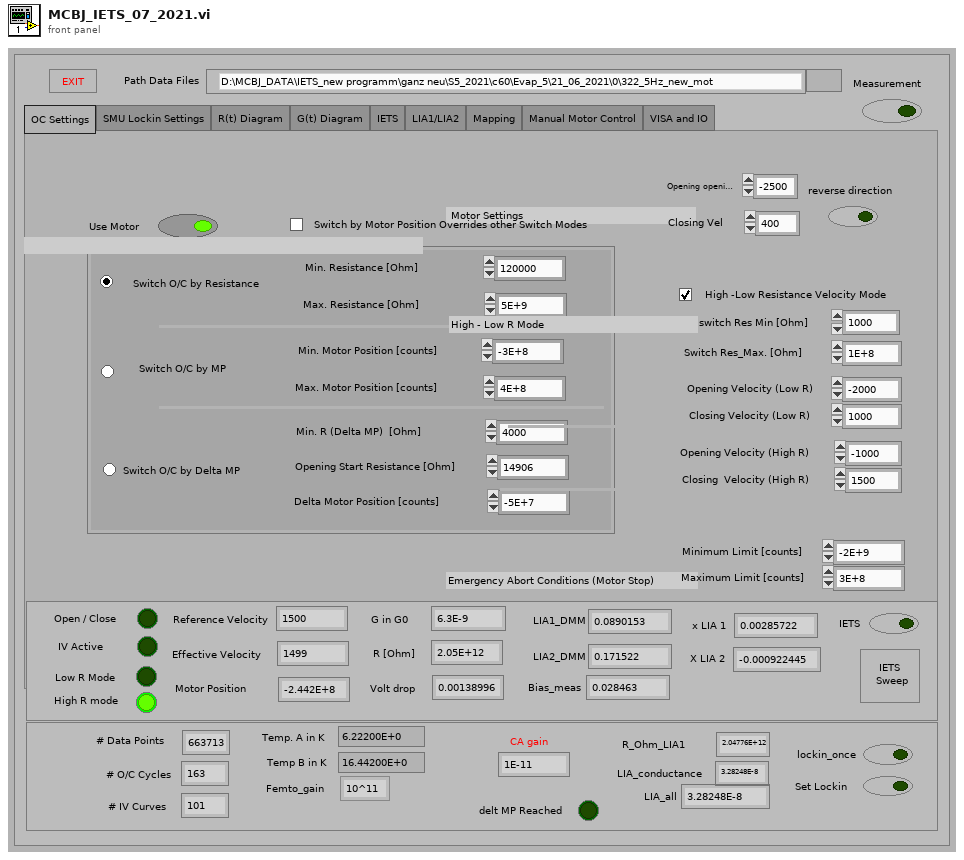
[diagram p1: front panel]
types:
  T1 = enum16{"10^3", "10^4", "10^5", "10^6", "10^7", "10^8", "10^9", "10^10", "10^11"}
  T2 = enum32{"OC Settings", "SMU Lockin Settings", "R(t) Diagram", "G(t) Diagram", "IETS", "LIA1/LIA2", "Mapping", "Manual Motor Control", "VISA and IO"}
  T3 = enum32{"Switch O/C by Resistance", "Switch O/C by MP", "Switch O/C by Delta MP"}
  T4 = enum16{"10mV", "100mV", "1V", "10V", "30V", "1mA", "10mA", "100mA"}
  T5 = enum16{"10^4", "10^5", "10^6", "10^7", "10^8", "10^9", "10^10", "10^11", "10^12", "10^13"}
  T6 = enum16{"10^3 Low noise", "10^4 Low noise", "10^5 Low noise", "10^6 Low noise", "10^7 Low noise", "10^8 Low noise", "10^9 Low noise", "10^10 High speed", "10^11 High speed"}
  T7 = typedef "for autom measure somehowControl 2.ctl" = i32
  T8 = enum32{"Move by Motor Counts", "Move by Electrode Distance"}
  T9 = typedef "FEMTO_LUCI-10.lvlib/Choose_Device_Enum.ctl" = enum16{"DDPCA-300", "DLPCA-200", "DHPCA-100", "OE-200", "OE-300", "LIA-MV-150-S", "LIA-MV-150-D", "LIA-MV-200-L", "LIA-MV-200-H", "LIA-MVD-200-L", "LIA-MVD-200-H", "DLPVA-100-BUN-S", "DLPVA-100-BLN-S", "DLPVA-100-B-S", "DLPVA-100-B-D", "DLPVA-100-F-S", "DLPVA-100-F-D", "DHPVA-100", "DHPVA-200", "DUPVA-1-60", "DUPVA-1-70"}
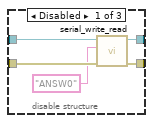
[diagram p2: hidden frame]
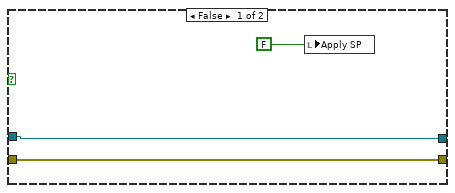
[diagram p4: hidden frame]
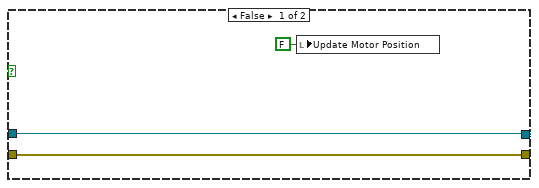
[diagram p5: hidden frame]
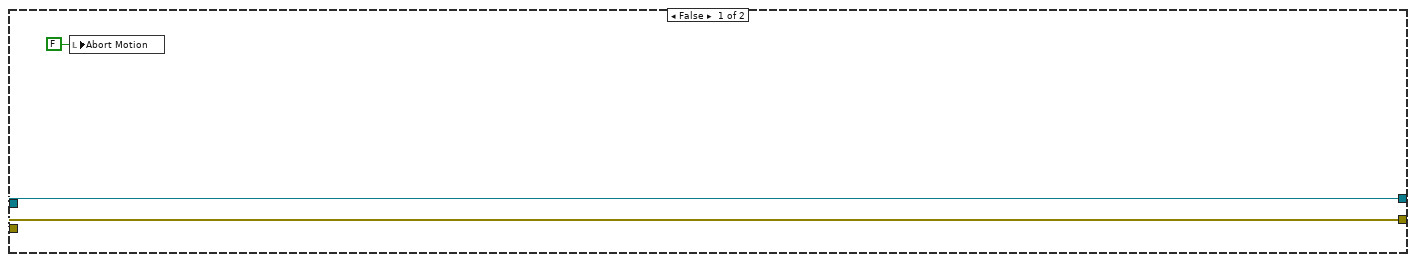
[diagram p6: hidden frame]
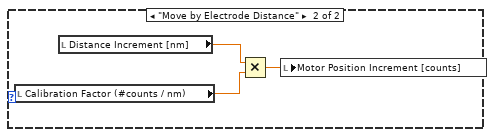
[diagram p7: hidden frame]
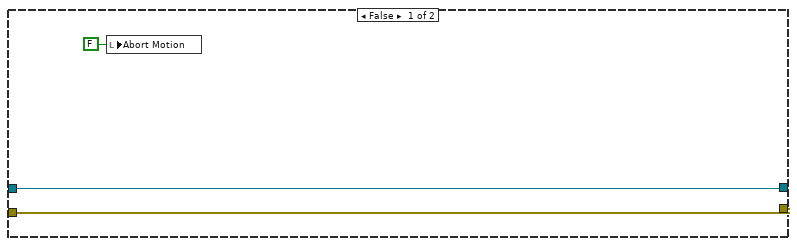
[diagram p9: hidden frame]
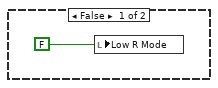
[diagram p13: hidden frame]
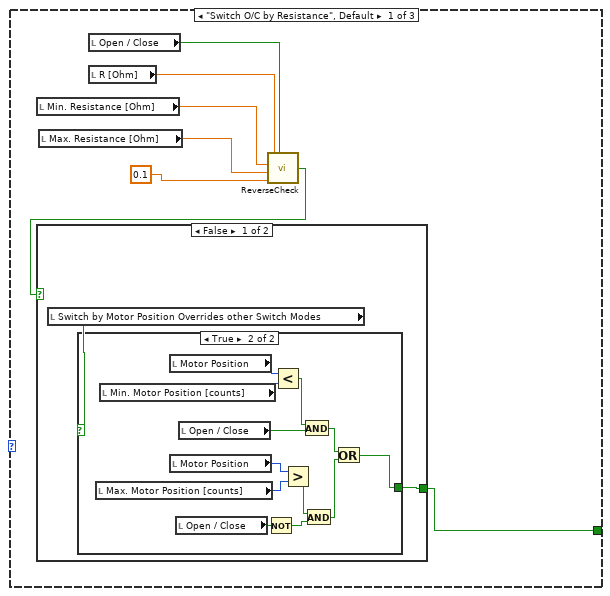
[diagram p14: hidden frame]
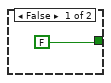
[diagram p15: hidden frame]
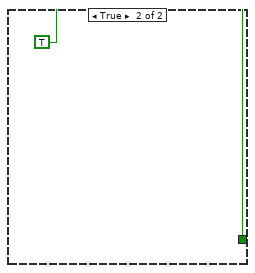
[diagram p16: hidden frame]
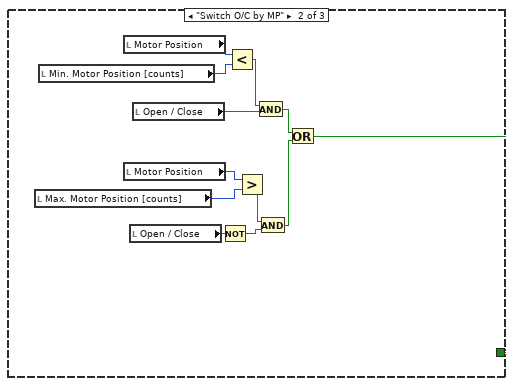
[diagram p17: hidden frame]
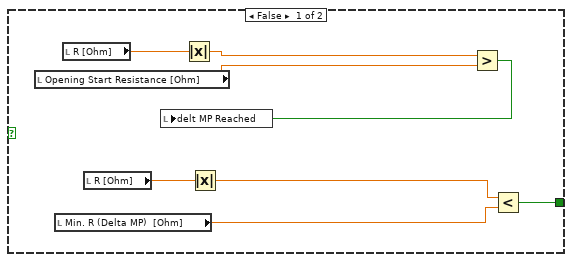
[diagram p18: hidden frame]
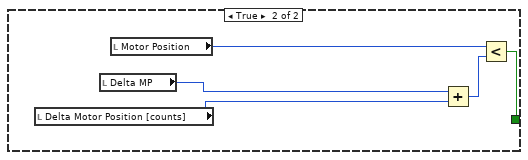
[diagram p20: hidden frame]
diagram:
  n1 = flat-sequence {
    tunnel: [w33] -> w20
    tunnel: [w34] -> w16
    tunnel: [w63] -> w14
    tunnel: [w62] -> w13
    tunnel: [w39] -> w12
    tunnel: [w40] -> w11
    tunnel: [w37] -> w10
    tunnel: [w38] -> w9
    tunnel: [w52] -> w4
    tunnel: [w51] -> w3
    tunnel: w20 -> [w98]
    tunnel: [w97] -> w19
    tunnel: [w96] -> w18
    tunnel: [w95] -> w17
    tunnel: w16 -> [w94]
    tunnel: [w93] -> w15
    tunnel: w14 -> [w92]
    tunnel: w13 -> [w91]
    tunnel: w12 -> [w81]
    tunnel: w11 -> [w82]
    tunnel: w10 -> [w80]
    tunnel: w9 -> [w79]
    tunnel: [w90] -> w8
    tunnel: [w89] -> w7
    tunnel: [w88] -> w6
    tunnel: [w87] -> w5
    tunnel: w4 -> [w86]
    tunnel: w3 -> [w85]
    tunnel: [w84] -> w1
    tunnel: [w83] -> w2
    tunnel: w19 -> [w1440]
    tunnel: w18 -> [w1447]
    tunnel: w17 -> [w1446]
    tunnel: w15 -> [w1441]
    tunnel: w8 -> [w1438]
    tunnel: w7 -> [w1437]
    tunnel: w6 -> [w1436]
    tunnel: w5 -> [w1435]
    frame #0 {
      w22 = 3 items=["Current DC", "Resistance", "Temperature", "Voltage DC"] ("Zero Type (0: Current DC)")
      w21 = u16 2 items=["On", "Off", "Once"] ("Autozero  (0: On)")
      w28 = errorcluster {"status"=FALSE, "code"=0, "source"=""} ("error constant")
      # "Controls and Variables"
      # "Motion Controller"
      # "KE 2000"
      # "Initialization"
      n2 = VISA Close(VISA resource name="VISA Resource MC") -> (error out=w47:errorcluster)  [unwired: 1 in]
      n3 = call <vilib>:"Clear Errors.vi"("error in (no error)"=w47) -> ("error out"=w49:errorcluster)  [unwired: 5 in, 1 out]
      n4 = call "Initialize.vi"("error in (no error)"=errorcluster {"status"=FALSE, "code"=0, "source"=""} ("Fehler (Eingang, kein Fehler)"), "VISA resource name"="Agilent 34410A") -> ("error out"=w35:errorcluster, "VISA resource name out"=w36:refnum<visa-resource-name>)  [unwired: 8 in]
      n5 = call "Initialize.vi"("error in (no error)"=w28, "VISA resource name"="DMM_6500_VISA") -> ("error out"=w23:errorcluster, "VISA resource name out"=w24:refnum<visa-resource-name>)  [unwired: 8 in]
      n6 = local write "# Errors"(u16 0 ("# Errors")) -> ()
      n7 = call "Initialize.vi"("error in (no error)"=w28, "VISA resource name"="LIA2_DMM_VISA") -> ("error out"=w30:errorcluster, "VISA resource name out"=w29:refnum<visa-resource-name>)  [unwired: 8 in]
      n8 = call "Initialize.vi"("error in (no error)"=w28, "VISA resource name"="LIA1_DMM_VISA") -> ("error out"=w31:errorcluster, "VISA resource name out"=w32:refnum<visa-resource-name>)  [unwired: 8 in]
      n9 = call "Configure Autozero.vi"("Auto Zero (0: Enable)"=w21, "error in (no error)"=w23, "Function (0: Voltage DC)"=w22, "VISA resource name"=w24) -> ()  [unwired: 6 in, 2 out]
      n10 = call-poly "VISA Configure Serial Port"("VISA resource name"="VISA Resource MC", "Enable Termination\nChar (T)"=TRUE ("Enable Termination\nChar (T)"), "baud rate (9600)"=57600, "error in (no error)"=w49) -> ("VISA resource name out"=w45:refnum<visa-resource-name>, "error out"=w48:errorcluster)  [unwired: 10 in]
      n11 = call "Configure Autozero.vi"("error in (no error)"=w35, "Autozero  (0: On)"=w21, "VISA resource name"=w36) -> ("error out"=w33:errorcluster, "VISA resource name out"=w34:refnum<visa-resource-name>)  [unwired: 7 in]
      n12 = call "Auto Zero.vi"("error in (no error)"=w30, "Auto Zero (1: Enable)"=w21, "Zero Type (0: Current DC)"=w22, "VISA resource name"=w29) -> ()  [unwired: 6 in, 2 out]
      n13 = call "Auto Zero.vi"("error in (no error)"=w31, "Auto Zero (1: Enable)"=w21, "Zero Type (0: Current DC)"=w22, "VISA resource name"=w32) -> ()  [unwired: 6 in, 2 out]
      n14 = VISA Open ("VISA: Öffnen")(error in (no error)=w48, VISA resource name=w45) -> (VISA resource name=w43:refnum<visa-resource-name>, error out=w44:errorcluster)  [unwired: 3 in]
      n15 = disable-structure shown="Enabled" {
        disable-tunnel: w44 -> [w71 w76 w77]
        disable-tunnel: w43 -> [w70 w75 w78]
        disable-tunnel: [w68 w73 w77] -> w41
        disable-tunnel: [w67 w72 w78] -> w42
        frame Disabled {
          n16 = call "serial_write_read.vi"("error in (no error)"=w71, "command"="ANSW0" ("write buffer"), "VISA resource name"=w70) -> ("error out"=w68:errorcluster, "VISA resource name out"=w67:refnum<visa-resource-name>)  [unwired: 6 in, 1 out]
        }
        frame Enabled {
          n17 = call "serial_write_read.vi"("error in (no error)"=w76, "command"="ANSW2" ("write buffer"), "VISA resource name"=w75) -> ("error out"=w73:errorcluster, "VISA resource name out"=w72:refnum<visa-resource-name>)  [unwired: 6 in, 1 out]
        }
        frame Disabled {
        }
      }
      n18 = call "Initialize.vi"("error in (no error)"=errorcluster {"status"=FALSE, "code"=0, "source"=""} ("Fehler (Eingang, kein Fehler)"), "VISA resource name"="VISA  LIA2") -> ("error out"=w38:errorcluster, "VISA resource name out"=w37:refnum<visa-resource-name>)  [unwired: 8 in]
      n19 = call "Initialize.vi"("error in (no error)"=errorcluster {"status"=FALSE, "code"=0, "source"=""} ("Fehler (Eingang, kein Fehler)"), "VISA resource name"="VISA LIA1") -> ("error out"=w39:errorcluster, "VISA resource name out"=w40:refnum<visa-resource-name>)  [unwired: 8 in]
      n20 = call "ReadMotorPosition_new_thatec.vi"("VISA resource name (output) 2"=w42, "error in (no error) (output)"=w41) -> ("VISA resource name (output)"=w63:refnum<visa-resource-name>, "position"=w64:i32, "error out"=w62:errorcluster)  [unwired: 1 in]
      n21 = local write "Stop"(FALSE) -> ()
      n22 = local write "Motor Position"(w64) -> ()
      n23 = local write "Error MC"(w62) -> ()
      n24 = call "Initialize.vi"("VISA resource name"="tempcontrl visa", "error in (no error)"=errorcluster {"status"=FALSE, "code"=0, "source"=""} ("Fehler (Eingang, kein Fehler)")) -> ("VISA resource name out"=w52:refnum<visa-resource-name>, "error out"=w51:errorcluster)  [unwired: 12 in]
    }
    frame #1 {
      # "Experimental Procedure"
      n25 = while {
        tunnel: w98 -> [w108]
        tunnel: [w134] -> w97
        tunnel: [w133] -> w96
        tunnel: [w132] -> w95
        tunnel: w94 -> [w109]
        tunnel: [w131] -> w93
        tunnel: w92 -> [w122]
        tunnel: w91 -> [w121]
        tunnel: w81 -> [w112]
        tunnel: w82 -> [w99]
        tunnel: w80 -> [w111]
        tunnel: w79 -> [w110]
        tunnel: [w107] -> w90
        tunnel: [w106] -> w89
        tunnel: [w105] -> w88
        tunnel: [w104] -> w87
        tunnel: w86 -> [w103]
        tunnel: w85 -> [w102]
        tunnel: [w101] -> w84
        tunnel: [w100] -> w83
        stop <- w135 continue-if-true
        n26 = local read "Apply SP"() -> (w113:bool)
        n27 = local read "Abs. Move"() -> (w127:bool)
        n28 = case shown="True" w127 {
          tunnel: [w230 w232] -> w125
          tunnel: [w229 w231] -> w124
          tunnel: w122 -> [w230 w236]
          tunnel: w121 -> [w229 w235]
          frame False {
            n29 = local write "Abort Motion"(FALSE ("Abort Motion")) -> ()
          }
          frame True {
            n30 = flat-sequence {
              tunnel: w236 -> [w243]
              tunnel: w235 -> [w242]
              tunnel: [w241] -> w234
              tunnel: [w240] -> w233
              tunnel: w234 -> [w250]
              tunnel: w233 -> [w249]
              tunnel: [w250] -> w232
              tunnel: [w249] -> w231
              frame #0 {
                n31 = local read "New Motor Position"() -> (w246:i32)
                n32 = local read "Motor Position"() -> (w245:i32)
                n33 = local read "Maximum Motor Velocity"() -> (w247:u16)
                n34 = local write "Reference Velocity"(w247) -> ()
                n35 = Subtract(x=w246, y=w245) -> (x-y=w244:i32)
                n36 = local read "Abort Motion"() -> (w239:bool)
                n37 = call "MotorRelativeMove_new.vi"("stop"=w239, "error"=w242, "Maximum Velocity"=w247, "Motor Position Increment"=w244, "VISA resource name (in)"=w243) -> ("error in (no error) (output)"=w240:errorcluster, "VISA resource name (out)"=w241:refnum<visa-resource-name>, "motor position"=w238:i32, "effective velocity"=w237:i16)  [unwired: 3 in]
                n38 = local write "Motor Position"(w238) -> ()
                n39 = local write "Effective Velocity"(w237) -> ()
                n40 = local write "Error SMU"(w240) -> ()
              }
              frame #1 {
                n41 = local write "Abs. Move"(FALSE ("Abs. Move")) -> ()
              }
            }
          }
        }
        n42 = local read "Rel. Move"() -> (w126:bool)
        n43 = case shown="True" w126 {
          tunnel: w125 -> [w178 w187]
          tunnel: w124 -> [w179 w186]
          tunnel: [w178 w183] -> w116
          tunnel: [w179 w181] -> w117
          frame False {
            n44 = local write "Abort Motion"(FALSE ("Abort Motion")) -> ()
          }
          frame True {
            n45 = flat-sequence {
              tunnel: w186 -> [w189]
              tunnel: w187 -> [w190]
              tunnel: [w190] -> w185
              tunnel: [w189] -> w184
              tunnel: w185 -> [w203]
              tunnel: w184 -> [w202]
              tunnel: [w205] -> w182
              tunnel: [w200] -> w180
              tunnel: [w207] -> w183
              tunnel: w182 -> [w207]
              tunnel: [w206] -> w181
              tunnel: w180 -> [w206]
              frame #0 {
                n46 = local read "Relative Move Mode"() -> (w188:T8)
                n47 = case shown="\"Move by Motor Counts\", Default" w188 {
                  frame "Move by Motor Counts", Default {
                    n48 = local read "Motor Position Increment [counts]"() -> (w191:i32)
                    n49 = local read "Calibration Factor (#counts / nm)"() -> (w192:dbl)
                    n50 = Divide(x=w191, y=w192) -> (x/y=w193:dbl)
                    n51 = local write "Distance Increment [nm]"(w193) -> ()
                  }
                  frame "Move by Electrode Distance" {
                    n52 = local read "Calibration Factor (#counts / nm)"() -> (w195:dbl)
                    n53 = local read "Distance Increment [nm]"() -> (w196:dbl)
                    n54 = Multiply(x=w196, y=w195) -> (x*y=w194:dbl)
                    n55 = local write "Motor Position Increment [counts]"(w194) -> ()
                  }
                }
              }
              frame #1 {
                n56 = local read "Maximum Motor Velocity"() -> (w201:u16)
                n57 = local read "Motor Position Increment [counts]"() -> (w204:i32)
                n58 = local read "Abort Motion"() -> (w199:bool)
                n59 = local write "Reference Velocity"(w201) -> ()
                n60 = call "MotorRelativeMove_new.vi"("stop"=w199, "error"=w202, "Maximum Velocity"=w201, "Motor Position Increment"=w204, "VISA resource name (in)"=w203) -> ("error in (no error) (output)"=w200:errorcluster, "VISA resource name (out)"=w205:refnum<visa-resource-name>, "motor position"=w198:i32, "effective velocity"=w197:i16)  [unwired: 3 in]
                n61 = local write "Error SMU"(w200) -> ()
                n62 = local write "Motor Position"(w198) -> ()
                n63 = local write "Effective Velocity"(w197) -> ()
              }
              frame #2 {
                n64 = local write "Rel. Move"(FALSE ("Rel. Move")) -> ()
              }
            }
          }
        }
        n65 = case shown="True" w113 {
          tunnel: [w137 w144] -> w114
          tunnel: w117 -> [w137 w143]
          tunnel: w116 -> [w138 w142]
          tunnel: [w138 w141] -> w115
          frame False {
            n66 = local write "Apply SP"(FALSE) -> ()
          }
          frame True {
            n67 = flat-sequence {
              tunnel: w143 -> [w151]
              tunnel: w142 -> [w150]
              tunnel: [w152] -> w140
              tunnel: [w149] -> w139
              tunnel: [w154] -> w141
              tunnel: [w155] -> w144
              tunnel: w140 -> [w155]
              tunnel: w139 -> [w154]
              frame #0 {
                (unwired) "V%d"
                n68 = local read "Maximum Motor Velocity"() -> (w146:u16)
                n69 = Format Into String(w146) -> (resulting string=w145:string)  [unwired: 3 in, 1 out]
                n70 = Concatenate Strings("SP", w145) -> (w148:string)
                n71 = call "serial_write_read.vi"("error in (no error)"=w151, "command"=w148, "VISA resource name"=w150) -> ("error out"=w152:errorcluster, "VISA resource name out"=w149:refnum<visa-resource-name>)  [unwired: 6 in, 1 out]
                n72 = local write "Error MC"(w152) -> ()
              }
              frame #1 {
                n73 = local write "Apply SP"(FALSE) -> ()
              }
            }
          }
        }
        n74 = local read "Update Motor Position"() -> (w118:bool)
        n75 = case shown="True" w118 {
          tunnel: [w156 w162] -> w120
          tunnel: [w157 w163] -> w119
          tunnel: w115 -> [w157 w164]
          tunnel: w114 -> [w156 w161]
          frame False {
            n76 = local write "Update Motor Position"(FALSE ("Update Motor Position")) -> ()
          }
          frame True {
            n77 = flat-sequence {
              tunnel: w164 -> [w169]
              tunnel: w161 -> [w167]
              tunnel: [w172] -> w160
              tunnel: [w170] -> w159
              tunnel: [w175] -> w162
              tunnel: [w176] -> w163
              tunnel: w160 -> [w176]
              tunnel: w159 -> [w175]
              frame #0 {
                n78 = call "ReadMotorVelocity.vi"("VISA resource name (output) 2"=w169, "error in (no error) (output)"=w167) -> ("VISA resource name (output)"=w168:refnum<visa-resource-name>, "current velocity"=w166:i16, "error out"=w165:errorcluster)  [unwired: 1 in]
                n79 = local write "Effective Velocity"(w166) -> ()
                n80 = local write "Error SMU"(w165) -> ()
                n81 = call "ReadMotorPosition_new_thatec.vi"("VISA resource name (output) 2"=w168, "error in (no error) (output)"=w165) -> ("VISA resource name (output)"=w172:refnum<visa-resource-name>, "position"=w171:i32, "error out"=w170:errorcluster)  [unwired: 1 in]
                n82 = local write "Error SMU"(w170) -> ()
                n83 = local write "Motor Position"(w171) -> ()
              }
              frame #1 {
                n84 = local write "Update Motor Position"(FALSE ("Update Motor Position")) -> ()
                n85 = local read "Motor Position"() -> (w173:i32)
                n86 = local write "Delta MP"(w173) -> ()
              }
            }
          }
        }
        n87 = local read "Reset"() -> (w128:bool)
        n88 = case shown="True" w128 {
          tunnel: [w210 w214] -> w129
          tunnel: [w209 w212] -> w123
          tunnel: w119 -> [w210 w216]
          tunnel: w120 -> [w209 w215]
          frame False {
          }
          frame True {
            n89 = flat-sequence {
              tunnel: w216 -> [w223]
              tunnel: w215 -> [w222]
              tunnel: [w220] -> w213
              tunnel: [w217] -> w211
              tunnel: [w226] -> w214
              tunnel: w213 -> [w226]
              tunnel: [w225] -> w212
              tunnel: w211 -> [w225]
              frame #0 {
                # "define home position"
                n90 = call "serial_write_read.vi"("error in (no error)"=w222, "command"="HO" ("Inputstring"), "VISA resource name"=w223) -> ("error out"=w219:errorcluster, "VISA resource name out"=w221:refnum<visa-resource-name>)  [unwired: 6 in, 1 out]
                n91 = local write "Error SMU"(w219) -> ()
                n92 = call "ReadMotorPosition_new_thatec.vi"("VISA resource name (output) 2"=w221, "error in (no error) (output)"=w219) -> ("VISA resource name (output)"=w220:refnum<visa-resource-name>, "position"=w218:i32, "error out"=w217:errorcluster)  [unwired: 1 in]
                n93 = local write "Motor Position"(w218) -> ()
                n94 = local write "Error SMU"(w217) -> ()
              }
              frame #1 {
                n95 = local write "Reset"(FALSE ("Reset")) -> ()
              }
            }
          }
        }
        n96 = while {
          tunnel: w129 -> [w270]
          tunnel: w108 -> [w269]
          tunnel: [w268] -> w134
          tunnel: [w267] -> w133
          tunnel: [w266] -> w132
          tunnel: w109 -> [w265]
          tunnel: [w264] -> w131
          tunnel: w123 -> [w263]
          tunnel: w112 -> [w262]
          tunnel: w99 -> [w261]
          tunnel: w111 -> [w260]
          tunnel: w110 -> [w259]
          tunnel: [w258] -> w107
          tunnel: [w257] -> w106
          tunnel: [w256] -> w105
          tunnel: [w255] -> w104
          tunnel: w103 -> [w254]
          tunnel: w102 -> [w253]
          tunnel: [w252] -> w101
          tunnel: [w251] -> w100
          stop <- "Measurement" stop-if-true
          n97 = case shown="True" "Measurement" {
            tunnel: w270 -> [w280 w327]
            tunnel: w269 -> [w281 w326]
            tunnel: [w281 w324] -> w268
            tunnel: [w280 w321] -> w267
            tunnel: [w278 w320] -> w266
            tunnel: w265 -> [w279 w319]
            tunnel: [w279 w317] -> w264
            tunnel: w263 -> [w278 w316]
            tunnel: w262 -> [w275 w309]
            tunnel: w261 -> [w274 w308]
            tunnel: w260 -> [w276 w305]
            tunnel: w259 -> [w277 w304]
            tunnel: [w277 w297] -> w258
            tunnel: [w276 w296] -> w257
            tunnel: [w275 w295] -> w256
            tunnel: [w274 w294] -> w255
            tunnel: w254 -> [w272 w293]
            tunnel: w253 -> [w273 w292]
            tunnel: [w273 w287] -> w252
            tunnel: [w272 w286] -> w251
            frame False {
            }
            frame True {
              n98 = flat-sequence {
                tunnel: [w343] -> w315
                tunnel: [w342] -> w314
                tunnel: [w341] -> w313
                tunnel: [w340] -> w312
                tunnel: [w339] -> w310
                tunnel: [w338] -> w306
                tunnel: [w337] -> w303
                tunnel: [w336] -> w302
                tunnel: [w335] -> w291
                tunnel: [w334] -> w290
                tunnel: w292 -> [w334]
                tunnel: w293 -> [w335]
                tunnel: w304 -> [w336]
                tunnel: w305 -> [w337]
                tunnel: w308 -> [w338]
                tunnel: w309 -> [w339]
                tunnel: w316 -> [w340]
                tunnel: w319 -> [w341]
                tunnel: w326 -> [w342]
                tunnel: w327 -> [w343]
                tunnel: w315 -> [w396]
                tunnel: w314 -> [w344]
                tunnel: w313 -> [w345]
                tunnel: w312 -> [w395]
                tunnel: [w406] -> w311
                tunnel: w310 -> [w406]
                tunnel: [w405] -> w307
                tunnel: w306 -> [w405]
                tunnel: w303 -> [w404]
                tunnel: w302 -> [w403]
                tunnel: [w404] -> w301
                tunnel: [w403] -> w300
                tunnel: [w389] -> w299
                tunnel: [w390] -> w298
                tunnel: w291 -> [w400]
                tunnel: w290 -> [w399]
                tunnel: [w400] -> w289
                tunnel: [w399] -> w288
                tunnel: [w396] -> w285
                tunnel: [w395] -> w284
                tunnel: [w355] -> w283
                tunnel: [w354] -> w282
                tunnel: [w442] -> w325
                tunnel: [w441] -> w323
                tunnel: [w440] -> w322
                tunnel: [w439] -> w318
                tunnel: w311 -> [w438]
                tunnel: w307 -> [w437]
                tunnel: w301 -> [w435]
                tunnel: w300 -> [w436]
                tunnel: w299 -> [w434]
                tunnel: w298 -> [w433]
                tunnel: [w432] -> w297
                tunnel: [w431] -> w296
                tunnel: [w430] -> w295
                tunnel: [w429] -> w294
                tunnel: w289 -> [w428]
                tunnel: w288 -> [w427]
                tunnel: [w426] -> w287
                tunnel: [w425] -> w286
                tunnel: w285 -> [w422]
                tunnel: w284 -> [w421]
                tunnel: w283 -> [w423]
                tunnel: w282 -> [w418]
                tunnel: w325 -> [w1428]
                tunnel: [w1428] -> w324
                tunnel: w323 -> [w1433]
                tunnel: w322 -> [w1434]
                tunnel: [w1431] -> w321
                tunnel: [w1430] -> w320
                tunnel: w318 -> [w1429]
                tunnel: [w1429] -> w317
                frame #0 {
                  w332 = 0
                  # "Preparation of Variables"
                  n99 = local read "Motor Position"() -> (w330:i32)
                  n100 = local write "IV Sweep"(FALSE) -> ()
                  n101 = local write "Open / Close"(TRUE) -> ()
                  n102 = local write "delt MP Reached"(FALSE ("Delta MP Start Reached")) -> ()
                  n103 = local write "# IV Curves"(w332) -> ()
                  n104 = local write "# Data Points"(w332) -> ()
                  n105 = local write "Set Lockin"(TRUE) -> ()
                  n106 = local write "# O/C Cycles"(w332) -> ()
                  n107 = local write "Delta MP"(w330) -> ()
                }
                frame #1 {
                  (unwired) TRUE ("Enable Auto Range (T: Enable)")
                  w346 = u16 0 items=["DC Voltage", "AC Voltage", "2 - Wire Resistance", "4 - Wire Resistance", "DC Current", "AC Current", "Frequency", "Period", "Continuity", "Diode Checking", "VDC:VDC Ratio", "Temperature", "Capacitance"] ("Function (0: DC Voltage)")
                  # "Set Bias Voltage and Compliance Limit"
                  # "Enable Controller and Set Velocity"
                  # "Preparation of Devices"
                  n108 = local read "Use_femto"() -> (w353:bool)
                  n109 = case shown="True" w353 {
                    frame False {
                    }
                    frame True {
                      w415 = T1."10^3" ("Gain [V/A]")
                      n110 = call "Choose_Device.vi"("error in (no error)"=errorcluster {"status"=FALSE, "code"=0, "source"=""}, "Choose_Device"=Choose_Device_Enum."DLPCA-200", "Index"="Femto_Index") -> ("error out"=w411:errorcluster, "Device_type"=→"Femto status":T9, "Index_Out"=w408:i32)
                      n111 = call "Init_LUCI.vi"() -> ()  [unwired: 10 in, 2 out]
                      n112 = call "femto_selector_subvi.vi"("Femto_gain"=w415) -> ("y"=w414:dbl, "Gain  [V/A]"=w410:T6)  [unwired: 9 in]
                      n113 = call "Set_Gain_DLPCA-200_Alex.vi"("error in"=w411, "Status"=0, "Gain  [V/A]"=w410, "index"=w408) -> ("index_out"=w409:i32)  [unwired: 2 out]
                      n114 = local write "Femto_Index"(w409) -> ()
                      n115 = local write "CA gain"(w414) -> ()
                      "Femto_gain" <- w415
                    }
                  }
                  n116 = local read "LIA2_DMM_VISA"() -> (w382:refnum<visa-resource-name>)
                  n117 = local read "Bias Voltage OC"() -> (w347:dbl)
                  n118 = call <instrlib>:"Configure Measurement.vi"("Manual Range (1.00)"=w347, "error in (no error)"=w344, "Function (0: DC Voltage)"=w346, "VISA resource name"=w345) -> ("error out"=w348:errorcluster, "VISA resource name out"=w349:refnum<visa-resource-name>)  [unwired: 6 in]
                  n119 = local read "LIA1_DMM_VISA"() -> (w383:refnum<visa-resource-name>)
                  n120 = local read "DMM_6500_VISA"() -> (w365:refnum<visa-resource-name>)
                  n121 = call "Configure AC Filter.vi"("error in (no error)"=w348, "AC Filter Bandwidth (20 Hz)"="AC Filter", "VISA resource name"=w349) -> ("error out"=w385:errorcluster, "VISA resource name out"=w386:refnum<visa-resource-name>)  [unwired: 7 in]
                  n122 = call <instrlib>:"Configure Measurement.vi"("Manual Range (0)"="rang OC (V)", "Auto Range (T: Enable)"="Auto Range", "VISA resource name"=w365) -> ("error out"=w363:errorcluster, "VISA resource name out"=w364:refnum<visa-resource-name>)  [unwired: 7 in]
                  n123 = call "Configure Integration.vi"("error in (no error)"=w385, "Integration Time (1 PLCs)"="Int. Time", "VISA resource name"=w386) -> ("error out"=w354:errorcluster, "VISA resource name out"=w355:refnum<visa-resource-name>)  [unwired: 7 in]
                  n124 = call "Configure Voltage.vi"("Voltage Integration Time (10: 10)"="Int. Time", "Auto Impedance (F: Disable)"="AutoZ", "Voltage Bandwidth (20: 20 Hz)"="AC Filter", "VISA resource name"=w382) -> ("error out"=w360:errorcluster, "VISA resource name out"=w361:refnum<visa-resource-name>)  [unwired: 6 in]
                  n125 = call "Configure Voltage.vi"("Voltage Integration Time (10: 10)"="Int. Time", "Auto Impedance (F: Disable)"="AutoZ", "Voltage Bandwidth (20: 20 Hz)"="AC Filter", "VISA resource name"=w383) -> ("error out"=w358:errorcluster, "VISA resource name out"=w359:refnum<visa-resource-name>)  [unwired: 6 in]
                  n126 = call "Configure Voltage.vi"("VISA resource name"=w364, "Input Impedance (0: 10Mohm)"="Input Z", "error in (no error)"=w363) -> ("VISA resource name out"=w375:refnum<visa-resource-name>, "error out"=w374:errorcluster)  [unwired: 11 in]
                  n127 = call <instrlib>:"Configure Measurement.vi"("Manual Range (1)"="rang OC (V)", "error in (no error)"=w358, "Auto Range (T: Enable)"="Auto Range", "VISA resource name"=w359) -> ()  [unwired: 6 in, 2 out]
                  n128 = call <instrlib>:"Configure Measurement.vi"("Manual Range (1)"="rang OC (V)", "error in (no error)"=w360, "Auto Range (T: Enable)"="Auto Range", "VISA resource name"=w361) -> ()  [unwired: 6 in, 2 out]
                  n129 = call "Configure Line Synchronization.vi"("Enable Line Sync (F: Disable)"="Line Sync", "error in (no error)"=w374, "VISA resource name"=w375) -> ("error out"=w379:errorcluster, "VISA resource name out"=w380:refnum<visa-resource-name>)  [unwired: 7 in]
                  n130 = call "7651 Initialize.vi"("error in"=errorcluster {"status"=FALSE, "code"=0, "source"=""} ("Fehler (Eingang, kein Fehler)"), "VISA  name"="Yokogawa 7651") -> ("error out"=w387:errorcluster, "VISA  name"=w388:refnum<visa-resource-name>)  [unwired: 8 in]
                  n131 = call "Resistance_SMU.vi"("error in (no error)"=w379, "Display (0: Home Screen)"="Display", "VISA resource name"=w380) -> ("error out"=w376:errorcluster, "VISA resource name out"=w377:refnum<visa-resource-name>)  [unwired: 7 in]
                  n132 = call "7651 Set Range.vi"("error in"=w387, "Range"="Yoko_Range", "VISA  name"=w388) -> ("error out"=w397:errorcluster, "VISA  name"=w398:refnum<visa-resource-name>)  [unwired: 6 in, 1 out]
                  n133 = call "Configure NPLC.vi"("Power Line Cycle (1)"="Int. Time", "error in (no error)"=w376, "VISA resource name"=w377) -> ("error out"=w371:errorcluster, "VISA resource name out"=w372:refnum<visa-resource-name>)  [unwired: 7 in]
                  n134 = local read "Bias Voltage OC"() -> (w350:dbl)
                  n135 = call "Configure Average Filter.vi"("VISA resource name"=w372, "Count (10)"="F. Count", "Window (0)"="Fi. Window", "Enable Average Filter (F: Disable)"="Average F.", "error in (no error)"=w371, "Average Filter Type (0: Repeat)"="Av. F. Type") -> ()  [unwired: 8 in, 2 out]
                  n136 = call "7651 Set output val.vi"("error in"=w397, "Pol (T)"="Bias_polarity", "Val V /A (0)"=w350, "VISA  name"=w398) -> ("error out"=w391:errorcluster, "VISA  name"=w392:refnum<visa-resource-name>)  [unwired: 6 in]
                  n137 = local write "Bias_pol_inloop"("Bias_polarity") -> ()
                  n138 = local write "bias_in_loop"(w350) -> ()
                  n139 = call "7651 Set Limit.vi"("error in"=w391, "Limit Value"=100.0, "Mode"=enum16{"mA Limit", "V limit"}."mA Limit", "VISA  name"=w392) -> ("error out"=w390:errorcluster, "VISA  name"=w389:refnum<visa-resource-name>)  [unwired: 6 in]
                }
                frame #2 {
                  # "Measurement Loop"
                  n140 = Initialize Array(0.0 ("element"), "Array size") -> (w420:dbl[])
                  n141 = while {
                    tunnel: [w533] -> w441
                    tunnel: [w532] -> w440
                    tunnel: [w531] -> w442
                    tunnel: w423 -> [w530]
                    tunnel: [w529] -> w439
                    tunnel: w438 -> [w516]
                    tunnel: w437 -> [w515]
                    tunnel: w436 -> [w511]
                    tunnel: w435 -> [w510]
                    tunnel: w434 -> [w495]
                    tunnel: w433 -> [w494]
                    tunnel: [w493] -> w432
                    tunnel: [w492] -> w431
                    tunnel: [w491] -> w430
                    tunnel: [w490] -> w429
                    tunnel: w428 -> [w489]
                    tunnel: w427 -> [w488]
                    tunnel: [w445] -> w426
                    tunnel: [w446] -> w425
                    tunnel: w422 -> [w483]
                    tunnel: w421 -> [w482]
                    tunnel: "Array size" -> [w478]
                    shift-right: [w477] -> _
                    shift-left: w420 -> [w479]
                    tunnel: w418 -> [w451]
                    i -> [w547]
                    stop <- w539 stop-if-true
                    # "Check Abort Conditions"
                    # "Count Loops"
                    n142 = flat-sequence {
                      tunnel: w530 -> [w552]
                      tunnel: w451 -> [w572]
                      tunnel: [w552] -> w521
                      tunnel: [w572] -> w520
                      tunnel: w516 -> [w564]
                      tunnel: w515 -> [w571]
                      tunnel: [w564] -> w514
                      tunnel: [w571] -> w513
                      tunnel: w511 -> [w569]
                      tunnel: w510 -> [w570]
                      tunnel: [w570] -> w509
                      tunnel: [w569] -> w508
                      tunnel: [w563] -> w501
                      tunnel: [w562] -> w500
                      tunnel: w495 -> [w563]
                      tunnel: w494 -> [w562]
                      tunnel: w489 -> [w568]
                      tunnel: w488 -> [w567]
                      tunnel: [w568] -> w487
                      tunnel: [w567] -> w486
                      tunnel: w483 -> [w566]
                      tunnel: w482 -> [w565]
                      tunnel: [w566] -> w481
                      tunnel: [w565] -> w480
                      tunnel: w479 -> [w560]
                      tunnel: w478 -> [w555]
                      tunnel: [w587] -> w550
                      tunnel: w521 -> [w584]
                      tunnel: w520 -> [w583]
                      tunnel: [w584] -> w518
                      tunnel: [w583] -> w517
                      tunnel: w514 -> [w582]
                      tunnel: w513 -> [w581]
                      tunnel: [w581] -> w512
                      tunnel: w509 -> [w602]
                      tunnel: w508 -> [w600]
                      tunnel: [w601] -> w507
                      tunnel: [w599] -> w506
                      tunnel: w501 -> [w586]
                      tunnel: w500 -> [w585]
                      tunnel: [w586] -> w499
                      tunnel: [w585] -> w498
                      tunnel: w487 -> [w598]
                      tunnel: w486 -> [w597]
                      tunnel: [w596] -> w485
                      tunnel: [w595] -> w484
                      tunnel: w481 -> [w593]
                      tunnel: w480 -> [w592]
                      tunnel: [w588] -> w476
                      tunnel: [w582] -> w447
                      tunnel: [w581] -> w443
                      tunnel: w550 -> [w761]
                      tunnel: [w748] -> w475
                      tunnel: [w749] -> w473
                      tunnel: [w763] -> w471
                      tunnel: w518 -> [w732]
                      tunnel: w517 -> [w731]
                      tunnel: w512 -> [w757]
                      tunnel: w507 -> [w755]
                      tunnel: w506 -> [w754]
                      tunnel: [w760] -> w469
                      tunnel: [w759] -> w467
                      tunnel: [w736] -> w465
                      tunnel: [w758] -> w463
                      tunnel: w499 -> [w752]
                      tunnel: w498 -> [w753]
                      tunnel: [w753] -> w461
                      tunnel: [w752] -> w459
                      tunnel: w485 -> [w739]
                      tunnel: w484 -> [w738]
                      tunnel: w476 -> [w762]
                      tunnel: [w733] -> w456
                      tunnel: [w734] -> w455
                      tunnel: w447 -> [w756]
                      tunnel: [w729] -> w446
                      tunnel: [w728] -> w445
                      tunnel: [w723] -> w444
                      tunnel: w443 -> [w722]
                      tunnel: w475 -> [w1015]
                      tunnel: [w1015] -> w474
                      tunnel: w473 -> [w1014]
                      tunnel: [w1014] -> w472
                      tunnel: w471 -> [w1013]
                      tunnel: [w1013] -> w470
                      tunnel: w469 -> [w1012]
                      tunnel: [w1012] -> w468
                      tunnel: w467 -> [w1011]
                      tunnel: [w1011] -> w466
                      tunnel: w465 -> [w1010]
                      tunnel: [w1010] -> w464
                      tunnel: w463 -> [w1009]
                      tunnel: [w1009] -> w462
                      tunnel: w461 -> [w1008]
                      tunnel: [w1008] -> w460
                      tunnel: w459 -> [w1007]
                      tunnel: [w1007] -> w458
                      tunnel: [w1003] -> w457
                      tunnel: w456 -> [w1002]
                      tunnel: w455 -> [w1001]
                      tunnel: [w1000] -> w454
                      tunnel: [w999] -> w453
                      tunnel: [w995] -> w452
                      tunnel: [w993] -> w450
                      tunnel: [w994] -> w449
                      tunnel: w444 -> [w990]
                      tunnel: w474 -> [w1044]
                      tunnel: w472 -> [w1045]
                      tunnel: [w1043] -> w549
                      tunnel: [w1042] -> w548
                      tunnel: w470 -> [w1038]
                      tunnel: [w1031] -> w519
                      tunnel: w468 -> [w1034]
                      tunnel: w466 -> [w1035]
                      tunnel: w464 -> [w1037]
                      tunnel: w462 -> [w1036]
                      tunnel: [w1037] -> w505
                      tunnel: [w1036] -> w504
                      tunnel: [w1035] -> w503
                      tunnel: [w1034] -> w502
                      tunnel: [w1033] -> w497
                      tunnel: w460 -> [w1033]
                      tunnel: [w1032] -> w496
                      tunnel: w458 -> [w1032]
                      tunnel: w457 -> [w1029]
                      tunnel: w454 -> [w1031]
                      tunnel: w453 -> [w1024]
                      tunnel: w452 -> [w1028]
                      tunnel: w450 -> [w1027]
                      tunnel: w449 -> [w1026]
                      tunnel: [w1024] -> w448
                      tunnel: [w1180] -> w525
                      tunnel: [w1178] -> w524
                      tunnel: [w1177] -> w523
                      tunnel: [w1174] -> w522
                      tunnel: [w1162] -> w493
                      tunnel: [w1161] -> w492
                      tunnel: [w1160] -> w491
                      tunnel: [w1159] -> w490
                      tunnel: w496 -> [w1164]
                      tunnel: w497 -> [w1163]
                      tunnel: w502 -> [w1165]
                      tunnel: w503 -> [w1166]
                      tunnel: w504 -> [w1167]
                      tunnel: w505 -> [w1168]
                      tunnel: w519 -> [w1175]
                      tunnel: w548 -> [w1179]
                      tunnel: w549 -> [w1176]
                      tunnel: w448 -> [w1181]
                      tunnel: [w1392] -> w529
                      tunnel: [w1387] -> w532
                      tunnel: [w1389] -> w533
                      tunnel: [w1393] -> w531
                      tunnel: w525 -> [w1393]
                      tunnel: w524 -> [w1390]
                      tunnel: w523 -> [w1388]
                      tunnel: w522 -> [w1392]
                      frame #0 {
                        n143 = local read "# Data Points"() -> (w554:u32)
                        n144 = Quotient & Remainder(x=w554, y=w555) -> (x-y*floor(x/y)=w553:u32)  [unwired: 1 out]
                        n145 = local read "G in G0"() -> (w561:dbl)
                        n146 = Replace Array Subset(array=w560, new element=w561, index=w553) -> (w559:dbl[])
                        "cond array last 10" <- w559
                        n147 = call <vilib>:"Std Deviation and Variance.vi"("X"=w559) -> ("mean"=w557:dbl, "standard deviation"=w558:dbl)  [unwired: 1 in, 1 out]
                        n148 = Divide(x=w558, y=w557) -> (x/y=→"CV" →"CV 2":dbl)
                        n149 = local read "High -Low Resistance Velocity Mode"() -> (w573:bool)
                        n150 = case shown="True" w573 {
                          frame False {
                            n151 = local write "Low R Mode"(FALSE ("Low R Mode Active")) -> ()
                          }
                          frame True {
                            n152 = local read "Switch Res_Max. [Ohm]"() -> (w578:dbl)
                            n153 = local read "R [Ohm]"() -> (w580:dbl)
                            n154 = Absolute Value(x=w580) -> (abs(x)=w579:dbl)
                            n155 = Greater?(x=w579, y=w578) -> (0:→"High R mode":bool)
                            n156 = Less?(x=w579, y="switch Res Min [Ohm]") -> (x < y?=w576:bool)
                            n157 = local write "Low R Mode"(w576) -> ()
                          }
                        }
                      }
                      frame #1 {
                        # "Check if Direction Has to Be Reversed"
                        # "Check Misc Things"
                        n158 = local read "O/C Switch Mode"() -> (w594:T3)
                        n159 = case shown="\"Switch O/C by Delta MP\"" w594 {
                          tunnel: [w603 w637 w638] -> w589
                          frame "Switch O/C by Resistance", Default {
                            n160 = local read "Min. Resistance [Ohm]"() -> (w608:dbl)
                            n161 = local read "Max. Resistance [Ohm]"() -> (w607:dbl)
                            n162 = local read "Open / Close"() -> (w605:bool)
                            n163 = local read "R [Ohm]"() -> (w609:dbl)
                            n164 = call "ReverseCheck.vi"("Akt. Widerstand [Ohm]"=w609, "Min OC resistance [Ohm]"=w608, "MAX OC resistance [Ohm]"=w607, "Offset [Ohm]"=0.1, "Öffnen/Schließen"=w605) -> ("ReverseMotion"=w604:bool)
                            n165 = case shown="False" w604 {
                              tunnel: [w610 TRUE] -> w603
                              frame False {
                                n166 = local read "Switch by Motor Position Overrides other Switch Modes"() -> (w611:bool)
                                n167 = case shown="True" w611 {
                                tunnel: [FALSE w613] -> w610
                                frame False {
                                }
                                frame True {
                                n168 = local read "Max. Motor Position [counts]"() -> (w624:i32)
                                n169 = local read "Min. Motor Position [counts]"() -> (w622:i32)
                                n170 = local read "Motor Position"() -> (w621:i32)
                                n171 = local read "Motor Position"() -> (w623:i32)
                                n172 = local read "Open / Close"() -> (w616:bool)
                                n173 = local read "Open / Close"() -> (w614:bool)
                                n174 = Not(x=w616) -> (.not. x?=w615:bool)
                                n175 = Less?(x=w621, y=w622) -> (x < y?=w618:bool)
                                n176 = Greater?(x=w623, y=w624) -> (0:w620:bool)
                                n177 = And(x=w618, y=w614) -> (x .and. y?=w617:bool)
                                n178 = And(x=w620, y=w615) -> (x .and. y?=w619:bool)
                                n179 = Or(x=w617, y=w619) -> (x .or. y?=w613:bool)
                                }
                                }
                              }
                              frame True {
                              }
                            }
                          }
                          frame "Switch O/C by MP" {
                            n180 = local read "Max. Motor Position [counts]"() -> (w636:i32)
                            n181 = local read "Min. Motor Position [counts]"() -> (w634:i32)
                            n182 = local read "Motor Position"() -> (w633:i32)
                            n183 = local read "Motor Position"() -> (w635:i32)
                            n184 = local read "Open / Close"() -> (w628:bool)
                            n185 = local read "Open / Close"() -> (w626:bool)
                            n186 = Not(x=w628) -> (.not. x?=w627:bool)
                            n187 = Less?(x=w633, y=w634) -> (x < y?=w630:bool)
                            n188 = Greater?(x=w635, y=w636) -> (0:w632:bool)
                            n189 = And(x=w630, y=w626) -> (x .and. y?=w629:bool)
                            n190 = And(x=w632, y=w627) -> (x .and. y?=w631:bool)
                            n191 = Or(x=w629, y=w631) -> (x .or. y?=w637:bool)
                          }
                          frame "Switch O/C by Delta MP" {
                            n192 = local read "Open / Close"() -> (w640:bool)
                            n193 = case shown="True" w640 {
                              tunnel: [w645 w650] -> w639
                              frame False {
                                n194 = local read "Opening Start Resistance [Ohm]"() -> (w648:dbl)
                                n195 = local read "Min. R (Delta MP)  [Ohm]"() -> (w646:dbl)
                                n196 = local read "R [Ohm]"() -> (w644:dbl)
                                n197 = local read "R [Ohm]"() -> (w642:dbl)
                                n198 = Absolute Value(x=w644) -> (abs(x)=w643:dbl)
                                n199 = Absolute Value(x=w642) -> (abs(x)=w641:dbl)
                                n200 = Greater?(x=w643, y=w648) -> (0:w647:bool)
                                n201 = local write "delt MP Reached"(w647) -> ()
                                n202 = Less?(x=w641, y=w646) -> (x < y?=w645:bool)
                              }
                              frame True {
                                n203 = local read "delt MP Reached"() -> (w649:bool)
                                n204 = case shown="False" w649 {
                                tunnel: [FALSE w659] -> w650
                                frame False {
                                n205 = flat-sequence {
                                frame #0 {
                                n206 = local read "Opening Start Resistance [Ohm]"() -> (w655:dbl)
                                n207 = local read "R [Ohm]"() -> (w653:dbl)
                                n208 = Absolute Value(x=w653) -> (abs(x)=w652:dbl)
                                n209 = Greater?(x=w652, y=w655) -> (0:w654:bool)
                                n210 = local write "delt MP Reached"(w654) -> ()
                                }
                                frame #1 {
                                n211 = local read "delt MP Reached"() -> (w656:bool)
                                n212 = case shown="True" w656 {
                                frame False {
                                }
                                frame True {
                                n213 = local read "R [Ohm]"() -> (w658:dbl)
                                n214 = Absolute Value(x=w658) -> (abs(x)=w657:dbl)
                                n215 = local write "R [Ohm]"(w657) -> ()
                                }
                                }
                                }
                                }
                                }
                                frame True {
                                n216 = local read "Delta Motor Position [counts]"() -> (w661:i32)
                                n217 = local read "Delta MP"() -> (w662:T7)
                                n218 = local read "Motor Position"() -> (w663:i32)
                                n219 = Add(x=w662, y=w661) -> (x+y=w660:T7)
                                n220 = Less?(x=w663, y=w660) -> (x < y?=w659:bool)
                                }
                                }
                              }
                            }
                            n221 = case shown="False" w639 {
                              tunnel: [w664 TRUE] -> w638
                              frame False {
                                n222 = local read "Switch by Motor Position Overrides other Switch Modes"() -> (w665:bool)
                                n223 = case shown="True" w665 {
                                tunnel: [FALSE w667] -> w664
                                frame False {
                                }
                                frame True {
                                n224 = local read "Max. Motor Position [counts]"() -> (w678:i32)
                                n225 = local read "Min. Motor Position [counts]"() -> (w676:i32)
                                n226 = local read "Motor Position"() -> (w675:i32)
                                n227 = local read "Motor Position"() -> (w677:i32)
                                n228 = local read "Open / Close"() -> (w670:bool)
                                n229 = local read "Open / Close"() -> (w668:bool)
                                n230 = Not(x=w670) -> (.not. x?=w669:bool)
                                n231 = Less?(x=w675, y=w676) -> (x < y?=w672:bool)
                                n232 = Greater?(x=w677, y=w678) -> (0:w674:bool)
                                n233 = And(x=w672, y=w668) -> (x .and. y?=w671:bool)
                                n234 = And(x=w674, y=w669) -> (x .and. y?=w673:bool)
                                n235 = Or(x=w671, y=w673) -> (x .or. y?=w667:bool)
                                }
                                }
                              }
                              frame True {
                              }
                            }
                          }
                        }
                        n236 = Or(x="reverse direction", y=w589) -> (x .or. y?=w591:bool)
                        n237 = case shown="True" w591 {
                          tunnel: [w685 w690] -> w587
                          tunnel: w592 -> [w685 w687]
                          tunnel: w593 -> [w684 w688]
                          tunnel: w602 -> [w683 w699]
                          tunnel: [w683 w699] -> w601
                          tunnel: w600 -> [w682 w698]
                          tunnel: [w682 w698] -> w599
                          tunnel: w598 -> [w681 w697]
                          tunnel: w597 -> [w680 w696]
                          tunnel: [w681 w697] -> w596
                          tunnel: [w680 w696] -> w595
                          tunnel: [w684 w686] -> w588
                          frame False {
                          }
                          frame True {
                            n238 = local read "# O/C Cycles"() -> (w700:u16)
                            n239 = local read "Open / Close"() -> (w695:bool)
                            n240 = Increment(x=w700) -> (x+1=w701:u16)
                            n241 = local write "# O/C Cycles"(w701) -> ()
                            n242 = Not(x=w695) -> (.not. x?=w694:bool)
                            n243 = case shown="True" w694 {
                              tunnel: [w703 w713] -> w693
                              frame True {
                                # "opening"
                                n244 = local read "High R mode"() -> (w705:bool)
                                n245 = local read "Low R Mode"() -> (w706:bool)
                                n246 = Not(x=w706) -> (.not. x?=w704:bool)
                                n247 = And(x=w704, y=w705) -> (x .and. y?=w702:bool)
                                n248 = case shown="False" w706 {
                                tunnel: [w708 w711] -> w703
                                tunnel: w702 -> [w707 _]
                                frame False {
                                n249 = case shown="True" w707 {
                                tunnel: [w709 w710] -> w708
                                frame True {
                                n250 = local read "Opening Velocity (High R)"() -> (w709:i16)
                                }
                                frame False {
                                n251 = local read "Opening opening Vel"() -> (w710:i16)
                                }
                                }
                                }
                                frame True {
                                n252 = local read "Opening Velocity (Low R)"() -> (w711:i16)
                                }
                                }
                              }
                              frame False {
                                # "opening"
                                n253 = local read "High R mode"() -> (w715:bool)
                                n254 = local read "Low R Mode"() -> (w716:bool)
                                n255 = Not(x=w716) -> (.not. x?=w714:bool)
                                n256 = And(x=w714, y=w715) -> (x .and. y?=w712:bool)
                                n257 = case shown="False" w716 {
                                tunnel: [w718 w721] -> w713
                                tunnel: w712 -> [w717 _]
                                frame False {
                                n258 = case shown="False" w717 {
                                tunnel: [w719 w720] -> w718
                                frame True {
                                n259 = local read "Closing  Velocity (High R)"() -> (w719:i16)
                                }
                                frame False {
                                n260 = local read "Closing Vel"() -> (w720:i16)
                                }
                                }
                                }
                                frame True {
                                n261 = local read "Closing Velocity (Low R)"() -> (w721:i16)
                                }
                                }
                              }
                            }
                            n262 = local write "Reference Velocity"(w693) -> ()
                            n263 = Number To Decimal String(number=w693) -> (decimal integer string=w692:string)  [unwired: 1 in]
                            n264 = Concatenate Strings("V" ("string"), w692) -> (w689:string)
                            n265 = local write "Open / Close"(w694) -> ()
                            n266 = call "serial_write_read.vi"("error in (no error)"=w687, "command"=w689, "VISA resource name"=w688) -> ("error out"=w690:errorcluster, "VISA resource name out"=w686:refnum<visa-resource-name>)  [unwired: 6 in, 1 out]
                          }
                        }
                      }
                      frame #2 {
                        w744 = u16 1 items=["A", "B"] ("Input (0: A)")
                        w743 = u16 0 items=["A", "B"] ("Input (0: A)")
                        # "Acquire Data"
                        n267 = case shown="True" "Use_femto" {
                          tunnel: [FALSE w772] -> w723
                          tunnel: w722 -> [_ w771]
                          frame False {
                            "CA gain" <- "CA gain (man)"
                          }
                          frame True {
                            n268 = flat-sequence {
                              tunnel: [w786] -> w780
                              tunnel: [w783] -> w774
                              tunnel: w771 -> [w782]
                              tunnel: [w781] -> w769
                              tunnel: w780 -> [w804]
                              tunnel: [w791] -> w779
                              tunnel: [w788] -> w778
                              tunnel: [w795] -> w777
                              tunnel: ["amp_very_high_gain"] -> w776
                              tunnel: ["amp_very_low_gain"] -> w775
                              tunnel: w774 -> [w796]
                              tunnel: [w793] -> w773
                              tunnel: [w787] -> w770
                              tunnel: w769 -> [w787]
                              tunnel: w778 -> [w812]
                              tunnel: w779 -> [w813]
                              tunnel: w777 -> [w809]
                              tunnel: w776 -> [w811]
                              tunnel: w775 -> [w810]
                              tunnel: w773 -> [w808]
                              tunnel: [w807] -> w772
                              tunnel: w770 -> [w806]
                              frame #0 {
                                n269 = local read "Femto_Index"() -> (w784:i32)
                                n270 = local read "LIA_G"() -> (w783:bool)
                                n271 = call "Read._Overload.vi"("Index"=w784, "Choose_Device"=Choose_Device_Enum."DLPCA-200") -> ("Overload"=w786:bool)  [unwired: 1 in, 3 out]
                                "Overload" <- w786
                                n272 = call "LIA_overload_bool.vi"("VISA resource name"=w782) -> ("Overload? 2"=w781:bool)  [unwired: 2 in, 1 out]
                              }
                              frame #1 {
                                n273 = local read "Femto_gain"() -> (w795:T1)
                                n274 = local read "Volt drop"() -> (w802:dbl)
                                n275 = local read "LIA1_DMM"() -> (w805:dbl)
                                n276 = call "Femto_switch_conditions_new.vi"("Akt. LIA_1_Signal"=w805, "Min_LIA1_Signal"="Min_LIA1_Signal", "Overload"=w804, "LIA_G"=w796, "MAX LIA_1_Signal"="MAX LIA_1_Signal", "Akt_Vdrop_Signal"=w802, "Min_Vdrop_Signal"="Min_Vdrop_Signal", "MAX V_drop_Signal"="MAX V_drop_Signal") -> ("down"=w792:bool, "up"=w790:bool, "Activate_Femto"=w793:bool)  [unwired: 5 in]
                                "Activate_Femto" <- w793
                                n277 = local read "# Data Points"() -> (w794:u32)
                                n278 = call "even_int_bool.vi"("x"=w794) -> ("x = 0?"=w789:bool)  [unwired: 1 in]
                                n279 = And(x=w789, y=w790) -> (x .and. y?=w788:bool)
                                n280 = And(x=w789, y=w792) -> (x .and. y?=w791:bool)
                              }
                              frame #2 {
                                n281 = case shown="True" w808 {
                                tunnel: w813 -> [_ w826]
                                tunnel: w812 -> [_ w825]
                                tunnel: w809 -> [w816 w824]
                                tunnel: w811 -> [_ w822]
                                tunnel: w810 -> [_ w821]
                                tunnel: [FALSE w820] -> w807
                                tunnel: w806 -> [_ w819]
                                frame False {
                                n282 = call "femto_selector_subvi.vi"("Femto_gain"=w816) -> ("y"=w817:dbl, "Gain  [V/A]"=w814:T6)  [unwired: 9 in]
                                n283 = local read "Femto_Index"() -> (w818:i32)
                                n284 = local write "CA gain"(w817) -> ()
                                n285 = call "Set_Gain_DLPCA-200_Alex.vi"("Gain  [V/A]"=w814, "index"=w818) -> ()  [unwired: 2 in, 3 out]
                                }
                                frame True {
                                n286 = flat-sequence {
                                tunnel: w824 -> [w833]
                                tunnel: w825 -> [w832]
                                tunnel: w826 -> [w828]
                                tunnel: w819 -> [w829]
                                tunnel: [w841] -> w823
                                tunnel: w822 -> [w847]
                                tunnel: w821 -> [w844]
                                tunnel: w823 -> [w887]
                                tunnel: [w881] -> w820
                                frame #0 {
                                n287 = Or(x=w828, y=w829) -> (x .or. y?=w827:bool)
                                n288 = Not(x=w829) -> (.not. x?=w831:bool)
                                n289 = And(x=w831, y=w832) -> (x .and. y?=w830:bool)
                                n290 = case shown="True" w830 {
                                tunnel: w833 -> [_ w836]
                                frame False {
                                }
                                frame True {
                                n291 = call "Femto_selectror_up.vi"("max_gain  [V/A]"="max_gain", "Femto_gain"=w836) -> ("Gain [V/A]"=w835:u16)  [unwired: 9 in]
                                n292 = local write "Femto_gain"(w835) -> ()
                                }
                                }
                                n293 = case shown="True" w827 {
                                tunnel: w833 -> [_ w838]
                                frame False {
                                }
                                frame True {
                                n294 = call "Femto_selectror_down_other selector test.vi"("Femto_gain"=w838) -> ("Gain [V/A]"=w837:u16)  [unwired: 10 in]
                                n295 = local write "Femto_gain"(w837) -> ()
                                }
                                }
                                }
                                frame #1 {
                                n296 = local read "auto_amp_high_gain"() -> (w849:dbl)
                                n297 = local read "auto_amp_low_gain"() -> (w850:dbl)
                                n298 = local read "Femto_Index"() -> (w856:i32)
                                n299 = local read "Femto_gain"() -> (w841:T1)
                                n300 = Less?(x=w841, y="ampl. high_low_G") -> (x < y?=w845:bool)
                                n301 = Less?(x=w841, y="ampl. low_low_G") -> (x < y?=w846:bool)
                                n302 = Less?(x=w841, y="ampl. high_high_G") -> (x < y?=w843:bool)
                                n303 = call "Auto_gain_controller_4gains.vi"("auto_amp_low_gain"=w850, "_amp_high_gain"=w849, "_amp_very_high gain"=w847, "low/very_low_G"=w846, "high/very_high_G"=w843, "high/low_G"=w845, "very_low_gain"=w844) -> ("gain_out"=w848:dbl)  [unwired: 1 in]
                                n304 = case shown="False" "LIA2_internal" {
                                tunnel: w848 -> [w857 w869]
                                frame True {
                                w863 = u16 1 items=["External", "Internal"] ("Reference Source (1: Internal)")
                                w865 = u16 0 items=["External", "Internal"] ("Reference Source (1: Internal)")
                                # "low"
                                # "LIA_2_in_control"
                                n305 = local read "man phase LIA2"() -> (w861:dbl)
                                n306 = local read "Man Phase LIA1"() -> (w867:dbl)
                                n307 = local write "S OutpAmpl"(w857) -> ()
                                n308 = local read "Harm"() -> (w862:dbl)
                                n309 = local read "Auto Phase"() -> (w866:bool)
                                n310 = local read "Frequency"() -> (w859:dbl)
                                n311 = local read "VISA LIA1"() -> (w868:refnum<visa-resource-name>)
                                n312 = local read "VISA  LIA2"() -> (w860:refnum<visa-resource-name>)
                                n313 = local read "Auto Pha  LIA2"() -> (w864:bool)
                                n314 = local read "Ext  Trigger"() -> (w858:u16)
                                n315 = call "Configure Reference_external.vi"("VISA resource name"=w860, "Reference Source (1: Internal)"=w863, "Sine Output Amplitude (1 V)"=w857, "Detection Harmonic Number (1)"=w862, "Auto Phase (T: Enabled)"=w864, "Internal Reference Frequency (1000 Hz)"=w859, "Manual Phase (0 Degree)"=w861) -> ()  [unwired: 11 in, 2 out]
                                n316 = call "Configure Reference_external.vi"("VISA resource name"=w868, "Reference Source (1: Internal)"=w865, "Auto Phase (T: Enabled)"=w866, "Manual Phase (0 Degree)"=w867, "External Reference Trigger (0: Sine Zero Crossing)"=w858) -> ()  [unwired: 13 in, 2 out]
                                }
                                frame False {
                                w875 = u16 0 items=["External", "Internal"] ("Reference Source (1: Internal)")
                                w877 = u16 1 items=["External", "Internal"] ("Reference Source (1: Internal)")
                                # "LIA_1_in_control"
                                n317 = local read "man phase LIA2"() -> (w873:dbl)
                                n318 = local read "Man Phase LIA1"() -> (w879:dbl)
                                n319 = local read "Harm"() -> (w874:dbl)
                                n320 = local read "Auto Phase"() -> (w878:bool)
                                n321 = local read "Frequency"() -> (w870:dbl)
                                n322 = local read "VISA LIA1"() -> (w880:refnum<visa-resource-name>)
                                n323 = local write "S OutpAmpl"(w869) -> ()
                                n324 = local read "VISA  LIA2"() -> (w872:refnum<visa-resource-name>)
                                n325 = local read "Auto Pha  LIA2"() -> (w876:bool)
                                n326 = local read "Ext  Trigger"() -> (w871:u16)
                                n327 = call "Configure Reference_external.vi"("VISA resource name"=w872, "Reference Source (1: Internal)"=w875, "Detection Harmonic Number (1)"=w874, "Auto Phase (T: Enabled)"=w876, "Manual Phase (0 Degree)"=w873, "External Reference Trigger (0: Sine Zero Crossing)"=w871) -> ()  [unwired: 12 in, 2 out]
                                n328 = call "Configure Reference_external.vi"("VISA resource name"=w880, "Reference Source (1: Internal)"=w877, "Sine Output Amplitude (1 V)"=w869, "Auto Phase (T: Enabled)"=w878, "Internal Reference Frequency (1000 Hz)"=w870, "Manual Phase (0 Degree)"=w879) -> ()  [unwired: 12 in, 2 out]
                                }
                                }
                                n329 = call "femto_selector_subvi.vi"("Femto_gain"=w841) -> ("Gain  [V/A]"=w840:T6)  [unwired: 9 in, 1 out]
                                n330 = call "Set_Gain_DLPCA-200_Alex.vi"("Status"=0, "Gain  [V/A]"=w840, "index"=w856) -> ("Status_out"=→"Status_out":i32, "index_out"=→"index_out":i32)  [unwired: 1 in, 1 out]
                                }
                                frame #2 {
                                n331 = call "femto_selector_subvi.vi"("Femto_gain"=w887) -> ("y"=w883:dbl)  [unwired: 9 in, 1 out]
                                n332 = Greater?(x=w883, y=0.0001) -> (0:w886:bool)
                                n333 = Less?(x=w883, y=1e-10) -> (x < y?=w885:bool)
                                n334 = local write "CA gain"(w883) -> ()
                                n335 = Or(x=w885, y=w886) -> (x .or. y?=w881:bool)
                                n336 = case shown="True" w881 {
                                frame False {
                                n337 = Wait (ms)(milliseconds to wait="Range_switch_delay") -> ()  [unwired: 1 out]
                                }
                                frame True {
                                n338 = Wait (ms)(milliseconds to wait=u32 200) -> ()  [unwired: 1 out]
                                }
                                }
                                }
                                }
                                }
                                }
                              }
                            }
                          }
                        }
                        n339 = Or(x="Set Lockin", y="lockin_once") -> (x .or. y?=w725:bool)
                        n340 = case shown="True" w725 {
                          tunnel: [w908 w909] -> w760
                          tunnel: [w907 w910] -> w759
                          tunnel: [w906 w913] -> w736
                          tunnel: [w905 w914] -> w758
                          tunnel: w757 -> [w908 w979]
                          tunnel: w756 -> [w907 w976]
                          tunnel: w755 -> [w906 w973]
                          tunnel: w754 -> [w905 w970]
                          frame False {
                          }
                          frame True {
                            w911 = u16 4 items=["X"=1, "Y"=2, "R"=3, "Theta"=4, "Channel 1"=5, "Channel 2"=6, "Aux In 1"=7, "Aux In 2"=8, "Aux In 3"=9, "Aux In 4"=10] ("Parameter (1: X)")
                            n341 = local read "LIA2_internal"() -> (w922:bool)
                            n342 = call "Configure Sensitivity and Reserve.vi"("error in (no error)"=w970, "Sensitivity (-1: Auto gain)"="Sensitivity LIA2", "Dynamic Reserve (-1: Auto Reserve)"="Dyn Reserve  LIA2", "VISA resource name"=w973) -> ("error out"=w969:errorcluster, "VISA resource name out"=w972:refnum<visa-resource-name>)  [unwired: 6 in]
                            n343 = call "Configure Sensitivity and Reserve.vi"("error in (no error)"=w976, "Sensitivity (-1: Auto gain)"="Sensitivity LIA1", "Dynamic Reserve (-1: Auto Reserve)"="Dyn Reserve LIA1", "VISA resource name"=w979) -> ("error out"=w975:errorcluster, "VISA resource name out"=w978:refnum<visa-resource-name>)  [unwired: 6 in]
                            n344 = case shown="False" w922 {
                              tunnel: [w986 w988] -> w921
                              tunnel: [w985 w987] -> w920
                              frame True {
                                w986 = u16 1 items=["External", "Internal"] ("Reference Source (1: Internal)")
                                w985 = u16 0 items=["External", "Internal"] ("Reference Source (1: Internal)")
                              }
                              frame False {
                                w988 = u16 0 items=["External", "Internal"] ("Reference Source (1: Internal)")
                                w987 = u16 1 items=["External", "Internal"] ("Reference Source (1: Internal)")
                              }
                            }
                            n345 = call "Configure Filter.vi"("error in (no error)"=w969, "Low Pass Filter Slope (1: 12dB/oct)"="LP Slope LIA2", "Time Constant (8: 100ms)"="LP_timeLIA2", "VISA resource name"=w972) -> ("error out"=w968:errorcluster, "VISA resource name out"=w971:refnum<visa-resource-name>)  [unwired: 6 in]
                            n346 = call "Configure Filter.vi"("error in (no error)"=w975, "Low Pass Filter Slope (1: 12dB/oct)"="LP_slope_ LIA1", "Time Constant (8: 100ms)"="LP_timeLIA1", "VISA resource name"=w978) -> ("error out"=w974:errorcluster, "VISA resource name out"=w977:refnum<visa-resource-name>)  [unwired: 6 in]
                            n347 = call "Configure Reference_external.vi"("VISA resource name"=w971, "Reference Source (1: Internal)"=w921, "Sine Output Amplitude (1 V)"="S OutpAmpl", "Detection Harmonic Number (1)"="Harm", "error in (no error)"=w968, "Auto Phase (T: Enabled)"="Auto Pha  LIA2", "Internal Reference Frequency (1000 Hz)"="Frequency", "Manual Phase (0 Degree)"="man phase LIA2", "External Reference Trigger (0: Sine Zero Crossing)"="Ext  Trigger") -> ("VISA resource name out"=w949:refnum<visa-resource-name>, "error out"=w945:errorcluster)  [unwired: 9 in]
                            n348 = call "Configure Reference_external.vi"("VISA resource name"=w977, "Reference Source (1: Internal)"=w920, "Sine Output Amplitude (1 V)"="S OutpAmpl", "Detection Harmonic Number (1)"=1.0, "error in (no error)"=w974, "Auto Phase (T: Enabled)"="Auto Phase", "Internal Reference Frequency (1000 Hz)"="Frequency", "Manual Phase (0 Degree)"="Man Phase LIA1", "External Reference Trigger (0: Sine Zero Crossing)"="Ext  Trigger") -> ("VISA resource name out"=w952:refnum<visa-resource-name>, "error out"=w951:errorcluster)  [unwired: 9 in]
                            n349 = call "Configure Channel Expand and Offset.vi"("Auto Offset (F: Disable)"=FALSE, "error in (no error)"=w945, "Expand (0: x1)"="Expand LIA2", "VISA resource name"=w949) -> ("error out"=w947:errorcluster, "VISA resource name out"=w948:refnum<visa-resource-name>)  [unwired: 6 in]
                            n350 = call "Configure Channel Expand and Offset.vi"("Auto Offset (F: Disable)"=FALSE, "error in (no error)"=w951, "Expand (0: x1)"="Expand LIA1", "VISA resource name"=w952) -> ("VISA resource name out"=w950:refnum<visa-resource-name>)  [unwired: 6 in, 1 out]
                            n351 = call "Configure Acquisition.vi"("Continuous Storage (T: Enable)"="Cont Stor", "Sample Rate (0: 62.5 mHz)"="Sample Rate", "VISA resource name"=w950) -> ("error out"=w941:errorcluster, "VISA resource name out"=w942:refnum<visa-resource-name>)  [unwired: 7 in]
                            n352 = call "Configure Acquisition.vi"("Continuous Storage (T: Enable)"="Cont Stor", "error in (no error)"=w947, "Sample Rate (0: 62.5 mHz)"="Sample Rate", "VISA resource name"=w948) -> ("error out"=w939:errorcluster, "VISA resource name out"=w940:refnum<visa-resource-name>)  [unwired: 6 in]
                            n353 = call "Configure Input Signal.vi"("Input Notch Filter (0: None)"="Notch", "Input Shield Grounding (0: Float)"="Grounding", "error in (no error)"=w941, "Input Coupling (0: AC)"="In Coupling", "Input Connection (0: Single-Ended Voltage)"="Input", "VISA resource name"=w942) -> ("error out"=w925:errorcluster, "VISA resource name out"=w926:refnum<visa-resource-name>)  [unwired: 4 in]
                            n354 = call "Configure Input Signal.vi"("Input Notch Filter (0: None)"="Notch", "Input Shield Grounding (0: Float)"="Grounding", "error in (no error)"=w939, "Input Coupling (0: AC)"="In Coupling", "Input Connection (0: Single-Ended Voltage)"="Input", "VISA resource name"=w940) -> ("error out"=w931:errorcluster, "VISA resource name out"=w932:refnum<visa-resource-name>)  [unwired: 4 in]
                            n355 = call "Save Recall Setup.vi"("error in (no error)"=w931, "Setup Number (1)"="Setup Num", "Operation (0: Save)"="Save load", "VISA resource name"=w932) -> ("error out"=w929:errorcluster, "VISA resource name out"=w930:refnum<visa-resource-name>)  [unwired: 6 in]
                            n356 = call "Save Recall Setup.vi"("error in (no error)"=w925, "Setup Number (1)"="Setup Num", "Operation (0: Save)"="Save load", "VISA resource name"=w926) -> ("error out"=w927:errorcluster, "VISA resource name out"=w928:refnum<visa-resource-name>)  [unwired: 6 in]
                            n357 = call "Read X LIA.vi"("error in (no error)"=w929, "VISA resource name"=w930) -> ("error out"=w915:errorcluster, "Measurement"=→"X LIA 2":dbl, "VISA resource name out"=w916:refnum<visa-resource-name>)  [unwired: 7 in]
                            n358 = call "Read X LIA.vi"("error in (no error)"=w927, "VISA resource name"=w928) -> ("error out"=w918:errorcluster, "Measurement"=→"x LIA 1":dbl, "VISA resource name out"=w919:refnum<visa-resource-name>)  [unwired: 7 in]
                            n359 = call "Read X LIA.vi"("error in (no error)"=w915, "Parameter (1: X)"=w911, "VISA resource name"=w916) -> ("error out"=w914:errorcluster, "Measurement"=→"lia 2 phase":dbl, "VISA resource name out"=w913:refnum<visa-resource-name>)  [unwired: 6 in]
                            n360 = call "Read X LIA.vi"("error in (no error)"=w918, "Parameter (1: X)"=w911, "VISA resource name"=w919) -> ("error out"=w910:errorcluster, "Measurement"=→"phase_Lia1":dbl, "VISA resource name out"=w909:refnum<visa-resource-name>)  [unwired: 6 in]
                          }
                        }
                        n361 = call "Configure Instrument.vi"("VISA resource name"=w739, "error in (no error)"=w738) -> ("VISA resource name out"=w737:refnum<visa-resource-name>, "error out"=w745:errorcluster)  [unwired: 12 in]
                        n362 = call "Read Sensor_tempcontrollerB.vi"("VISA resource name"=w737, "Input (0: A)"=w743, "error in (no error)"=w745) -> ("VISA resource name out"=w741:refnum<visa-resource-name>, "Kelvin Reading"=→"Temp. A in K":dbl, "error out"=w742:errorcluster)  [unwired: 8 in, 2 out]
                        n363 = call "Read Sensor_tempcontrollerB.vi"("VISA resource name"=w741, "Input (0: A)"=w744, "error in (no error)"=w742) -> ("VISA resource name out"=w729:refnum<visa-resource-name>, "Kelvin Reading"=→"Temp B in K" →"sample Temperature":dbl, "error out"=w728:errorcluster)  [unwired: 8 in, 2 out]
                        n364 = case shown="True" "talk 34401" {
                          tunnel: [w890 w904] -> w734
                          tunnel: [w891 w896] -> w733
                          tunnel: w732 -> [w891 w901]
                          tunnel: w731 -> [w890 w903]
                          frame False {
                          }
                          frame True {
                            w900 = u16 0 items=["DC Voltage", "AC Voltage", "2 - Wire Resistance", "4 - Wire Resistance", "DC Current", "AC Current", "Frequency", "Period", "Continuity", "Diode Checking", "VDC:VDC Ratio", "Temperature", "Capacitance"] ("Function (0: DC Voltage)")
                            n365 = local read "Auto Range"() -> (w902:bool)
                            n366 = local read "rang OC (V)"() -> (w892:dbl)
                            n367 = call <instrlib>:"Configure Measurement.vi"("Manual Range (1.00)"=w892, "Manual Resolution (5.5 Digits)"="res 34401", "error in (no error)"=w903, "Enable Auto Range (T: Enable)"=w902, "Function (0: DC Voltage)"=w900, "VISA resource name"=w901) -> ("error out"=w904:errorcluster, "VISA resource name out"=w898:refnum<visa-resource-name>)  [unwired: 4 in]
                            n368 = VISA Write(VISA resource name=w898, write buffer="VOLTage:DC:RANGe?") -> (VISA resource name out=w897:refnum<visa-resource-name>)  [unwired: 1 in, 2 out]
                            n369 = VISA Read(VISA resource name=w897, byte count=u32 100) -> (VISA resource name out=w896:refnum<visa-resource-name>, read buffer=→"34401 range read":string)  [unwired: 1 in, 2 out]
                          }
                        }
                        n370 = call "serial_write_read.vi"("error in (no error)"=w761, "command"="POS", "VISA resource name"=w762) -> ("error out"=w748:errorcluster, "read buffer"=w751:string, "VISA resource name out"=w749:refnum<visa-resource-name>)  [unwired: 6 in]
                        n371 = call <vilib>:"Trim Whitespace.vi"("string"=w751) -> ("trimmed string"=w750:string)  [unwired: 1 in]
                        n372 = case shown="True" "Bias_set_in_loop" {
                          frame False {
                          }
                          frame True {
                            n373 = local read "Yokogawa 7651"() -> (w766:refnum<visa-resource-name>)
                            n374 = call "7651 Set output val.vi"("Pol (T)"="Bias_pol_inloop", "Val V /A (0)"="bias_in_loop", "VISA  name"=w766) -> ()  [unwired: 7 in, 2 out]
                          }
                        }
                        n375 = Decimal String To Number(string=w750) -> (number=w763:i32)  [unwired: 2 in, 1 out]
                        n376 = local write "Error MC"(w748) -> ()
                      }
                      frame #3 {
                        n377 = local read "DMM_6500_VISA"() -> (w1004:refnum<visa-resource-name>)
                        n378 = local read "# Data Points"() -> (w998:u32)
                        n379 = call "Read (Single Point).vi"("VISA resource name"=w1004) -> ("Measurement"=w1003:dbl)  [unwired: 12 in, 2 out]
                        "Volt drop" <- w1003
                        n380 = Quotient & Remainder(x=w998, y="wait bias") -> (x-y*floor(x/y)=w997:u32)  [unwired: 1 out]
                        n381 = local read "LIA1_DMM_VISA"() -> (w1005:refnum<visa-resource-name>)
                        n382 = local read "LIA2_DMM_VISA"() -> (w1006:refnum<visa-resource-name>)
                        n383 = call "Read (Single Point).vi"("VISA resource name"=w1006) -> ("Measurement"=w994:dbl)  [unwired: 8 in, 2 out]
                        "LIA2_DMM" <- w994
                        "LIA2_DMM_chart" <- w994
                        n384 = local read "Activate_Femto"() -> (w991:bool)
                        n385 = Not And(1:w990, 2:w991) -> (0:w989:bool)
                        n386 = case shown="True" w989 {
                          frame False {
                          }
                          frame True {
                            n387 = call "Time Delay"() -> ()  [unwired: 11 in, 1 out]
                          }
                        }
                        n388 = call "Read (Single Point).vi"("VISA resource name"=w1005) -> ("Measurement"=w993:dbl)  [unwired: 8 in, 2 out]
                        "LIA1_DMM" <- w993
                        "LIA1_DMM_chart" <- w993
                        n389 = Equal To 0?(x=w997) -> (x = 0?=w996:bool)
                        n390 = case shown="True" w996 {
                          tunnel: w1002 -> [w1017 w1023]
                          tunnel: w1001 -> [w1018 w1022]
                          tunnel: [w1017 w1021] -> w1000
                          tunnel: [w1018 w1020] -> w999
                          tunnel: [w1016 w1019] -> w995
                          frame False {
                            n391 = local read "Bias_meas"() -> (w1016:dbl)
                          }
                          frame True {
                            n392 = call "Read (Single Point).vi"("error in (no error)"=w1022, "VISA resource name"=w1023) -> ("error out"=w1020:errorcluster, "Measurement"=w1019:dbl, "VISA resource name out"=w1021:refnum<visa-resource-name>)  [unwired: 7 in]
                          }
                        }
                        "Bias_meas" <- w995
                      }
                      frame #4 {
                        n393 = local read "LIA_G"() -> (w1025:bool)
                        n394 = case shown="False" w1025 {
                          tunnel: w1038 -> [w1073 w1112]
                          tunnel: w1029 -> [w1066 w1104]
                          tunnel: w1028 -> [w1065 w1103]
                          tunnel: w1027 -> [w1048 w1089]
                          tunnel: w1026 -> [w1063 w1100]
                          frame True {
                            w1051 = "\t"
                            w1082 = FALSE
                            # "time    velocity     G     Vdrop       LIA_1      LIA_2   G_LIA1  Sens   Gain   ACamp   Temp"
                            # "Save Data to File and Display"
                            n395 = local read "CA gain"() -> (w1064:dbl)
                            n396 = local read "Pre-R [Ohm]"() -> (w1049:dbl)
                            n397 = call "Resistance_SMU.vi"("CA gain"=w1064, "Measurement Voltage"=w1065, "cable and pre-resistance"=w1049, "Input Value"=w1066) -> ("Output Resistance"=w1061:dbl, "Output conductance"=w1056:dbl)  [unwired: 6 in]
                            n398 = Less Than 0?(x=w1061) -> (x < 0?=w1067:bool)
                            n399 = case shown="True" w1067 {
                              tunnel: w1061 -> [w1083 w1085]
                              tunnel: [w1083 w1084] -> w1054
                              frame False {
                              }
                              frame True {
                                n400 = Multiply(x=w1085, y=-1.0) -> (x*y=w1084:dbl)
                              }
                            }
                            "R_Ohm_Vdrop" <- w1054
                            n401 = local read "Sensitivity"() -> (w1059:dbl)
                            n402 = local write "Sample Conductance (slave)"(w1056) -> ()
                            n403 = local read "Effective Velocity"() -> (w1068:i32)
                            n404 = local read "S OutpAmpl"() -> (w1057:dbl)
                            n405 = local read "Temp B in K"() -> (w1055:dbl)
                            n406 = local read "CA gain"() -> (w1058:dbl)
                            n407 = call "LIA1GG0-prefactor_corrected.vi"("LIA1_Sig"=w1048, "Expand"=1.0, "R_pre"=w1049, "AC amp"=w1057, "Sensitivity"=w1059, "CA gain"=w1058) -> ("G_[G_0]"=w1047:dbl, "LIA_all"=→"LIA_all":dbl)
                            n408 = local write "Sample Conductance (Main)"(w1047) -> ()
                            n409 = call "GinG0_to_R.vi"("G/G0_input"=w1047) -> ("R_Ohm_LIA1"=w1053:dbl)  [unwired: 2 in]
                            "R_Ohm_LIA1" <- w1053
                            n410 = local write "Resistance / time graph"(w1053) -> ()
                            n411 = local write "G in G0"(w1047) -> ()
                            n412 = local write "R [Ohm]"(w1053) -> ()
                            n413 = Number To Exponential String(number=w1073, 1:w1082) -> (E-format string=w1079:string)  [unwired: 2 in]
                            n414 = Number To Exponential String(number=w1047, 1:w1082) -> (E-format string=w1078:string)  [unwired: 2 in]
                            n415 = Number To Exponential String(number=w1061, 1:w1082) -> (E-format string=w1052:string)  [unwired: 2 in]
                            n416 = local read "Path Data Files"() -> (w1072:path)
                            n417 = local read "# O/C Cycles"() -> (w1075:u16)
                            n418 = Merge Signals(w1073, w1068, w1056, w1066, w1048, w1063, w1047, w1059, w1058, w1057, w1055) -> (w1081:dynamicdata)
                            n419 = local read "Label Filenames o/c/n"() -> (w1069:bool)
                            n420 = local read "Use Motor"() -> (w1070:bool)
                            n421 = local read "Open / Close"() -> (w1071:bool)
                            n422 = Number To Exponential String(number=0.0, 1:w1082) -> (E-format string=w1050:string)  [unwired: 2 in]
                            n423 = Concatenate Strings(w1079, w1051, w1078, w1051, w1052, w1051, w1050) -> (w1077:string)
                            n424 = local write "Acquired Data"(w1077) -> ()
                            n425 = call "Dateinamen_Nummerieren.vi"("Label Filenames"=w1069, "Use Motor"=w1070, "Open/Close"=w1071, "Breite"=3, "Nummer"=w1075, "Prefix"="G0", "Eingangspfad"=w1072) -> ("Ausgangspfad"=w1080:path)  [unwired: 2 in, 1 out]
                            n426 = call "LabVIEW-Messdaten in Datei schreiben"("File Name"=w1080, "Signals"=w1081) -> ()  [unwired: 7 in, 3 out]
                          }
                          frame False {
                            w1118 = ";"
                            w1124 = FALSE
                            # "time    velocity     G     Vdrop       LIA_1      LIA_2   G_LIA1  Sens   Gain   ACamp   Temp"
                            # "Save Data to File and Display"
                            n427 = local read "Pre-R [Ohm]"() -> (w1106:dbl)
                            n428 = local read "CA gain"() -> (w1102:dbl)
                            n429 = call "Resistance_SMU.vi"("CA gain"=w1102, "Measurement Voltage"=w1103, "cable and pre-resistance"=w1106, "Input Value"=w1104) -> ("Output Resistance"=w1098:dbl, "Output conductance"=w1092:dbl)  [unwired: 6 in]
                            n430 = Less Than 0?(x=w1098) -> (x < 0?=w1105:bool)
                            n431 = case shown="True" w1105 {
                              tunnel: w1098 -> [w1125 w1127]
                              tunnel: [w1125 w1126] -> w1101
                              frame False {
                              }
                              frame True {
                                n432 = Multiply(x=w1127, y=-1.0) -> (x*y=w1126:dbl)
                              }
                            }
                            n433 = local write "R [Ohm]"(w1101) -> ()
                            n434 = local read "Sensitivity"() -> (w1096:dbl)
                            n435 = local read "Pre-R [Ohm]"() -> (w1090:dbl)
                            n436 = local write "Sample Conductance (Main)"(w1092) -> ()
                            n437 = local read "S OutpAmpl"() -> (w1094:dbl)
                            n438 = call "GinG0_to_R.vi"("G/G0_input"=w1092) -> ("R_Ohm_LIA1"=w1091:dbl)  [unwired: 2 in]
                            n439 = local write "Resistance / time graph"(w1098) -> ()
                            n440 = local read "Effective Velocity"() -> (w1107:i32)
                            n441 = local read "CA gain"() -> (w1095:dbl)
                            n442 = call "LIA1GG0-prefactor_corrected.vi"("LIA1_Sig"=w1089, "Expand"=1.0, "R_pre"=w1090, "AC amp"=w1094, "Sensitivity"=w1096, "CA gain"=w1095) -> ("G_[G_0]"=w1088:dbl, "LIA_all"=w1087:dbl)
                            "Sample Conductance (slave)" <- w1088
                            "LIA_conductance" <- w1088
                            n443 = local write "R_Ohm_LIA1"(w1091) -> ()
                            n444 = local write "G in G0"(w1092) -> ()
                            n445 = local read "Temp B in K"() -> (w1093:dbl)
                            n446 = local read "Open / Close"() -> (w1110:bool)
                            n447 = local read "Path Data Files"() -> (w1111:path)
                            n448 = local write "LIA_all"(w1087) -> ()
                            n449 = local read "# O/C Cycles"() -> (w1114:u16)
                            n450 = Number To Exponential String(number=w1112, 1:w1124) -> (E-format string=w1121:string)  [unwired: 2 in]
                            n451 = Number To Exponential String(number=w1092, 1:w1124) -> (E-format string=w1120:string)  [unwired: 2 in]
                            n452 = Number To Exponential String(number=0.0, 1:w1124) -> (E-format string=w1119:string)  [unwired: 2 in]
                            n453 = Number To Exponential String(number=w1098, 1:w1124) -> (E-format string=w1117:string)  [unwired: 2 in]
                            n454 = local read "Label Filenames o/c/n"() -> (w1108:bool)
                            n455 = Merge Signals(w1112, w1107, w1092, w1104, w1089, w1100, w1088, w1096, w1095, w1094, w1093) -> (w1123:dynamicdata)
                            n456 = Concatenate Strings(w1121, w1118, w1120, w1118, w1119, w1118, w1117) -> (w1116:string)
                            n457 = local write "Acquired Data"(w1116) -> ()
                            n458 = local read "Use Motor"() -> (w1109:bool)
                            n459 = call "Current calc__Agilent _for IETS loop.vi"() -> ()  [unwired: 15 in, 1 out]
                            n460 = call "Dateinamen_Nummerieren.vi"("Label Filenames"=w1108, "Use Motor"=w1109, "Open/Close"=w1110, "Breite"=3, "Nummer"=w1114, "Prefix"="G0", "Eingangspfad"=w1111) -> ("Ausgangspfad"=w1122:path)  [unwired: 2 in, 1 out]
                            n461 = call "LabVIEW-Messdaten in Datei schreiben2"("File Name"=w1122, "Signals"=w1123) -> ()  [unwired: 7 in, 3 out]
                          }
                        }
                        n462 = local write "Motor Position"(w1038) -> ()
                        n463 = local read "# Data Points"() -> (w1041:u32)
                        n464 = Quotient & Remainder(x=w1041, y=1) -> (x-y*floor(x/y)=w1039:u32)  [unwired: 1 out]
                        n465 = Equal To 0?(x=w1039) -> (x = 0?=w1030:bool)
                        n466 = case shown="True" w1030 {
                          tunnel: w1045 -> [w1130 w1138]
                          tunnel: w1044 -> [w1129 w1137]
                          tunnel: [w1129 w1134] -> w1043
                          tunnel: [w1130 w1133] -> w1042
                          frame False {
                          }
                          frame True {
                            n467 = call "serial_write_read.vi"("error in (no error)"=w1137, "command"="GN", "VISA resource name"=w1138) -> ("error out"=w1134:errorcluster, "read buffer"=w1131:string, "VISA resource name out"=w1133:refnum<visa-resource-name>)  [unwired: 6 in]
                            n468 = local write "Error MC"(w1134) -> ()
                            n469 = call <vilib>:"Trim Whitespace.vi"("string"=w1131) -> ("trimmed string"=w1132:string)  [unwired: 1 in]
                            n470 = local write "Error MC"(w1134) -> ()
                            n471 = Decimal String To Number(string=w1132) -> (number=w1136:i32)  [unwired: 2 in, 1 out]
                            n472 = local write "Effective Velocity"(w1136) -> ()
                          }
                        }
                      }
                      frame #5 {
                        # "IETS-Loop"
                        n473 = local read "Temp B in K"() -> (w1148:dbl)
                        n474 = call "TimeStamp2013.vi"() -> ("LabVIEW TimeStamp"=→"LabVIEW\nTimeStamp":timestamp, "Date Formatted with Milliseconds"=w1139:string)  [unwired: 1 in]
                        n475 = local read "# Data Points"() -> (w1154:u32)
                        n476 = local read "IV Sweep"() -> (w1158:bool)
                        n477 = local read "wait points"() -> (w1155:i16)
                        n478 = local read "Max.  [Ohm]"() -> (w1173:dbl)
                        n479 = local read "Min.  [Ohm]"() -> (w1172:dbl)
                        n480 = local read "R [Ohm]"() -> (w1171:dbl)
                        n481 = local read "CV"() -> (w1152:dbl)
                        n482 = Quotient & Remainder(x=w1154, y=w1155) -> (x-y*floor(x/y)=w1153:u32)  [unwired: 1 out]
                        n483 = Less?(x=w1148, y="min_temp_limit") -> (x < y?=w1145:bool)
                        n484 = Equal To 0?(x=w1153) -> (x = 0?=w1156:bool)
                        n485 = Greater?(x=w1173, y=w1171) -> (0:w1170:bool)
                        n486 = Greater?(x=w1171, y=w1172) -> (0:w1169:bool)
                        n487 = Less?(x=w1152, y="CV _ Value") -> (x < y?=w1151:bool)
                        n488 = And(x=w1158, y=w1156) -> (x .and. y?=w1157:bool)
                        n489 = And(x=w1170, y=w1169) -> (x .and. y?=w1150:bool)
                        n490 = And(x=w1150, y=w1151) -> (x .and. y?=w1149:bool)
                        n491 = And(x=w1149, y=w1145) -> (x .and. y?=w1146:bool)
                        n492 = And(x=w1157, y=w1146) -> (x .and. y?=w1144:bool)
                        n493 = Or(x=w1144, y="IETS") -> (x .or. y?=w1141:bool)
                        n494 = local write "IV Active"(w1141) -> ()
                        n495 = case shown="True" w1141 {
                          tunnel: w1181 -> [w1189 w1229]
                          tunnel: [w1189 w1223] -> w1180
                          tunnel: [w1188 w1219] -> w1178
                          tunnel: w1179 -> [w1188 w1228]
                          tunnel: [w1187 w1224] -> w1177
                          tunnel: w1176 -> [w1187 w1227]
                          tunnel: w1175 -> [w1190 w1230]
                          tunnel: [w1190 w1215] -> w1174
                          tunnel: w1168 -> [w1185 w1212]
                          tunnel: w1167 -> [w1186 w1211]
                          tunnel: w1166 -> [w1184 w1210]
                          tunnel: w1165 -> [w1183 w1209]
                          tunnel: w1164 -> [_ w1204]
                          tunnel: w1163 -> [_ w1203]
                          tunnel: [w1186 w1201] -> w1162
                          tunnel: [w1185 w1200] -> w1161
                          tunnel: [w1184 w1199] -> w1160
                          tunnel: [w1183 w1198] -> w1159
                          tunnel: w1139 -> [_ w1191]
                          frame False {
                            "no IV" <- TRUE ("Boolean")
                          }
                          frame True {
                            n496 = local read "IV Delay [ms]"() -> (w1213:u16)
                            n497 = Wait (ms)(milliseconds to wait=w1213) -> ()  [unwired: 1 out]
                            n498 = flat-sequence {
                              tunnel: w1230 -> [w1238]
                              tunnel: w1229 -> [w1237]
                              tunnel: w1228 -> [w1243]
                              tunnel: w1227 -> [w1242]
                              tunnel: [w1240] -> w1226
                              tunnel: [w1239] -> w1225
                              tunnel: ["# IV  Loops"] -> w1218
                              tunnel: [w1238] -> w1216
                              tunnel: [w1237] -> w1214
                              tunnel: w1212 -> [w1233]
                              tunnel: w1211 -> [w1235]
                              tunnel: w1210 -> [w1236]
                              tunnel: w1209 -> [w1234]
                              tunnel: [w1234] -> w1208
                              tunnel: [w1236] -> w1207
                              tunnel: [w1233] -> w1206
                              tunnel: [w1235] -> w1205
                              tunnel: w1204 -> [w1231]
                              tunnel: w1203 -> [_]
                              tunnel: [w1231] -> w1202
                              tunnel: [w1234] -> w1197
                              tunnel: [w1233] -> w1196
                              tunnel: w1226 -> [w1259]
                              tunnel: w1225 -> [w1260]
                              tunnel: [w1258] -> w1222
                              tunnel: [w1256] -> w1221
                              tunnel: [w1255] -> w1220
                              tunnel: w1218 -> [w1246]
                              tunnel: [w1257] -> w1217
                              tunnel: w1216 -> [w1254]
                              tunnel: w1214 -> [w1253]
                              tunnel: w1208 -> [w1248]
                              tunnel: w1207 -> [w1249]
                              tunnel: w1206 -> [w1250]
                              tunnel: w1205 -> [w1251]
                              tunnel: w1202 -> [w1252]
                              tunnel: [w1251] -> w1201
                              tunnel: [w1250] -> w1200
                              tunnel: [w1249] -> w1199
                              tunnel: [w1248] -> w1198
                              tunnel: w1197 -> [w1245]
                              tunnel: w1196 -> [w1247]
                              tunnel: w1191 -> [w1244]
                              tunnel: w1217 -> [w1344]
                              tunnel: w1222 -> [w1343]
                              tunnel: w1221 -> [w1332]
                              tunnel: w1220 -> [w1329]
                              tunnel: [w1341] -> w1195
                              tunnel: [w1330] -> w1194
                              tunnel: [w1327] -> w1193
                              tunnel: [w1342] -> w1192
                              tunnel: [w1383] -> w1219
                              tunnel: [w1384] -> w1223
                              tunnel: [w1385] -> w1215
                              tunnel: [w1386] -> w1224
                              tunnel: w1195 -> [w1386]
                              tunnel: w1194 -> [w1385]
                              tunnel: w1193 -> [w1384]
                              tunnel: w1192 -> [w1383]
                              frame #0 {
                                n499 = call "serial_write_read.vi"("error in (no error)"=w1242, "command"="DI", "VISA resource name"=w1243) -> ("error out"=w1239:errorcluster, "VISA resource name out"=w1240:refnum<visa-resource-name>)  [unwired: 6 in, 1 out]
                                n500 = local write "Error MC"(w1239) -> ()
                              }
                              frame #1 {
                                n501 = for {
                                N: w1246 -> [_]
                                shift-right: [w1320] -> w1258
                                shift-left: w1260 -> [w1320]
                                shift-right: [w1321] -> w1257
                                shift-left: w1259 -> [w1321]
                                shift-right: [w1269] -> w1256
                                shift-left: w1254 -> [_]
                                shift-right: [w1293] -> w1255
                                shift-left: w1253 -> [w1293]
                                tunnel: w1252 -> [w1291]
                                tunnel: w1247 -> [w1287]
                                tunnel: w1245 -> [w1290]
                                tunnel: w1244 -> [w1264]
                                stop <- "?" stop-if-true
                                w1265 = "\t"
                                w1304 = 4
                                n502 = local read "R [Ohm]"() -> (w1280:dbl)
                                n503 = local read "G in G0"() -> (w1282:dbl)
                                n504 = local read "Bias Voltage OC"() -> (w1277:dbl)
                                n505 = local read "S OutpAmpl"() -> (w1288:dbl)
                                n506 = local read "CA gain"() -> (w1284:dbl)
                                n507 = local read "Man Phase LIA1"() -> (w1266:dbl)
                                n508 = local read "Pre-R [Ohm]"() -> (w1268:dbl)
                                n509 = local read "# IV Curves"() -> (w1305:u16)
                                n510 = local read "Open / Close"() -> (w1308:bool)
                                n511 = local read "Path Data Files"() -> (w1306:path)
                                n512 = local read "Label Filenames o/c/n"() -> (w1307:bool)
                                n513 = local read "Use Motor"() -> (w1303:bool)
                                n514 = Increment(x=w1305) -> (x+1=w1319:u16)
                                n515 = local write "# IV Curves"(w1319) -> ()
                                n516 = call "Dateinamen_Nummerieren.vi"("Label Filenames"=w1307, "Use Motor"=w1303, "Open/Close"=w1308, "Breite"=w1304, "Nummer"=w1305, "Prefix"="IETS", "Eingangspfad"=w1306) -> ("Ausgangspfad"=w1278:path)  [unwired: 2 in, 1 out]
                                n517 = local read "Temp B in K"() -> (w1263:dbl)
                                n518 = local read "Motor Position"() -> (w1302:i32)
                                n519 = local read "man phase LIA2"() -> (w1317:dbl)
                                n520 = local read "S OutpAmpl"() -> (w1298:dbl)
                                n521 = local read "LP_timeLIA1"() -> (w1301:u16)
                                n522 = local read "# O/C Cycles"() -> (w1325:u16)
                                n523 = local read "# Data Points"() -> (w1326:u32)
                                n524 = local read "Volt drop"() -> (w1296:dbl)
                                n525 = call "Dateinamen_Nummerieren.vi"("Label Filenames"=w1307, "Use Motor"=w1303, "Open/Close"=w1308, "Breite"=w1304, "Nummer"=w1305, "Prefix"="upsweep", "Eingangspfad"=w1306) -> ("Ausgangspfad"=w1285:path)  [unwired: 2 in, 1 out]
                                n526 = Number To Decimal String(number=w1317) -> (decimal integer string=w1314:string)  [unwired: 1 in]
                                n527 = Number To Decimal String(number=w1326) -> (decimal integer string=w1324:string)  [unwired: 1 in]
                                n528 = Number To Decimal String(number=w1325) -> (decimal integer string=w1323:string)  [unwired: 1 in]
                                n529 = Number To Decimal String(number=w1302) -> (decimal integer string=w1322:string)  [unwired: 1 in]
                                n530 = call "format into string.vi"("float"=w1263) -> ("resulting string"=w1262:string)  [unwired: 1 in]
                                n531 = Multiply(x=w1296, y=1000.0 ("x")) -> (x*y=w1294:dbl)
                                n532 = local read "LP_timeLIA2"() -> (w1311:u16)
                                n533 = Number To Decimal String(number=w1294) -> (decimal integer string=w1313:string)  [unwired: 1 in]
                                n534 = Multiply(x=10.0, y=w1298) -> (x*y=w1297:dbl)
                                n535 = call "Dateinamen_Nummerieren.vi"("Label Filenames"=w1307, "Use Motor"=w1303, "Open/Close"=w1308, "Breite"=w1304, "Nummer"=w1305, "Prefix"="downsweep", "Eingangspfad"=w1306) -> ("Ausgangspfad"=w1286:path)  [unwired: 2 in, 1 out]
                                n536 = Number To Decimal String(number=w1297) -> (decimal integer string=w1312:string)  [unwired: 1 in]
                                n537 = Number To Decimal String(number=w1311) -> (decimal integer string=w1267:string)  [unwired: 1 in]
                                n538 = Number To Decimal String(number=w1301) -> (decimal integer string=w1300:string)  [unwired: 1 in]
                                n539 = Concatenate Strings("Data_Points   O/C_Cyles  Motor_Pos  lockin_phase  Temperature Voltage_drop LockAmpl timeLIA1 timeLIA2   OC_timestamp ", "\r", w1324, w1265, w1323, w1265, w1322, w1265, w1314, w1265, w1262, w1265, w1313, w1265, w1312, w1265, w1300, w1265, w1267, w1265, w1264, w1265) -> (w1281:string)
                                n540 = call "IETS_sweep routine_2021_subvis.vi"("Yokogawa 7651"=w1291, "LIA1"=w1290, "Sens_LIA 1"="Sensitivity", "AC amp"=w1288, "LIA2"=w1287, "file path 3"=w1286, "pre-resistance"=w1268, "file path 2"=w1285, "Initail V"="Initail V", "CA gain"=w1284, "LIA exp 2"="LIA exp 2", "Step (V)"="Step (V)", "Sensitivity 2"="Sensitivity 2", "Set0 step (V)"="Set0 step", "Final V"="Final V", "bias_in"=w1277, "Lia1_pase"=w1266, "file path"=w1278, "LIA exp 1"="LIA exp 1", "Resistance"=w1280, "motor-info"=w1281, "Cond (G0)"=w1282) -> ("allchart_lia2"=→"?":cluster{"x":dbl, "y":dbl}[], "VISA Agilent out"=w1269:refnum<visa-resource-name>, "IV_allchart"=→"XY Graph   4":cluster{"x":dbl, "y":dbl}[], "allchart_Lia1"=→"XY Graph   3":cluster{"X":dbl, "Y":dbl}[])  [unwired: 2 in]
                                n541 = local write "IV Comment"(w1281) -> ()
                                }
                              }
                              frame #2 {
                                w1333 = u16 0 items=["DC Voltage", "AC Voltage", "2 - Wire Resistance", "4 - Wire Resistance", "DC Current", "AC Current", "Frequency", "Period", "Continuity", "Diode Checking", "VDC:VDC Ratio", "Temperature", "Capacitance"] ("Function (0: DC Voltage)")
                                n542 = local read "LIA2_DMM_VISA"() -> (w1337:refnum<visa-resource-name>)
                                n543 = local read "DMM_6500_VISA"() -> (w1338:refnum<visa-resource-name>)
                                n544 = local read "Int. Time"() -> (w1339:dbl)
                                n545 = local read "LIA1_DMM_VISA"() -> (w1336:refnum<visa-resource-name>)
                                n546 = local read "Use Motor"() -> (w1340:bool)
                                n547 = case shown="True" w1340 {
                                tunnel: w1344 -> [w1349 w1360]
                                tunnel: w1343 -> [w1347 w1359]
                                tunnel: [w1348 w1357] -> w1342
                                tunnel: [w1346 w1355] -> w1341
                                frame False {
                                n548 = call "serial_write_read.vi"("error in (no error)"=w1347, "command"="DI", "VISA resource name"=w1349) -> ("error out"=w1346:errorcluster, "VISA resource name out"=w1348:refnum<visa-resource-name>)  [unwired: 6 in, 1 out]
                                }
                                frame True {
                                (unwired) "V%d"
                                n549 = local read "Open / Close"() -> (w1352:bool)
                                n550 = case shown="False" w1352 {
                                tunnel: [w1366 w1376] -> w1351
                                frame True {
                                n551 = local read "Low R Mode"() -> (w1365:bool)
                                n552 = local read "High R mode"() -> (w1363:bool)
                                n553 = Not(x=w1365) -> (.not. x?=w1364:bool)
                                n554 = And(x=w1364, y=w1363) -> (x .and. y?=w1362:bool)
                                n555 = case shown="False" w1365 {
                                tunnel: [w1368 w1371] -> w1366
                                tunnel: w1362 -> [w1367 _]
                                frame False {
                                n556 = case shown="False" w1367 {
                                tunnel: [w1369 w1370] -> w1368
                                frame False {
                                n557 = local read "Opening opening Vel"() -> (w1369:i16)
                                }
                                frame True {
                                n558 = local read "Opening Velocity (High R)"() -> (w1370:i16)
                                }
                                }
                                }
                                frame True {
                                n559 = local read "Opening Velocity (Low R)"() -> (w1371:i16)
                                }
                                }
                                }
                                frame False {
                                n560 = local read "Low R Mode"() -> (w1375:bool)
                                n561 = local read "High R mode"() -> (w1373:bool)
                                n562 = Not(x=w1375) -> (.not. x?=w1374:bool)
                                n563 = And(x=w1374, y=w1373) -> (x .and. y?=w1372:bool)
                                n564 = case shown="False" w1375 {
                                tunnel: [w1378 w1381] -> w1376
                                tunnel: w1372 -> [w1377 _]
                                frame False {
                                n565 = case shown="True" w1377 {
                                tunnel: [w1379 w1380] -> w1378
                                frame False {
                                n566 = local read "Closing Vel"() -> (w1379:i16)
                                }
                                frame True {
                                n567 = local read "Closing  Velocity (High R)"() -> (w1380:i16)
                                }
                                }
                                }
                                frame True {
                                n568 = local read "Closing Velocity (Low R)"() -> (w1381:i16)
                                }
                                }
                                }
                                }
                                n569 = local write "Reference Velocity"(w1351) -> ()
                                n570 = call "serial_write_read.vi"("error in (no error)"=w1359, "command"="EN", "VISA resource name"=w1360) -> ("error out"=w1356:errorcluster, "VISA resource name out"=w1358:refnum<visa-resource-name>)  [unwired: 6 in, 1 out]
                                n571 = local write "Error MC"(w1356) -> ()
                                n572 = Format Into String(w1351) -> (resulting string=w1350:string)  [unwired: 3 in, 1 out]
                                n573 = Concatenate Strings("V", w1350) -> (w1353:string)
                                n574 = call "serial_write_read.vi"("error in (no error)"=w1356, "command"=w1353, "VISA resource name"=w1358) -> ("error out"=w1355:errorcluster, "VISA resource name out"=w1357:refnum<visa-resource-name>)  [unwired: 6 in, 1 out]
                                n575 = local write "Error MC"(w1355) -> ()
                                }
                                }
                                n576 = call "Configure Voltage.vi"("Voltage Integration Time (10: 10)"=w1339, "VISA resource name"=w1336) -> ()  [unwired: 8 in, 2 out]
                                n577 = call "Configure Voltage.vi"("Voltage Integration Time (10: 10)"=w1339, "VISA resource name"=w1337) -> ()  [unwired: 8 in, 2 out]
                                n578 = call "Configure NPLC.vi"("Power Line Cycle (1)"=w1339, "VISA resource name"=w1338) -> ()  [unwired: 8 in, 2 out]
                                n579 = local read "Bias Voltage OC"() -> (w1335:dbl)
                                n580 = call <instrlib>:"Configure Measurement.vi"("Manual Range (1.00)"=w1335, "error in (no error)"=w1329, "Enable Auto Range (T: Enable)"=FALSE, "Function (0: DC Voltage)"=w1333, "VISA resource name"=w1332) -> ("error out"=w1328:errorcluster, "VISA resource name out"=w1331:refnum<visa-resource-name>)  [unwired: 5 in]
                                n581 = call "Configure Integration.vi"("error in (no error)"=w1328, "Integration Time (1 PLCs)"=w1339, "VISA resource name"=w1331) -> ("error out"=w1327:errorcluster, "VISA resource name out"=w1330:refnum<visa-resource-name>)  [unwired: 7 in]
                              }
                              frame #3 {
                                n582 = Wait (ms)(milliseconds to wait=u32 100) -> ()  [unwired: 1 out]
                              }
                            }
                          }
                        }
                      }
                      frame #6 {
                        n583 = local read "Use Motor"() -> (w1391:bool)
                        n584 = case shown="True" w1391 {
                          tunnel: w1390 -> [w1395 w1406]
                          tunnel: [w1395 w1404] -> w1389
                          tunnel: [w1394 w1402] -> w1387
                          tunnel: w1388 -> [w1394 w1398]
                          frame False {
                          }
                          frame True {
                            (unwired) "V%d"
                            n585 = call "serial_write_read.vi"("error in (no error)"=w1398, "command"="EN", "VISA resource name"=w1406) -> ("error out"=w1403:errorcluster, "VISA resource name out"=w1405:refnum<visa-resource-name>)  [unwired: 6 in, 1 out]
                            n586 = local read "Open / Close"() -> (w1399:bool)
                            n587 = case shown="True" w1399 {
                              tunnel: [w1412 w1422] -> w1396
                              frame True {
                                n588 = local read "Low R Mode"() -> (w1411:bool)
                                n589 = local read "High R mode"() -> (w1409:bool)
                                n590 = Not(x=w1411) -> (.not. x?=w1410:bool)
                                n591 = And(x=w1410, y=w1409) -> (x .and. y?=w1408:bool)
                                n592 = case shown="False" w1411 {
                                tunnel: [w1414 w1417] -> w1412
                                tunnel: w1408 -> [w1413 _]
                                frame False {
                                n593 = case shown="True" w1413 {
                                tunnel: [w1415 w1416] -> w1414
                                frame True {
                                n594 = local read "Opening Velocity (High R)"() -> (w1415:i16)
                                }
                                frame False {
                                n595 = local read "Opening opening Vel"() -> (w1416:i16)
                                }
                                }
                                }
                                frame True {
                                n596 = local read "Opening Velocity (Low R)"() -> (w1417:i16)
                                }
                                }
                              }
                              frame False {
                                n597 = local read "Low R Mode"() -> (w1421:bool)
                                n598 = local read "High R mode"() -> (w1419:bool)
                                n599 = Not(x=w1421) -> (.not. x?=w1420:bool)
                                n600 = And(x=w1420, y=w1419) -> (x .and. y?=w1418:bool)
                                n601 = case shown="False" w1421 {
                                tunnel: [w1424 w1427] -> w1422
                                tunnel: w1418 -> [w1423 _]
                                frame False {
                                n602 = case shown="True" w1423 {
                                tunnel: [w1425 w1426] -> w1424
                                frame True {
                                n603 = local read "Closing  Velocity (High R)"() -> (w1425:i16)
                                }
                                frame False {
                                n604 = local read "Closing Vel"() -> (w1426:i16)
                                }
                                }
                                }
                                frame True {
                                n605 = local read "Closing Velocity (Low R)"() -> (w1427:i16)
                                }
                                }
                              }
                            }
                            n606 = local write "Error MC"(w1403) -> ()
                            n607 = local write "Reference Velocity"(w1396) -> ()
                            n608 = Format Into String(w1396) -> (resulting string=w1397:string)  [unwired: 3 in, 1 out]
                            n609 = Concatenate Strings("V", w1397) -> (w1400:string)
                            n610 = call "serial_write_read.vi"("error in (no error)"=w1403, "command"=w1400, "VISA resource name"=w1405) -> ("error out"=w1402:errorcluster, "VISA resource name out"=w1404:refnum<visa-resource-name>)  [unwired: 6 in, 1 out]
                            n611 = local write "Error MC"(w1402) -> ()
                          }
                        }
                      }
                    }
                    n612 = local read "Minimum Limit [counts]"() -> (w545:i32)
                    n613 = local read "Maximum Limit [counts]"() -> (w544:i32)
                    n614 = local read "Motor Position"() -> (w543:i32)
                    n615 = local read "Measurement"() -> (w546:bool)
                    n616 = local read "Stop"() -> (w535:bool)
                    n617 = local read "R [Ohm]"() -> (w542:dbl)
                    n618 = local read "# Errors"() -> (w528:u16)
                    n619 = Not(x=w546) -> (.not. x?=w534:bool)
                    n620 = Absolute Value(x=w542) -> (abs(x)=w541:dbl)
                    n621 = Greater?(x=w528, y=25) -> (0:w526:bool)
                    n622 = Less?(x=w543, y=w545) -> (x < y?=w538:bool)
                    n623 = Greater?(x=w543, y=w544) -> (0:w537:bool)
                    n624 = Less?(x=w541, y=1) -> (x < y?=w536:bool)
                    n625 = Compound Arithmetic op=OR(w538, w537, w536, w535, w534, w526) -> (w539:bool)
                    n626 = local read "cond array last 10"() -> (w477:dbl[])
                    n627 = local write "# Data Points"(w547) -> ()
                    n628 = case shown="True" w539 {
                      frame False {
                      }
                      frame True {
                        n629 = local write "Measurement"(FALSE) -> ()
                      }
                    }
                  }
                }
                frame #3 {
                  # "Turn off Devices"
                  n630 = call "serial_write_read.vi"("error in (no error)"=w1434, "command"="DI", "VISA resource name"=w1433) -> ("error out"=w1430:errorcluster, "VISA resource name out"=w1431:refnum<visa-resource-name>)  [unwired: 6 in, 1 out]
                  n631 = local write "Error MC"(w1430) -> ()
                }
              }
            }
          }
        }
        n632 = Not(x="Stop") -> (.not. x?=w135:bool)
      }
    }
    frame #2 {
      # "Close VISA"
      # "Switch off Motor"
      # "Finalization"
      n633 = VISA Close(VISA resource name=w1441, error in (no error)=w1440) -> (error out=→"Error SMU":errorcluster)
      n634 = call "serial_write_read.vi"("error in (no error)"=w1446, "command"="DI", "VISA resource name"=w1447) -> ("error out"=w1443:errorcluster, "VISA resource name out"=w1445:refnum<visa-resource-name>)  [unwired: 6 in, 1 out]
      n635 = local write "Error MC"(w1443) -> ()
      n636 = call "Close.vi"("error in (no error)"=w1436, "VISA resource name"=w1435) -> ()  [unwired: 9 in, 1 out]
      n637 = call "Close.vi"("error in (no error)"=w1438, "VISA resource name"=w1437) -> ()  [unwired: 9 in, 1 out]
      n638 = VISA Close(VISA resource name=w1445, error in (no error)=w1443) -> (error out=→"Error MC":errorcluster)
    }
  }
  n639 = call "Close.vi"("VISA resource name"=w2, "error in (no error)"=w1) -> ()  [unwired: 13 in, 1 out]
